vi "DOE Washer SM.vi"() -> ()   [LabVIEW 2018]
uses:
  Utility/Custom Pallet Controls/Custom Pallet Timer.ctl
  Type Definitions/DOE Front Panel Meters.ctl
  Utility/Type Definitions/UTILITY Power Data.ctl
  Utility/Standby Power/Type Definitions/Standby Power Main Data.ctl
  Drivers/Omega FMA-1600A Series Gas Flow Meter/Type Definitions/FMA1600A Gas Data.ctl
  Drivers/Omega FMA-1600A Series Gas Flow Meter/Type Definitions/FMA1600A Gas Type.ctl
  Range/Type Definitions/RANGE Meter Selector 1-2.ctl
  Utility/Save File/File Setup (Public)/Type Definition/Save File DOE File Path Control.ctl
  Utility/Save File/File Setup (Public)/Type Definition/Save File DOE Data Save Filepaths.ctl
  Type Definitions/DOE Main Control.ctl
  Type Definitions/DOE Test Fixture Hardware.ctl
  Utility/Type Definitions/UTILITY Power Inputs Control.ctl
  Drivers/IND560 Scale Monitor/Type Definitions/IND560 Configuration.ctl
  Hybrid Water Heater/Type Definitions/HEWH Agilent Cluster.ctl
  Utility/Type Definitions/UTILITY TC Coefficients.ctl
  Drivers/Omega FMA-1600A Series Gas Flow Meter/Type Definitions/FMA1600A COM Ports.ctl
  Configuration/GEA2.ctl
  Type Definitions/DOE Capacity Measurments.ctl
  Utility/Save File/Public/Type Definitions/Save File Washer.ctl
  Utility/Save File/File Setup (Public)/Type Definition/Save File DISH Dishwasher Details.ctl
  <vilib>/Platform/fileVersionInfo.llb/FileVersionInformation.ctl
  Type Definitions/DOE Appliance Common.ctl
  Utility/Custom Pallet Controls/Custom Pallet String.ctl
  Utility/Save File/File Setup (Public)/Type Definition/DPT IMC Data.ctl
  Type Definitions/DOE Dryer Standard.ctl
  Utility/Save File/Public/Type Definitions/Save File Appliance Display.ctl
  Utility/Save File/Public/Type Definitions/Save File Unit Type.ctl
  Utility/Type Definitions/UTILITY Power Analyzer.ctl
  Type Definitions/DOE Dishwasher Events.ctl
  Utility/Save File/File Setup (Public)/Type Definition/Save File DOE Configuration State.ctl
  Utility/Custom Pallet Controls/Custom Pallet DBL.ctl
  Range/Type Definitions/RANGE DAQ Data Four Meters.ctl
  Range/Type Definitions/RANGE DAQ Data.ctl
  Drivers/Omega FMA-1600A Series Gas Flow Meter/Type Definitions/FMA1600A Units String.ctl
  Range/Type Definitions/RANGE GAS Data.ctl
  Range/Type Definitions/RANGE Panel Data.ctl
  Drivers/Chroma 617xx/Type Definition/CHROMA Phase Shift Lines.ctl
  Drivers/Chroma 617xx/Type Definition/CHROMA Voltage Range.ctl
  Drivers/Yokogawa WT500/Type Definitions/WT500 Wiring Control.ctl
  Type Definitions/DOE Dryer NI Card Settings.ctl
  <vilib>/NI/Modbus Library/API/Master/Modbus Master.lvclass
  Refrigeration/RTS/Type Definitions/RTS Room Selector.ctl
  Drivers/Chroma 617xx/Type Definition/CHROMA Phase.ctl
  Drivers/Chroma 617xx/Type Definition/CHROMA Output State.ctl
  <vilib>/Utility/NIReport.llb/NI_report.lvclass
  Utility/Save File/File Setup (Public)/Type Definition/Save File DOE Model Information.ctl
  Utility/GEA2 Commands/Type Definitions/GEA2 Commands Washer logData.ctl
  Utility/Save File/File Setup (Public)/Type Definition/Save File DOE LabView Program.ctl
  Type Definitions/DOE Data Logger Type.ctl
  <vilib>/Utility/error.llb/whitespace.ctl
  Drivers/Omega FMA-1600A Series Gas Flow Meter/Type Definitions/FMA1600A Commands.ctl
  <vilib>/Instr/_visa.llb/VISA Open Access Mode.ctl
  Drivers/Laurel Meter/Type Definitions/Laurel Serial Commands.ctl
  Range/Type Definitions/Range Meter Bank.ctl
  <vilib>/NI/Modbus Library/API/Wrapper/Create TCP Master.vi
  <vilib>/Utility/file.llb/Write Delimited Spreadsheet (string).vi
  Utility/Save File/File Setup.lvlib
  Utility/Save File/Save File.lvlib
  <vilib>/NI/Modbus Library/API/Wrapper/API Main.lvlib
panel:
  out "Hot Water Rate (GPM)":dbl
  in  "Reset":bool
  in  "Main Tab":T1(tab)
  out "Dishwasher Events":T2
  in  "Rinse Button?":bool
  in  "Reset Hot Laurel Meter":bool
  in  "Scan Rate (Seconds)":dbl=1.0
  in  "Final Weight":bool
  in  "Reset Cold Laurel Meter":bool
  in  "Log Data":bool
  out "Cold Total Usage (Gal)":dbl
  in  "Cold Estimated Water Usage (Gallons)":dbl
  out "Hot Total Usage (Gal)":dbl
  in  "Hot Estimated Water Usage (Gallons)":dbl
  in  "Wait for Power Threshold":bool
  in  "Auto-Terminate Prog":bool
  in  "Power Limit (Watts)":dbl=4.0 format="%#_13g"
  in  "Time Limit At Power Limit (Seconds)":dbl=20.0
  out "XY Graph":T3(graph)
  out "Delta X":dbl
  out "Delta Y":dbl
  in  "Pause Graph":bool
  in  "Clear Graph Data":bool
  in  "X-Axis":string(combo)
  in  "Y-Axis-1":string(combo)
  in  "Y-Axis-2":string(combo)
  out "Test Status":string
  out "Save Path":path
  out "Data":string[][](array[string])
  in  "Change Headers":bool
  out "Point File Path":path
  in  "Save Standby Power Data":bool
  in  "Reset Standby Power":bool
  in  "Est. Power (Watts)":dbl
  in  "Use Estimated Standby Power":bool
  in  "X-Axis (Standby)":string(combo)
  in  "Y-Axis (Standby)":string(combo)
  out "XY Graph Standby":cluster{dbl[], dbl[]}(graph)
  in  "Reset Standby Data":bool
  in  "Start Standby Power":bool
  out "Standby Power Data":string[][](array[string])
  in  "Choose Folder":path
  in  "Start/Stop (Wh Integration)":bool=TRUE
  in  "Tare Totalized Flow":bool
  in  "Tare Mass Flow":bool
  in  "Voltage Limit":i32=130
  in  "Power Supply Status":bool
  in  "L1 Voltage":dbl=120.0
  in  "L2 Voltage":dbl=120.0
  out "Chroma Name":string
  in  "Set Parameters":bool
  in  "Frequency":dbl=60.0
  in  "Set Initialization":bool
  in  "Phase Shift Lines":T4
  in  "Phase Shift Angle":i32=180
  in  "Voltage Range":T5=enum."Low (150V)"
  in  "Wiring (0: 1P2W, 1P2W, 1P2W)":T6=1 items=["1P2W, 1P2W, 1P2W", "1P3W, 1P2W", "3P3W, 1P2W", "1P2W, 1P3W", "1P2W, 3P3W", "3P4W", "3V3A"]
  in  "Set Configuration":bool
  in  "Element (0: All)":u16(ring) items=["All", "Element 1", "Element 2", "Element 3", "Sigma"]
  in  "Voltage Range (8: 1000V)":u16(ring)=6 items=["AUTO", "15", "30", "60", "100", "150", "300", "600", "1000", "7.5", "15", "30", "50", "75", "150", "300", "500"]
  in  "Current Range (7: 40A)":u16(ring)=7 items=["AUTO", "500 mA", "1 A", "2 A", "5 A", "10 A", "20 A", "40 A", "S-AUTO", "50 mV", "100 mV", "200 mV", "500 mV", "1 V", "2 V", "5 V", "10 V", "250 mA", "500 mA", "1 A", "2.5 A", "5 A", "10 A", "20 A", "25 mV", "50 mV", "100 mV", "250 mV", "500 mV", "1 V", "2.5 V", "5 V"]
  in  "Update Rate (3: 500ms)":u16(ring)=2 items=["-", "100ms", "200ms", "500ms", "1s", "2s", "5s"]
  in  "Crest Factor (0: 3)":u16(ring) items=["3", "6"]
  in  "Display Format":u16(ring) items=["Numeric", "Wave", "Bar", "Vector", "Trend"]
  in  "Reset Power Meter":bool
  in  "Condition Name In Column":string="RINSE"
  in  "Column Name":string="Sub-Cycle"
  in  "Use Auto-Rinse Detect":bool
  in  "Start Reading":bool
  in  "File Path To Read":path
  out "Voltage":dbl
  out "Power (Watts)":dbl
  out "Cold Water Pressure (PSIG)":dbl
  out "Hot Water Pressure (PSIG)":dbl
  out "Hot Water Total (Gallons)":dbl
  out "Cold Water Total (Gallons)":dbl
  out "Room Temperature":dbl
  out "Water Temperature (°F)":dbl
  in  "Heating Value (BTU/ft³)":dbl=990.0
  in  "Dryer Pre-Condition":bool
  out "Cold Dryer Weight (lbs)":dbl
  in  "NI Card Settings":T7={"Disable NI Card 1"=FALSE, "Disable NI Card 2"=TRUE, "Disable NI Card 3"=TRUE, "Disable NI Card 4"=TRUE, "Disable NI Card 5"=TRUE, "Disable NI Card 6"=TRUE, "Disable NI Card 7"=TRUE}
  in  "Update Calibration":bool
  in  "Disable Temp/Humidity":bool
  in  "Disable Power":bool
  in  "Disable Flow Rates":bool
  in  "Disable Scale Data":bool
  in  "Disable Analog Data":bool
  in  "Disable Plot":bool
  in  "Washer Controls Input":T8={"Test Fixture Hardware"={"Power "={"Yokogawa"={"WT210"={"Sample Rate (1: 0.25s)"=1, "A Range (12: 20A)"=12, "V Range (6: 600V)"=4, "Power VISA Yokogawa WT210"="WT210"}, "WT500"={"Power VISA Yokogawa WT500"="WT500", "V Range (8: 1000V)"=6, "I Range (7: 40A)"=7, "Update Rate (3: 500ms)"=2}, "WT310_2"={"Sample Rate (1: 0.25s)"=1, "A Range (12: 20A)"=12, "V Range (6: 600V)"=4, "Power VISA Yokogawa WT310_2"="WT310_2"}, "WT310_3"={"Sample Rate (1: 0.25s)"=1, "A Range (12: 20A)"=12, "V Range (6: 600V)"=4, "Power VISA Yokogawa WT310_3"="WT310_3"}}, "Aplus"={"Aplus IP Address"="192.168.1.101", "Remote Port"=502, "Instrument"="APLUS", "Instr Driver Revision"="1.03.0053"}, "Power Limits"={"Crest Factor"={"Upper Limit"=1.49, "Lower Limit"=1.34}, "Harmonic Content"={"Uthd"=2.0}, "Voltage"={"% Error"=2.0}, "Stability"={"<1 Watt "={"Wattage"=1.0, "Slope (mW/H)"=10.0}, ">1 Watt"={"1%Power/Hour"=1.0}}}, "Nominal Voltage"=120, "Time Limit (s)"=10800.0, "Power Variation Limit (%)"=50.0, "Power Supply"={"Chroma 61605"="CHROMA", "Use Chroma?"=FALSE}}, "Weight Scale"={"Com Options"={"IND560Scale VISA"="IND560", "IP Address"="192.168.1.50", "Remote Port"=502, "Setra Scale VISA"="SETRA", "GSE 350"="GSE350"}, "Select Scale"=""}, "Flow Rates"={"Laurel Cold IP Address"="", "Laurel Hot IP Address"="34972A_2", "Hot Water Laurel VISA"="LaurelMeter_Hot", "Cold Water Laurel VISA"="LaurelMeter_Cold", "Remote Port"=0, "Laurel Communication Type"="", "Meters To Collect (Hot Cold)"="", "HOT Laurel Reference"=refnum, "COLD Laurel Reference"=refnum}, "Analog Data"={"Agilent"={"Agilent 34972_1"="34972A_1", "Agilent 34972_2"="34972A_2", "Agilent 34972_3"="34972A_3", "Agilent 34972_4"="34972A_4", "Agilent 34972_5"="34972A_5", "Agilent 34972_6"="34972A_6", "Agilent Gain"=0.0, "TC Type (K,J,T)"="", "Instrument IDN?"="", "TC Channels-List"="", "Analog Channels-List"="", "Agilent Cluster Array"=[], "TC Channels-List 2"="", "Analog Channels-List 2"=""}, "Yokogawa"={"MW100"="MW100", "Intellifaucet"=FALSE}, "Select Analog"="", "TC Coefficients"={"TC Coefficients 1"=[], "TC Coefficients 2"=[], "TC Coefficients 3"=[], "TC Coefficients 4"=[], "TC Coefficients 5"=[], "TC Coefficients 6"=[], "TC Coefficients 7"=[]}, "NI Tasks (Dryer DOE)"=["TC Temps-Module 1", "TC Temps-Module 2", "TC Temps-Module 3", "TC Temps-Module 4", "TC Temps-Module 5", "Gas and Temp-Module 6", "AC_DC Events-Module 7"], "Laurel Analog"={"Laurel IP (Water Temp)"="", "Laurel IP (Pressure)"=""}}, "ITHX-Temp Humidity"={"IP Address 1"="", "Remote Port"=0, "IP Address 2"="", "IP Address 3"=""}, "Gas Meter COM Ports"={"Gas Meter 1"="COM3", "Gas Meter 2"="COM4", "Gas Meter 3"="COM5", "Gas Meter 4"="COM6", "Gas Meter 5"="COM7", "Gas Meter 6"="COM8"}, "Barometric Pressure"={"HEISE 901A"="HEISE", "Use Barometer?"=FALSE}}, "GEA2"={"Address"=35, "Source"=228, "Viper/Hawk"=0}, "DOE Capacity Measurments"={"Weight 1"=35.0, "Model Number 1"="", "Temp 1"=0.0, "Serial Number 1"="", "Lab Number 1"="", "Lab Number 2"="", "Serial Number 2"="", "Temp 2"=0.0, "Model Number 2"="", "Weight 2"=0.0, "Lab Number 3"="", "Serial Number 3"="", "Temp 3"=0.0, "Model Number 3"="", "Weight 3"=0.0, "Lab Number 4"="", "Serial Number 4"="", "Temp 4"=0.0, "Model Number 4"="", "Weight 4"=0.0, "Capacity Measurment Output String"=[]}, "Initialize.Washer In"={"Appliance Details"={"FileVersionInfo"={"FileVersion"="", "ProductName"="", "InternalName"="", "CompanyName"="", "LegalCopyright"="", "FileDescription"=""}, "Dishwasher Info"={"Open Cup Weight (gm):"=0.0, "Auto Cup Weight (gm):"=0.0, "Detergent-Dish:"="", "Inlet Temperature-Dish:"="", "Cycle Mode-Dish:"="", "Unit Control-Dish:"="", "Manufacturer-Dish:"=""}, "Washer Info"={"Hot Water Temperature (Fahrenheit):"="", "Cold Water Temperature (Fahrenheit):"="", "Capacity (cu.ft):"=0.0, "Initial Cloth Weight:"=0.0, "Cloth Lot:"=60, "Model Family:"="", "Program Name:"="", "Cycle Selection:"="", "Wash Temperature:"="", "Rinse Temperature:"="", "Load Size:"=""}, "File Name Output Array"=[], "Calibration Output Array"=[], "Appliance Common"={"Engineer:"="", "Model Number:"="", "Serial Number:"="", "Comments:"="", "Station ID:"="", "Technician:"="", "TR Number:"="", "Lab ID:"="", "Voltage:"="", "Water Pressure (PSI):"="", "Test Date:"="", "Computer Name:"="", "IP Address:"="", "Ambient RH:"="", "Frequency:"="", "Build:"="", "Filename:"="", "Test Type:"="", "Load Run #:"=17, "Ambient Temperature (F):"="", "File Path:"=path "", "Cycles Per Year"=0}, "Water Heater"={"Heating Mode:"=""}, "Dryer"={"Heat Setting:"="", "Washer Water Temperature (60 ± 5°F):"=7, "Water Hardness (PPM):"=7, "Dryness Setting:"="", "Dryer Type:"="", "Exhaust:"="", "Drying Cycle:"="", "Load Type:"="", "Nominal Load Weight"="", "Dryer Initial IMC Data"={"Measured IMC (lbs)"=100.0, "Actual Initial RMC (%)"=7.0, "RMC (Desired %)"=5.0, "Bone Dry Wt(lbs)"=60.0, "Tolerance(%)"=0.0, "Actual Final RMC (%)"=7.0, "CEF (lbf/kWh)"=0.0, "Minimum Weight (lbf)"=0.0, "Average Weight (lbf)"=0.0, "Maximum Weight (lbf)"=0.0, "Measured IMC In Range?"=FALSE, "Moisture Reduction Factor"=55.5, "Field Use Factor"=1.04, "Empty Dryer Cold Weigth"=0.0, "Energy Standard"=enum."D2-Automatic Dryer", "Weight Cloth (lbs)"=0.0, "Relative Moisture Content (%)"=0.0, "Relative Moisture Content - Avg (%)"=0.0}}}, "Display Data (RLT)"={"Status Color"=0, "Serial Number Display"="", "Cycle Count Display"=0, "Station Label Display"="", "Current Run Start Time Display"=0.0, "Board ID Display"="", "RPM Display"=0, "Current Display"=0.0, "Current Path Display"=path "", "Saving Display"=FALSE, "Unit Type Display"=enum."", "Total Time On Display"=0.0, "UI Button"=FALSE}}} {"Initialize.Washer In"."Display Data (RLT)"."Current Display" format="%.2f"; "Initialize.Washer In"."Display Data (RLT)"."Cycle Count Display" format="%04d"; "Initialize.Washer In"."Appliance Details"."Dryer"."Dryer Initial IMC Data"."Maximum Weight (lbf)" format="%03_6g"; "Initialize.Washer In"."Appliance Details"."Dryer"."Dryer Initial IMC Data"."Average Weight (lbf)" format="%03_6g"; "Initialize.Washer In"."Appliance Details"."Dryer"."Dryer Initial IMC Data"."Minimum Weight (lbf)" format="%03_6g"; "Initialize.Washer In"."Appliance Details"."Dryer"."Dryer Initial IMC Data"."CEF (lbf/kWh)" format="%03_6g"; "Initialize.Washer In"."Appliance Details"."Dryer"."Dryer Initial IMC Data"."Actual Final RMC (%)" format="%03_6g"; "Initialize.Washer In"."Appliance Details"."Dryer"."Dryer Initial IMC Data"."Tolerance(%)" format="%0#_6g"; "Initialize.Washer In"."Appliance Details"."Dryer"."Dryer Initial IMC Data"."Bone Dry Wt(lbs)" format="%03_6g"; "Initialize.Washer In"."Appliance Details"."Dryer"."Dryer Initial IMC Data"."RMC (Desired %)" format="%0#_6g"; "Initialize.Washer In"."Appliance Details"."Dryer"."Dryer Initial IMC Data"."Actual Initial RMC (%)" format="%03_6g"; "Initialize.Washer In"."Appliance Details"."Dryer"."Dryer Initial IMC Data"."Measured IMC (lbs)" format="%0#_6g"; "GEA2"."Address" format="%x"; "GEA2"."Source" format="%x"; "GEA2"."Viper/Hawk" items=["Viper", "Hawk"]; "Test Fixture Hardware"."Power"."Yokogawa"."WT310_3"."V Range (6: 600V)" items=["Auto", "15V", "30V", "60V", "150V", "300V", "600V"]; "Test Fixture Hardware"."Power"."Yokogawa"."WT310_3"."A Range (12: 20A)" items=["Auto", "5mA", "10mA", "20mA", "50mA", "100mA", "200mA", "0.5A", "1A", "2A", "5A", "10A", "20A", "50mV", "100mV", "200mV", "2.5V", "5V", "10V"]; "Test Fixture Hardware"."Power"."Yokogawa"."WT310_3"."Sample Rate (1: 0.25s)" items=["0.1s", "0.25s", "0.5s", "1s", "2s", "5s"]; "Test Fixture Hardware"."Power"."Yokogawa"."WT310_2"."V Range (6: 600V)" items=["Auto", "15V", "30V", "60V", "150V", "300V", "600V"]; "Test Fixture Hardware"."Power"."Yokogawa"."WT310_2"."A Range (12: 20A)" items=["Auto", "5mA", "10mA", "20mA", "50mA", "100mA", "200mA", "0.5A", "1A", "2A", "5A", "10A", "20A", "50mV", "100mV", "200mV", "2.5V", "5V", "10V"]; "Test Fixture Hardware"."Power"."Yokogawa"."WT310_2"."Sample Rate (1: 0.25s)" items=["0.1s", "0.25s", "0.5s", "1s", "2s", "5s"]; "Test Fixture Hardware"."Power"."Yokogawa"."WT500"."Update Rate (3: 500ms)" items=["-", "100ms", "200ms", "500ms", "1s", "2s", "5s"]; "Test Fixture Hardware"."Power"."Yokogawa"."WT500"."I Range (7: 40A)" items=["AUTO", "500 mA", "1 A", "2 A", "5 A", "10 A", "20 A", "40 A", "S-AUTO", "50 mV", "100 mV", "200 mV", "500 mV", "1 V", "2 V", "5 V", "10 V", "250 mA", "500 mA", "1 A", "2.5 A", "5 A", "10 A", "20 A", "25 mV", "50 mV", "100 mV", "250 mV", "500 mV", "1 V", "2.5 V", "5 V"]; "Test Fixture Hardware"."Power"."Yokogawa"."WT500"."V Range (8: 1000V)" items=["AUTO", "15", "30", "60", "100", "150", "300", "600", "1000", "7.5", "15", "30", "50", "75", "150", "300", "500"]; "Test Fixture Hardware"."Power"."Yokogawa"."WT210"."V Range (6: 600V)" items=["Auto", "15V", "30V", "60V", "150V", "300V", "600V"]; "Test Fixture Hardware"."Power"."Yokogawa"."WT210"."A Range (12: 20A)" items=["Auto", "5mA", "10mA", "20mA", "50mA", "100mA", "200mA", "0.5A", "1A", "2A", "5A", "10A", "20A", "50mV", "100mV", "200mV", "2.5V", "5V", "10V"]; "Test Fixture Hardware"."Power"."Yokogawa"."WT210"."Sample Rate (1: 0.25s)" items=["0.1s", "0.25s", "0.5s", "1s", "2s", "5s"]}
  out "Max File Size":dbl
  out "Station Name (Specific)":string="Parametric Stand"
  out "Dishwasher Events Visible":bool
  out "Fixture Hardware":T9={"Power "={"Yokogawa"={"WT210"={"Sample Rate (1: 0.25s)"=1, "A Range (12: 20A)"=11, "V Range (6: 600V)"=4, "Power VISA Yokogawa WT210"=""}, "WT500"={"Power VISA Yokogawa WT500"="", "V Range (8: 1000V)"=6, "I Range (7: 40A)"=7, "Update Rate (3: 500ms)"=2}, "WT310_2"={"Sample Rate (1: 0.25s)"=1, "A Range (12: 20A)"=11, "V Range (6: 600V)"=4, "Power VISA Yokogawa WT310_2"=""}, "WT310_3"={"Sample Rate (1: 0.25s)"=1, "A Range (12: 20A)"=11, "V Range (6: 600V)"=4, "Power VISA Yokogawa WT310_3"=""}}, "Aplus"={"Aplus IP Address"="192.168.1.101", "Remote Port"=502, "Instrument"="APLUS", "Instr Driver Revision"="1.03.0053"}, "Power Limits"={"Crest Factor"={"Upper Limit"=1.49, "Lower Limit"=1.34}, "Harmonic Content"={"Uthd"=2.0}, "Voltage"={"% Error"=2.0}, "Stability"={"<1 Watt "={"Wattage"=1.0, "Slope (mW/H)"=10.0}, ">1 Watt"={"1%Power/Hour"=1.0}}}, "Nominal Voltage"=120, "Time Limit (s)"=10800.0, "Power Variation Limit (%)"=50.0, "Power Supply"={"Chroma 61605"="CHROMA", "Use Chroma?"=FALSE}}, "Weight Scale"={"Com Options"={"IND560Scale VISA"="MW100", "IP Address"="", "Remote Port"=0, "Setra Scale VISA"="MW100", "GSE 350"="GSE350"}, "Select Scale"=""}, "Flow Rates"={"Laurel Cold IP Address"="", "Laurel Hot IP Address"="", "Hot Water Laurel VISA"="LaurelMeter_Cold", "Cold Water Laurel VISA"="MW100", "Remote Port"=0, "Laurel Communication Type"="", "Meters To Collect (Hot Cold)"="", "HOT Laurel Reference"=refnum, "COLD Laurel Reference"=refnum}, "Analog Data"={"Agilent"={"Agilent 34972_1"="34972A_3", "Agilent 34972_2"="34972A_2", "Agilent 34972_3"="34972A_3", "Agilent 34972_4"="34972A_3", "Agilent 34972_5"="34972A_3", "Agilent 34972_6"="34972A_3", "Agilent Gain"=0.0, "TC Type (K,J,T)"="", "Instrument IDN?"="", "TC Channels-List"="", "Analog Channels-List"="", "Agilent Cluster Array"=[], "TC Channels-List 2"="", "Analog Channels-List 2"=""}, "Yokogawa"={"MW100"="MW100", "Intellifaucet"=FALSE}, "Select Analog"="", "TC Coefficients"={"TC Coefficients 1"=[], "TC Coefficients 2"=[], "TC Coefficients 3"=[], "TC Coefficients 4"=[], "TC Coefficients 5"=[], "TC Coefficients 6"=[], "TC Coefficients 7"=[]}, "NI Tasks (Dryer DOE)"=["TC Temps-Module 1", "TC Temps-Module 2", "TC Temps-Module 3", "TC Temps-Module 4", "TC Temps-Module 5", "Gas and Temp-Module 6", "AC_DC Events-Module 7"], "Laurel Analog"={"Laurel IP (Water Temp)"="", "Laurel IP (Pressure)"=""}}, "ITHX-Temp Humidity"={"IP Address 1"="", "Remote Port"=0, "IP Address 2"="", "IP Address 3"=""}, "Gas Meter COM Ports"={"Gas Meter 1"="COM3", "Gas Meter 2"="COM4", "Gas Meter 3"="COM5", "Gas Meter 4"="COM6", "Gas Meter 5"="COM7", "Gas Meter 6"="COM8"}, "Barometric Pressure"={"HEISE 901A"="HEISE", "Use Barometer?"=FALSE}} {"Power"."Yokogawa"."WT310_3"."V Range (6: 600V)" items=["Auto", "15V", "30V", "60V", "150V", "300V", "600V"]; "Power"."Yokogawa"."WT310_3"."A Range (12: 20A)" items=["Auto", "5mA", "10mA", "20mA", "50mA", "100mA", "200mA", "0.5A", "1A", "2A", "5A", "10A", "20A", "50mV", "100mV", "200mV", "2.5V", "5V", "10V"]; "Power"."Yokogawa"."WT310_3"."Sample Rate (1: 0.25s)" items=["0.1s", "0.25s", "0.5s", "1s", "2s", "5s"]; "Power"."Yokogawa"."WT310_2"."V Range (6: 600V)" items=["Auto", "15V", "30V", "60V", "150V", "300V", "600V"]; "Power"."Yokogawa"."WT310_2"."A Range (12: 20A)" items=["Auto", "5mA", "10mA", "20mA", "50mA", "100mA", "200mA", "0.5A", "1A", "2A", "5A", "10A", "20A", "50mV", "100mV", "200mV", "2.5V", "5V", "10V"]; "Power"."Yokogawa"."WT310_2"."Sample Rate (1: 0.25s)" items=["0.1s", "0.25s", "0.5s", "1s", "2s", "5s"]; "Power"."Yokogawa"."WT500"."Update Rate (3: 500ms)" items=["-", "100ms", "200ms", "500ms", "1s", "2s", "5s"]; "Power"."Yokogawa"."WT500"."I Range (7: 40A)" items=["AUTO", "500 mA", "1 A", "2 A", "5 A", "10 A", "20 A", "40 A", "S-AUTO", "50 mV", "100 mV", "200 mV", "500 mV", "1 V", "2 V", "5 V", "10 V", "250 mA", "500 mA", "1 A", "2.5 A", "5 A", "10 A", "20 A", "25 mV", "50 mV", "100 mV", "250 mV", "500 mV", "1 V", "2.5 V", "5 V"]; "Power"."Yokogawa"."WT500"."V Range (8: 1000V)" items=["AUTO", "15", "30", "60", "100", "150", "300", "600", "1000", "7.5", "15", "30", "50", "75", "150", "300", "500"]; "Power"."Yokogawa"."WT210"."V Range (6: 600V)" items=["Auto", "15V", "30V", "60V", "150V", "300V", "600V"]; "Power"."Yokogawa"."WT210"."A Range (12: 20A)" items=["Auto", "5mA", "10mA", "20mA", "50mA", "100mA", "200mA", "0.5A", "1A", "2A", "5A", "10A", "20A", "50mV", "100mV", "200mV", "2.5V", "5V", "10V"]; "Power"."Yokogawa"."WT210"."Sample Rate (1: 0.25s)" items=["0.1s", "0.25s", "0.5s", "1s", "2s", "5s"]}
  out "Header Data":string[][](array[string])
  out "Measurments Output":T26={"Power Measurements"={"Current (A):Element 1"=0.0, "Current (A):Element 2"=0.0, "Power (W):Sigma"=0.0, "Watt Hours (Wh):Sigma"=0.0, "Voltage (V):Element 2"=0.0, "Voltage (V):Element 1"=0.0, "Current Crest Factor:Element 1"=0.0, "Current Crest Factor:Element 2"=0.0, "Voltage Harmonic (%):Element 1"=0.0, "Voltage Harmonic (%):Element 2"=0.0, "Voltage Crest Factor:Element 1"=0.0, "Voltage Crest Factor:Element 2"=0.0, "Time:Element 1"=0.0, "Frequency (Hz):Element 1"=0.0, "Apparent Power (VA):Element 1"=0.0, "Apparent Power (VA):Element 2"=0.0, "Power Factor:Element 1"=0.0, "Power Factor:Element 2"=0.0, "Max Watt Hours"=0.0, "Voltage (V):Element 2 Avg"=0.0, "Voltage (V):Element 1 Avg"=0.0}, "Standby Power"={"Standby Power Spreadsheet"=[], "Standby Power - Pia (Watts)"=0.0, "Off Mode Power - Poff (Watts)"=0.0, "Sia hr/yr"=8620.0, "Soff hr/yr"=0.0, "Yearly Energy Etso kWh/yr"=0.0, "Maximum Power (Watts)"=0.0, "Power Variation (%)"=0.0, "Slope (mW/hr)"=0.0, "Final Harmonics-U1 (%)"="", "Final Harmonics-U2 (%)"="", "Energy (Wh)"=0.0}, "Washer"={"Washer String Data"=[], "Analog Scale Weight (lbs)"=0.0}, "Dishwasher"={"Drain Solonoid Event"=0, "Pump Event"=0, "Water Valve Event"=0, "Heater Event"=0, "Motor Event"=0, "Turbidity Sensor"=0.0, "Spare 2"=0.0, "Spare 3"=0.0, "Spare 4"=0.0, "Spare 5"=0.0, "Thermocouple 1"=0.0, "Thermocouple 2"=0.0, "Thermocouple 3"=0.0, "Thermocouple 4"=0.0, "Thermocouple 5"=0.0, "Thermocouple 6"=0.0, "Spare 1"=0.0, "Dishwasher String Data"=[]}, "Washer HCC"={"Chan 101"=0.0, "Chan 102"=0.0, "Chan 103"=0.0, "Chan 104"=0.0, "Chan 105"=0.0, "Chan 106"=0.0, "Chan 107"=0.0, "Chan 108"=0.0, "Chan 109"=0.0, "Chan 110"=0.0, "Chan 111"=0.0, "Chan 112"=0.0, "Chan 113"=0.0, "Chan 114"=0.0, "Chan 115"=0.0, "Chan 116"=0.0, "Chan 117"=0.0, "Chan 118"=0.0, "Chan 119"=0.0, "Chan 120"=0.0, "Chan 201"=0.0, "Chan 202"=0.0, "Chan 203"=0.0, "Chan 204"=0.0, "Chan 205"=0.0, "Chan 206"=0.0, "Chan 207"=0.0, "Chan 208"=0.0, "Chan 209"=0.0, "Chan 210"=0.0, "Chan 211"=0.0, "Chan 212"=0.0, "Chan 213"=0.0, "Chan 214"=0.0, "Chan 215"=0.0, "Chan 216"=0.0, "Chan 217"=0.0, "Chan 218"=0.0, "Chan 219"=0.0, "Chan 220"=0.0, "Chan 301"=0.0, "Chan 302"=0.0, "Chan 303"=0.0, "Chan 304"=0.0, "Chan 305"=0.0, "Chan 306"=0.0, "Chan 307"=0.0, "Chan 308"=0.0, "Chan 309"=0.0, "Chan 310"=0.0, "Chan 311"=0.0, "Chan 312"=0.0, "Chan 313"=0.0, "Chan 314"=0.0, "Chan 315"=0.0, "Chan 316"=0.0, "Chan 317"=0.0, "Chan 318"=0.0, "Chan 319"=0.0, "Chan 320"=0.0}, "Barometric Pressure"={"Barometric Pressure (in. Hg)"=0.0}, "Ambient Conditions"={"Ambient Temperature  1 (°F)"=0.0, "Ambient Temperature 2 (°F)"=0.0, "Ambient Temperature 3 (°F)"=0.0, "Ambient Humidity 1 (%)"=0.0, "Ambient Humidity 2 (%)"=0.0, "Ambient Humidity 3 (%)"=0.0, "Ambient Dewpoint  1 (°F)"=0.0, "Ambient Dewpoint 2 (°F)"=0.0, "Ambient Dewpoint 3 (°F)"=0.0}, "Weight Scale"={"Gross Weigth (lbs)"=0.0, "Net Weight (lbs)"=0.0, "Final Weight (lbs)"=""}, "Water Measurements"={"Hot Water Pressure (psi)"=0.0, "Hot Water Pressure Max (psi)"=0.0, "Hot Water Temperature (°F)"=0.0, "Cold Water Pressure (psi)"=0.0, "Cold Water Pressure Max (psi)"=0.0, "Hot Water Temperature Max (°F)"=0.0, "Cold Water Temperature (°F)"=0.0, "Cold Water Temperature Max (°F)"=0.0, "Hot Water Total (Gal)"=0.0, "Hot Water Rate (GPM)"=0.0, "Cold Water Total (Gal)"=0.0, "Cold Water Rate (GPM)"=0.0, "Cold Water Total During Wash (Gal)"=0.0, "Hot Water Total During Wash (Gal)"=0.0, "Rinse Cold (Gal)"=0.0, "Rinse Hot (Gal)"=0.0, "Hot Water Pressure Min (psi)"=0.0, "Hot Water Temperature Min (°F)"=0.0, "Cold Water Pressure Min (psi)"=0.0, "Cold Water Temperature Min (°F)"=0.0}, "Gas Data"={"Meter Type (Gas)"="", "Meter ID"=enum."Disabled", "Heating Value (BTU/ft³)"=0.0, "Ft³ / Hr (SCFH)"=0.0, "15 Second Average (BTU/HR)"=0.0, "30 Second Average (BTU/HR)"=0.0, "SLPM (Mass Flow)"=0.0, "LPM (Vol. Flow)"=0.0, "Gas Temperature (°F)"=0.0, "Gas Pressure (PSIA)"=0.0, "Tot.Flow (Liters)"=0.0}} {"Power Measurements"."Voltage (V):Element 1 Avg" format="%.3g"; "Power Measurements"."Voltage (V):Element 2 Avg" format="%.3g"; "Power Measurements"."Max Watt Hours" format="%.3g"; "Power Measurements"."Power Factor:Element 2" format="%.3g"; "Power Measurements"."Power Factor:Element 1" format="%.3g"; "Power Measurements"."Apparent Power (VA):Element 2" format="%.3g"; "Power Measurements"."Apparent Power (VA):Element 1" format="%.3g"; "Power Measurements"."Frequency (Hz):Element 1" format="%.3g"; "Power Measurements"."Time:Element 1" format="%.3g"; "Power Measurements"."Voltage Crest Factor:Element 2" format="%.3g"; "Power Measurements"."Voltage Crest Factor:Element 1" format="%.3g"; "Power Measurements"."Voltage Harmonic (%):Element 2" format="%.3g"; "Power Measurements"."Voltage Harmonic (%):Element 1" format="%.3g"; "Power Measurements"."Current Crest Factor:Element 2" format="%.3g"; "Power Measurements"."Current Crest Factor:Element 1" format="%.3g"; "Power Measurements"."Voltage (V):Element 1" format="%.3g"; "Power Measurements"."Voltage (V):Element 2" format="%.3g"; "Power Measurements"."Watt Hours (Wh):Sigma" format="%.3f"; "Power Measurements"."Power (W):Sigma" format="%.3g"; "Power Measurements"."Current (A):Element 2" format="%.3g"; "Power Measurements"."Current (A):Element 1" format="%.3g"}
  out "Measurments 2":T26={"Power Measurements"={"Current (A):Element 1"=0.0, "Current (A):Element 2"=0.0, "Power (W):Sigma"=0.0, "Watt Hours (Wh):Sigma"=0.0, "Voltage (V):Element 2"=0.0, "Voltage (V):Element 1"=0.0, "Current Crest Factor:Element 1"=0.0, "Current Crest Factor:Element 2"=0.0, "Voltage Harmonic (%):Element 1"=0.0, "Voltage Harmonic (%):Element 2"=0.0, "Voltage Crest Factor:Element 1"=0.0, "Voltage Crest Factor:Element 2"=0.0, "Time:Element 1"=0.0, "Frequency (Hz):Element 1"=0.0, "Apparent Power (VA):Element 1"=0.0, "Apparent Power (VA):Element 2"=0.0, "Power Factor:Element 1"=0.0, "Power Factor:Element 2"=0.0, "Max Watt Hours"=0.0, "Voltage (V):Element 2 Avg"=0.0, "Voltage (V):Element 1 Avg"=0.0}, "Standby Power"={"Standby Power Spreadsheet"=[], "Standby Power - Pia (Watts)"=0.0, "Off Mode Power - Poff (Watts)"=0.0, "Sia hr/yr"=8620.0, "Soff hr/yr"=0.0, "Yearly Energy Etso kWh/yr"=0.0, "Maximum Power (Watts)"=0.0, "Power Variation (%)"=0.0, "Slope (mW/hr)"=0.0, "Final Harmonics-U1 (%)"="", "Final Harmonics-U2 (%)"="", "Energy (Wh)"=0.0}, "Washer"={"Washer String Data"=[], "Analog Scale Weight (lbs)"=0.0}, "Dishwasher"={"Drain Solonoid Event"=0, "Pump Event"=0, "Water Valve Event"=0, "Heater Event"=0, "Motor Event"=0, "Turbidity Sensor"=0.0, "Spare 2"=0.0, "Spare 3"=0.0, "Spare 4"=0.0, "Spare 5"=0.0, "Thermocouple 1"=0.0, "Thermocouple 2"=0.0, "Thermocouple 3"=0.0, "Thermocouple 4"=0.0, "Thermocouple 5"=0.0, "Thermocouple 6"=0.0, "Spare 1"=0.0, "Dishwasher String Data"=[]}, "Washer HCC"={"Chan 101"=0.0, "Chan 102"=0.0, "Chan 103"=0.0, "Chan 104"=0.0, "Chan 105"=0.0, "Chan 106"=0.0, "Chan 107"=0.0, "Chan 108"=0.0, "Chan 109"=0.0, "Chan 110"=0.0, "Chan 111"=0.0, "Chan 112"=0.0, "Chan 113"=0.0, "Chan 114"=0.0, "Chan 115"=0.0, "Chan 116"=0.0, "Chan 117"=0.0, "Chan 118"=0.0, "Chan 119"=0.0, "Chan 120"=0.0, "Chan 201"=0.0, "Chan 202"=0.0, "Chan 203"=0.0, "Chan 204"=0.0, "Chan 205"=0.0, "Chan 206"=0.0, "Chan 207"=0.0, "Chan 208"=0.0, "Chan 209"=0.0, "Chan 210"=0.0, "Chan 211"=0.0, "Chan 212"=0.0, "Chan 213"=0.0, "Chan 214"=0.0, "Chan 215"=0.0, "Chan 216"=0.0, "Chan 217"=0.0, "Chan 218"=0.0, "Chan 219"=0.0, "Chan 220"=0.0, "Chan 301"=0.0, "Chan 302"=0.0, "Chan 303"=0.0, "Chan 304"=0.0, "Chan 305"=0.0, "Chan 306"=0.0, "Chan 307"=0.0, "Chan 308"=0.0, "Chan 309"=0.0, "Chan 310"=0.0, "Chan 311"=0.0, "Chan 312"=0.0, "Chan 313"=0.0, "Chan 314"=0.0, "Chan 315"=0.0, "Chan 316"=0.0, "Chan 317"=0.0, "Chan 318"=0.0, "Chan 319"=0.0, "Chan 320"=0.0}, "Barometric Pressure"={"Barometric Pressure (in. Hg)"=0.0}, "Ambient Conditions"={"Ambient Temperature  1 (°F)"=0.0, "Ambient Temperature 2 (°F)"=0.0, "Ambient Temperature 3 (°F)"=0.0, "Ambient Humidity 1 (%)"=0.0, "Ambient Humidity 2 (%)"=0.0, "Ambient Humidity 3 (%)"=0.0, "Ambient Dewpoint  1 (°F)"=0.0, "Ambient Dewpoint 2 (°F)"=0.0, "Ambient Dewpoint 3 (°F)"=0.0}, "Weight Scale"={"Gross Weigth (lbs)"=0.0, "Net Weight (lbs)"=0.0, "Final Weight (lbs)"=""}, "Water Measurements"={"Hot Water Pressure (psi)"=0.0, "Hot Water Pressure Max (psi)"=0.0, "Hot Water Temperature (°F)"=0.0, "Cold Water Pressure (psi)"=0.0, "Cold Water Pressure Max (psi)"=0.0, "Hot Water Temperature Max (°F)"=0.0, "Cold Water Temperature (°F)"=0.0, "Cold Water Temperature Max (°F)"=0.0, "Hot Water Total (Gal)"=0.0, "Hot Water Rate (GPM)"=0.0, "Cold Water Total (Gal)"=0.0, "Cold Water Rate (GPM)"=0.0, "Cold Water Total During Wash (Gal)"=0.0, "Hot Water Total During Wash (Gal)"=0.0, "Rinse Cold (Gal)"=0.0, "Rinse Hot (Gal)"=0.0, "Hot Water Pressure Min (psi)"=0.0, "Hot Water Temperature Min (°F)"=0.0, "Cold Water Pressure Min (psi)"=0.0, "Cold Water Temperature Min (°F)"=0.0}, "Gas Data"={"Meter Type (Gas)"="", "Meter ID"=enum."Disabled", "Heating Value (BTU/ft³)"=0.0, "Ft³ / Hr (SCFH)"=0.0, "15 Second Average (BTU/HR)"=0.0, "30 Second Average (BTU/HR)"=0.0, "SLPM (Mass Flow)"=0.0, "LPM (Vol. Flow)"=0.0, "Gas Temperature (°F)"=0.0, "Gas Pressure (PSIA)"=0.0, "Tot.Flow (Liters)"=0.0}} {"Power Measurements"."Voltage (V):Element 1 Avg" format="%.3g"; "Power Measurements"."Voltage (V):Element 2 Avg" format="%.3g"; "Power Measurements"."Max Watt Hours" format="%.3g"; "Power Measurements"."Power Factor:Element 2" format="%.3g"; "Power Measurements"."Power Factor:Element 1" format="%.3g"; "Power Measurements"."Apparent Power (VA):Element 2" format="%.3g"; "Power Measurements"."Apparent Power (VA):Element 1" format="%.3g"; "Power Measurements"."Frequency (Hz):Element 1" format="%.3g"; "Power Measurements"."Time:Element 1" format="%.3g"; "Power Measurements"."Voltage Crest Factor:Element 2" format="%.3g"; "Power Measurements"."Voltage Crest Factor:Element 1" format="%.3g"; "Power Measurements"."Voltage Harmonic (%):Element 2" format="%.3g"; "Power Measurements"."Voltage Harmonic (%):Element 1" format="%.3g"; "Power Measurements"."Current Crest Factor:Element 2" format="%.3g"; "Power Measurements"."Current Crest Factor:Element 1" format="%.3g"; "Power Measurements"."Voltage (V):Element 1" format="%.3g"; "Power Measurements"."Voltage (V):Element 2" format="%.3g"; "Power Measurements"."Watt Hours (Wh):Sigma" format="%.3f"; "Power Measurements"."Power (W):Sigma" format="%.3g"; "Power Measurements"."Current (A):Element 2" format="%.3g"; "Power Measurements"."Current (A):Element 1" format="%.3g"}
  out "Save Data":string[][](array[string])
  out "Start DAQ":bool
  in  "Config State":T32
  out "File  Version":string="Parametric Stand"
  out "Standard GEA2":string[][](array[string])
  out "Front Program Name":string="Parametric Stand"
  out "Elapsed Time":T33 format="%<%H:%M:%S>t"
  in  "Configuration Tab":T34(tab)
  out "Start Flow Rate Loop":bool
  out "Test State":string[](array[string])
  in  "Debug Main":bool
  out "Flow Rate Loop":i32
  out "Write Header":bool
  out "Config Path with Tool Base":path
  in  "Disable Digital":bool
  out "Folder Path":path
  out "Plot Array":dbl[][](array[numeric])
  out "Main Start":dbl format="%.2f"
  out "Main Loop Rate":dbl format="%0.2f"
  out "Scale Loop":i32
  out "Main Loop Rate 2":T35 format="%.2f"
  out "Rate":dbl format="%0.2f"
  in  "K(0.3)":dbl=0.3 format="%#_13g"
  out "Main Loop":i32
  in  "Initialize Rate":bool
  out "Laurel SM":string[](array[string])
  in  "Debug Laurel":bool
  out "Laurel State":string
  out "Main State":string
  out "Stop Scale Loop":bool=TRUE
  out "Main Exit":bool=TRUE
  in  "Enable RMC Collection":bool
  in  "Manual Range (20 <10> A)":dbl(ring)=10.0 items=["5m <2.5m>"=0.0025, "10m <5m>"=0.005, "20m <10m>"=0.01, "50m <25m>"=0.025, "100m <50m>"=0.05, "200m <100m>"=0.1, "500m <250m>"=0.25, "1 <500m>"=0.5, "2 <1>"=1.0, "5 <2.5>"=2.5, "10 <5>"=5.0, "20 <10>"=10.0, "40 <20>"=20.0]
  out "Water Temperature":dbl
  out "Water Pressure":dbl
  in  "Hardware Tab":T36(tab)
  out "Washer Controls":T8={"Test Fixture Hardware"={"Power "={"Yokogawa"={"WT210"={"Sample Rate (1: 0.25s)"=1, "A Range (12: 20A)"=12, "V Range (6: 600V)"=4, "Power VISA Yokogawa WT210"="WT210"}, "WT500"={"Power VISA Yokogawa WT500"="WT500", "V Range (8: 1000V)"=0, "I Range (7: 40A)"=0, "Update Rate (3: 500ms)"=2}, "WT310_2"={"Sample Rate (1: 0.25s)"=1, "A Range (12: 20A)"=11, "V Range (6: 600V)"=4, "Power VISA Yokogawa WT310_2"="WT310_2"}, "WT310_3"={"Sample Rate (1: 0.25s)"=1, "A Range (12: 20A)"=11, "V Range (6: 600V)"=4, "Power VISA Yokogawa WT310_3"="WT310_3"}}, "Aplus"={"Aplus IP Address"="192.168.1.101", "Remote Port"=502, "Instrument"="APLUS", "Instr Driver Revision"="1.03.0053"}, "Power Limits"={"Crest Factor"={"Upper Limit"=1.49, "Lower Limit"=1.34}, "Harmonic Content"={"Uthd"=2.0}, "Voltage"={"% Error"=2.0}, "Stability"={"<1 Watt "={"Wattage"=1.0, "Slope (mW/H)"=10.0}, ">1 Watt"={"1%Power/Hour"=1.0}}}, "Nominal Voltage"=120, "Time Limit (s)"=10800.0, "Power Variation Limit (%)"=50.0, "Power Supply"={"Chroma 61605"="CHROMA", "Use Chroma?"=FALSE}}, "Weight Scale"={"Com Options"={"IND560Scale VISA"="IND560", "IP Address"="192.168.1.50", "Remote Port"=502, "Setra Scale VISA"="SETRA", "GSE 350"="GSE350"}, "Select Scale"=""}, "Flow Rates"={"Laurel Cold IP Address"="", "Laurel Hot IP Address"="34972A_2", "Hot Water Laurel VISA"="LaurelMeter_Hot", "Cold Water Laurel VISA"="LaurelMeter_Cold", "Remote Port"=0, "Laurel Communication Type"="", "Meters To Collect (Hot Cold)"="", "HOT Laurel Reference"=refnum, "COLD Laurel Reference"=refnum}, "Analog Data"={"Agilent"={"Agilent 34972_1"="34972A_1", "Agilent 34972_2"="34972A_2", "Agilent 34972_3"="34972A_3", "Agilent 34972_4"="34972A_4", "Agilent 34972_5"="34972A_5", "Agilent 34972_6"="34972A_6", "Agilent Gain"=0.0, "TC Type (K,J,T)"="", "Instrument IDN?"="", "TC Channels-List"="", "Analog Channels-List"="", "Agilent Cluster Array"=[], "TC Channels-List 2"="", "Analog Channels-List 2"=""}, "Yokogawa"={"MW100"="MW100", "Intellifaucet"=FALSE}, "Select Analog"="", "TC Coefficients"={"TC Coefficients 1"=[], "TC Coefficients 2"=[], "TC Coefficients 3"=[], "TC Coefficients 4"=[], "TC Coefficients 5"=[], "TC Coefficients 6"=[], "TC Coefficients 7"=[]}, "NI Tasks (Dryer DOE)"=["TC Temps-Module 1", "TC Temps-Module 2", "TC Temps-Module 3", "TC Temps-Module 4", "TC Temps-Module 5", "Gas and Temp-Module 6", "AC_DC Events-Module 7"], "Laurel Analog"={"Laurel IP (Water Temp)"="", "Laurel IP (Pressure)"=""}}, "ITHX-Temp Humidity"={"IP Address 1"="", "Remote Port"=0, "IP Address 2"="", "IP Address 3"=""}, "Gas Meter COM Ports"={"Gas Meter 1"="COM3", "Gas Meter 2"="COM4", "Gas Meter 3"="COM5", "Gas Meter 4"="COM6", "Gas Meter 5"="COM7", "Gas Meter 6"="COM8"}, "Barometric Pressure"={"HEISE 901A"="HEISE", "Use Barometer?"=FALSE}}, "GEA2"={"Address"=35, "Source"=228, "Viper/Hawk"=0}, "DOE Capacity Measurments"={"Weight 1"=35.0, "Model Number 1"="", "Temp 1"=0.0, "Serial Number 1"="", "Lab Number 1"="", "Lab Number 2"="", "Serial Number 2"="", "Temp 2"=0.0, "Model Number 2"="", "Weight 2"=0.0, "Lab Number 3"="", "Serial Number 3"="", "Temp 3"=0.0, "Model Number 3"="", "Weight 3"=0.0, "Lab Number 4"="", "Serial Number 4"="", "Temp 4"=0.0, "Model Number 4"="", "Weight 4"=0.0, "Capacity Measurment Output String"=[]}, "Initialize.Washer In"={"Appliance Details"={"FileVersionInfo"={"FileVersion"="", "ProductName"="", "InternalName"="", "CompanyName"="", "LegalCopyright"="", "FileDescription"=""}, "Dishwasher Info"={"Open Cup Weight (gm):"=0.0, "Auto Cup Weight (gm):"=0.0, "Detergent-Dish:"="", "Inlet Temperature-Dish:"="", "Cycle Mode-Dish:"="", "Unit Control-Dish:"="", "Manufacturer-Dish:"=""}, "Washer Info"={"Hot Water Temperature (Fahrenheit):"="", "Cold Water Temperature (Fahrenheit):"="", "Capacity (cu.ft):"=0.0, "Initial Cloth Weight:"=0.0, "Cloth Lot:"=60, "Model Family:"="", "Program Name:"="", "Cycle Selection:"="", "Wash Temperature:"="", "Rinse Temperature:"="", "Load Size:"=""}, "File Name Output Array"=[], "Calibration Output Array"=[], "Appliance Common"={"Engineer:"="", "Model Number:"="", "Serial Number:"="", "Comments:"="", "Station ID:"="", "Technician:"="", "TR Number:"="", "Lab ID:"="", "Voltage:"="", "Water Pressure (PSI):"="", "Test Date:"="", "Computer Name:"="", "IP Address:"="", "Ambient RH:"="", "Frequency:"="", "Build:"="", "Filename:"="", "Test Type:"="", "Load Run #:"=17, "Ambient Temperature (F):"="", "File Path:"=path "", "Cycles Per Year"=0}, "Water Heater"={"Heating Mode:"=""}, "Dryer"={"Heat Setting:"="", "Washer Water Temperature (60 ± 5°F):"=7, "Water Hardness (PPM):"=7, "Dryness Setting:"="", "Dryer Type:"="", "Exhaust:"="", "Drying Cycle:"="", "Load Type:"="", "Nominal Load Weight"="", "Dryer Initial IMC Data"={"Measured IMC (lbs)"=100.0, "Actual Initial RMC (%)"=7.0, "RMC (Desired %)"=5.0, "Bone Dry Wt(lbs)"=60.0, "Tolerance(%)"=0.0, "Actual Final RMC (%)"=7.0, "CEF (lbf/kWh)"=0.0, "Minimum Weight (lbf)"=0.0, "Average Weight (lbf)"=0.0, "Maximum Weight (lbf)"=0.0, "Measured IMC In Range?"=FALSE, "Moisture Reduction Factor"=55.5, "Field Use Factor"=1.04, "Empty Dryer Cold Weigth"=0.0, "Energy Standard"=enum."D2-Automatic Dryer", "Weight Cloth (lbs)"=0.0, "Relative Moisture Content (%)"=0.0, "Relative Moisture Content - Avg (%)"=0.0}}}, "Display Data (RLT)"={"Status Color"=0, "Serial Number Display"="", "Cycle Count Display"=0, "Station Label Display"="", "Current Run Start Time Display"=0.0, "Board ID Display"="", "RPM Display"=0, "Current Display"=0.0, "Current Path Display"=path "", "Saving Display"=FALSE, "Unit Type Display"=enum."", "Total Time On Display"=0.0, "UI Button"=FALSE}}} {"Initialize.Washer In"."Display Data (RLT)"."Current Display" format="%.2f"; "Initialize.Washer In"."Display Data (RLT)"."Cycle Count Display" format="%04d"; "Initialize.Washer In"."Appliance Details"."Dryer"."Dryer Initial IMC Data"."Maximum Weight (lbf)" format="%03_6g"; "Initialize.Washer In"."Appliance Details"."Dryer"."Dryer Initial IMC Data"."Average Weight (lbf)" format="%03_6g"; "Initialize.Washer In"."Appliance Details"."Dryer"."Dryer Initial IMC Data"."Minimum Weight (lbf)" format="%03_6g"; "Initialize.Washer In"."Appliance Details"."Dryer"."Dryer Initial IMC Data"."CEF (lbf/kWh)" format="%03_6g"; "Initialize.Washer In"."Appliance Details"."Dryer"."Dryer Initial IMC Data"."Actual Final RMC (%)" format="%03_6g"; "Initialize.Washer In"."Appliance Details"."Dryer"."Dryer Initial IMC Data"."Tolerance(%)" format="%0#_6g"; "Initialize.Washer In"."Appliance Details"."Dryer"."Dryer Initial IMC Data"."Bone Dry Wt(lbs)" format="%03_6g"; "Initialize.Washer In"."Appliance Details"."Dryer"."Dryer Initial IMC Data"."RMC (Desired %)" format="%0#_6g"; "Initialize.Washer In"."Appliance Details"."Dryer"."Dryer Initial IMC Data"."Actual Initial RMC (%)" format="%03_6g"; "Initialize.Washer In"."Appliance Details"."Dryer"."Dryer Initial IMC Data"."Measured IMC (lbs)" format="%0#_6g"; "GEA2"."Address" format="%x"; "GEA2"."Source" format="%x"; "GEA2"."Viper/Hawk" items=["Viper", "Hawk"]; "Test Fixture Hardware"."Power"."Yokogawa"."WT310_3"."V Range (6: 600V)" items=["Auto", "15V", "30V", "60V", "150V", "300V", "600V"]; "Test Fixture Hardware"."Power"."Yokogawa"."WT310_3"."A Range (12: 20A)" items=["Auto", "5mA", "10mA", "20mA", "50mA", "100mA", "200mA", "0.5A", "1A", "2A", "5A", "10A", "20A", "50mV", "100mV", "200mV", "2.5V", "5V", "10V"]; "Test Fixture Hardware"."Power"."Yokogawa"."WT310_3"."Sample Rate (1: 0.25s)" items=["0.1s", "0.25s", "0.5s", "1s", "2s", "5s"]; "Test Fixture Hardware"."Power"."Yokogawa"."WT310_2"."V Range (6: 600V)" items=["Auto", "15V", "30V", "60V", "150V", "300V", "600V"]; "Test Fixture Hardware"."Power"."Yokogawa"."WT310_2"."A Range (12: 20A)" items=["Auto", "5mA", "10mA", "20mA", "50mA", "100mA", "200mA", "0.5A", "1A", "2A", "5A", "10A", "20A", "50mV", "100mV", "200mV", "2.5V", "5V", "10V"]; "Test Fixture Hardware"."Power"."Yokogawa"."WT310_2"."Sample Rate (1: 0.25s)" items=["0.1s", "0.25s", "0.5s", "1s", "2s", "5s"]; "Test Fixture Hardware"."Power"."Yokogawa"."WT500"."Update Rate (3: 500ms)" items=["-", "100ms", "200ms", "500ms", "1s", "2s", "5s"]; "Test Fixture Hardware"."Power"."Yokogawa"."WT500"."I Range (7: 40A)" items=["AUTO", "500 mA", "1 A", "2 A", "5 A", "10 A", "20 A", "40 A", "S-AUTO", "50 mV", "100 mV", "200 mV", "500 mV", "1 V", "2 V", "5 V", "10 V", "250 mA", "500 mA", "1 A", "2.5 A", "5 A", "10 A", "20 A", "25 mV", "50 mV", "100 mV", "250 mV", "500 mV", "1 V", "2.5 V", "5 V"]; "Test Fixture Hardware"."Power"."Yokogawa"."WT500"."V Range (8: 1000V)" items=["AUTO", "15", "30", "60", "100", "150", "300", "600", "1000", "7.5", "15", "30", "50", "75", "150", "300", "500"]; "Test Fixture Hardware"."Power"."Yokogawa"."WT210"."V Range (6: 600V)" items=["Auto", "15V", "30V", "60V", "150V", "300V", "600V"]; "Test Fixture Hardware"."Power"."Yokogawa"."WT210"."A Range (12: 20A)" items=["Auto", "5mA", "10mA", "20mA", "50mA", "100mA", "200mA", "0.5A", "1A", "2A", "5A", "10A", "20A", "50mV", "100mV", "200mV", "2.5V", "5V", "10V"]; "Test Fixture Hardware"."Power"."Yokogawa"."WT210"."Sample Rate (1: 0.25s)" items=["0.1s", "0.25s", "0.5s", "1s", "2s", "5s"]}
  out "error out":errorcluster
  in  "error in (no error)":errorcluster
  out "P:Sigma":dbl
  out "Limit Reached":bool
  out "Start Saving Data":bool
  in  "Power Analyzer":T37=enum."APLUS"
  out "Start Time (sec)":dbl format="%<%H:%M:%S>t"
  in  "Filepath":T38
  out "File Name Output Array":string[][](array[string])
  out "Weight Data":string[][](array[string])
  out "DAQ Data Out":T40={"Meter 1"={"Meter Size"=0.0, "DAQ Output (Voltage)"=0.0, "Reference (Voltage)"=0.0, "Meter Present"=FALSE, "Meter Visa"="COM3", "Gas Type"="", "SLPM Error @ Zero"=0.0, "Gas Mix Number"="", "Set STP Register"=FALSE, "Measurement Units"={"Abs. Pressure"="", "Gauge/Diff. Press."="", "Barometric Press."="", "Temperature"="", "Volume"="", "Mass"="", "Setpoint"="", "Valve Drive"="", "Totalizer"="", "Tot. Timer"="", "Tot. Avg. Flow"="", "Tot. Peak Flow"="", "Software Version"=""}}, "Meter 2"={"Meter Size"=0.0, "DAQ Output (Voltage)"=0.0, "Reference (Voltage)"=0.0, "Meter Present"=FALSE, "Meter Visa"="COM3", "Gas Type"="", "SLPM Error @ Zero"=0.0, "Gas Mix Number"="", "Set STP Register"=FALSE, "Measurement Units"={"Abs. Pressure"="", "Gauge/Diff. Press."="", "Barometric Press."="", "Temperature"="", "Volume"="", "Mass"="", "Setpoint"="", "Valve Drive"="", "Totalizer"="", "Tot. Timer"="", "Tot. Avg. Flow"="", "Tot. Peak Flow"="", "Software Version"=""}}, "Meter 3"={"Meter Size"=0.0, "DAQ Output (Voltage)"=0.0, "Reference (Voltage)"=0.0, "Meter Present"=FALSE, "Meter Visa"="COM3", "Gas Type"="", "SLPM Error @ Zero"=0.0, "Gas Mix Number"="", "Set STP Register"=FALSE, "Measurement Units"={"Abs. Pressure"="", "Gauge/Diff. Press."="", "Barometric Press."="", "Temperature"="", "Volume"="", "Mass"="", "Setpoint"="", "Valve Drive"="", "Totalizer"="", "Tot. Timer"="", "Tot. Avg. Flow"="", "Tot. Peak Flow"="", "Software Version"=""}}, "Meter 4"={"Meter Size"=0.0, "DAQ Output (Voltage)"=0.0, "Reference (Voltage)"=0.0, "Meter Present"=FALSE, "Meter Visa"="COM3", "Gas Type"="", "SLPM Error @ Zero"=0.0, "Gas Mix Number"="", "Set STP Register"=FALSE, "Measurement Units"={"Abs. Pressure"="", "Gauge/Diff. Press."="", "Barometric Press."="", "Temperature"="", "Volume"="", "Mass"="", "Setpoint"="", "Valve Drive"="", "Totalizer"="", "Tot. Timer"="", "Tot. Avg. Flow"="", "Tot. Peak Flow"="", "Software Version"=""}}, "Meter 5"={"Meter Size"=0.0, "DAQ Output (Voltage)"=0.0, "Reference (Voltage)"=0.0, "Meter Present"=FALSE, "Meter Visa"="COM3", "Gas Type"="", "SLPM Error @ Zero"=0.0, "Gas Mix Number"="", "Set STP Register"=FALSE, "Measurement Units"={"Abs. Pressure"="", "Gauge/Diff. Press."="", "Barometric Press."="", "Temperature"="", "Volume"="", "Mass"="", "Setpoint"="", "Valve Drive"="", "Totalizer"="", "Tot. Timer"="", "Tot. Avg. Flow"="", "Tot. Peak Flow"="", "Software Version"=""}}, "Meter 6"={"Meter Size"=0.0, "DAQ Output (Voltage)"=0.0, "Reference (Voltage)"=0.0, "Meter Present"=FALSE, "Meter Visa"="COM3", "Gas Type"="", "SLPM Error @ Zero"=0.0, "Gas Mix Number"="", "Set STP Register"=FALSE, "Measurement Units"={"Abs. Pressure"="", "Gauge/Diff. Press."="", "Barometric Press."="", "Temperature"="", "Volume"="", "Mass"="", "Setpoint"="", "Valve Drive"="", "Totalizer"="", "Tot. Timer"="", "Tot. Avg. Flow"="", "Tot. Peak Flow"="", "Software Version"=""}}, "Meter Bank 1"={"Flow Rate (BTU/HR)"=0.0, "ANSI Placeholder Array"=[], "15 Sec Avg Array"=[], "30 Sec Avg Array "=[], "ANSI Average (BTU/HR)"=0.0, "Panel Data"={"Meter Type (Gas)"="", "Heating Value (BTU/ft³)"=0.0, "Ft³ / Hr (SCFH)"=0.0, "15 Second Average (BTU/HR)"=0.0, "30 Second Average (BTU/HR)"=0.0, "Mass Flow"=0.0, "Vol. Flow"=0.0, "Gas Temperature"=0.0, "Gas Pressure"=0.0, "Tot.Flow"=0.0}, "Start ANSI"=FALSE, "ANSI Start Time"=0.0, "Restart ANSI"=FALSE, "Meter ID"=""}, "Meter Bank 2"={"Flow Rate (BTU/HR)"=0.0, "ANSI Placeholder Array"=[], "15 Sec Avg Array"=[], "30 Sec Avg Array "=[], "ANSI Average (BTU/HR)"=0.0, "Panel Data"={"Meter Type (Gas)"="", "Heating Value (BTU/ft³)"=0.0, "Ft³ / Hr (SCFH)"=0.0, "15 Second Average (BTU/HR)"=0.0, "30 Second Average (BTU/HR)"=0.0, "Mass Flow"=0.0, "Vol. Flow"=0.0, "Gas Temperature"=0.0, "Gas Pressure"=0.0, "Tot.Flow"=0.0}, "Start ANSI"=FALSE, "ANSI Start Time"=0.0, "Restart ANSI"=FALSE, "Meter ID"=""}, "Meter Bank 3"={"Flow Rate (BTU/HR)"=0.0, "ANSI Placeholder Array"=[], "15 Sec Avg Array"=[], "30 Sec Avg Array "=[], "ANSI Average (BTU/HR)"=0.0, "Panel Data"={"Meter Type (Gas)"="", "Heating Value (BTU/ft³)"=0.0, "Ft³ / Hr (SCFH)"=0.0, "15 Second Average (BTU/HR)"=0.0, "30 Second Average (BTU/HR)"=0.0, "Mass Flow"=0.0, "Vol. Flow"=0.0, "Gas Temperature"=0.0, "Gas Pressure"=0.0, "Tot.Flow"=0.0}, "Start ANSI"=FALSE, "ANSI Start Time"=0.0, "Restart ANSI"=FALSE, "Meter ID"=""}, "Threshold Voltage (NI DAQ)"=0.2, "Use RS232 Data Collection"=FALSE, "Use Auto Switching"=FALSE}
  in  "DAQ Data In":T40={"Meter 1"={"Meter Size"=0.0, "DAQ Output (Voltage)"=0.0, "Reference (Voltage)"=0.0, "Meter Present"=FALSE, "Meter Visa"="COM3", "Gas Type"="", "SLPM Error @ Zero"=0.0, "Gas Mix Number"="", "Set STP Register"=FALSE, "Measurement Units"={"Abs. Pressure"="", "Gauge/Diff. Press."="", "Barometric Press."="", "Temperature"="", "Volume"="", "Mass"="", "Setpoint"="", "Valve Drive"="", "Totalizer"="", "Tot. Timer"="", "Tot. Avg. Flow"="", "Tot. Peak Flow"="", "Software Version"=""}}, "Meter 2"={"Meter Size"=0.0, "DAQ Output (Voltage)"=0.0, "Reference (Voltage)"=0.0, "Meter Present"=FALSE, "Meter Visa"="COM3", "Gas Type"="", "SLPM Error @ Zero"=0.0, "Gas Mix Number"="", "Set STP Register"=FALSE, "Measurement Units"={"Abs. Pressure"="", "Gauge/Diff. Press."="", "Barometric Press."="", "Temperature"="", "Volume"="", "Mass"="", "Setpoint"="", "Valve Drive"="", "Totalizer"="", "Tot. Timer"="", "Tot. Avg. Flow"="", "Tot. Peak Flow"="", "Software Version"=""}}, "Meter 3"={"Meter Size"=0.0, "DAQ Output (Voltage)"=0.0, "Reference (Voltage)"=0.0, "Meter Present"=FALSE, "Meter Visa"="COM3", "Gas Type"="", "SLPM Error @ Zero"=0.0, "Gas Mix Number"="", "Set STP Register"=FALSE, "Measurement Units"={"Abs. Pressure"="", "Gauge/Diff. Press."="", "Barometric Press."="", "Temperature"="", "Volume"="", "Mass"="", "Setpoint"="", "Valve Drive"="", "Totalizer"="", "Tot. Timer"="", "Tot. Avg. Flow"="", "Tot. Peak Flow"="", "Software Version"=""}}, "Meter 4"={"Meter Size"=0.0, "DAQ Output (Voltage)"=0.0, "Reference (Voltage)"=0.0, "Meter Present"=FALSE, "Meter Visa"="COM3", "Gas Type"="", "SLPM Error @ Zero"=0.0, "Gas Mix Number"="", "Set STP Register"=FALSE, "Measurement Units"={"Abs. Pressure"="", "Gauge/Diff. Press."="", "Barometric Press."="", "Temperature"="", "Volume"="", "Mass"="", "Setpoint"="", "Valve Drive"="", "Totalizer"="", "Tot. Timer"="", "Tot. Avg. Flow"="", "Tot. Peak Flow"="", "Software Version"=""}}, "Meter 5"={"Meter Size"=0.0, "DAQ Output (Voltage)"=0.0, "Reference (Voltage)"=0.0, "Meter Present"=FALSE, "Meter Visa"="COM3", "Gas Type"="", "SLPM Error @ Zero"=0.0, "Gas Mix Number"="", "Set STP Register"=FALSE, "Measurement Units"={"Abs. Pressure"="", "Gauge/Diff. Press."="", "Barometric Press."="", "Temperature"="", "Volume"="", "Mass"="", "Setpoint"="", "Valve Drive"="", "Totalizer"="", "Tot. Timer"="", "Tot. Avg. Flow"="", "Tot. Peak Flow"="", "Software Version"=""}}, "Meter 6"={"Meter Size"=0.0, "DAQ Output (Voltage)"=0.0, "Reference (Voltage)"=0.0, "Meter Present"=FALSE, "Meter Visa"="COM3", "Gas Type"="", "SLPM Error @ Zero"=0.0, "Gas Mix Number"="", "Set STP Register"=FALSE, "Measurement Units"={"Abs. Pressure"="", "Gauge/Diff. Press."="", "Barometric Press."="", "Temperature"="", "Volume"="", "Mass"="", "Setpoint"="", "Valve Drive"="", "Totalizer"="", "Tot. Timer"="", "Tot. Avg. Flow"="", "Tot. Peak Flow"="", "Software Version"=""}}, "Meter Bank 1"={"Flow Rate (BTU/HR)"=0.0, "ANSI Placeholder Array"=[], "15 Sec Avg Array"=[], "30 Sec Avg Array "=[], "ANSI Average (BTU/HR)"=0.0, "Panel Data"={"Meter Type (Gas)"="", "Heating Value (BTU/ft³)"=0.0, "Ft³ / Hr (SCFH)"=0.0, "15 Second Average (BTU/HR)"=0.0, "30 Second Average (BTU/HR)"=0.0, "Mass Flow"=0.0, "Vol. Flow"=0.0, "Gas Temperature"=0.0, "Gas Pressure"=0.0, "Tot.Flow"=0.0}, "Start ANSI"=FALSE, "ANSI Start Time"=0.0, "Restart ANSI"=FALSE, "Meter ID"=""}, "Meter Bank 2"={"Flow Rate (BTU/HR)"=0.0, "ANSI Placeholder Array"=[], "15 Sec Avg Array"=[], "30 Sec Avg Array "=[], "ANSI Average (BTU/HR)"=0.0, "Panel Data"={"Meter Type (Gas)"="", "Heating Value (BTU/ft³)"=0.0, "Ft³ / Hr (SCFH)"=0.0, "15 Second Average (BTU/HR)"=0.0, "30 Second Average (BTU/HR)"=0.0, "Mass Flow"=0.0, "Vol. Flow"=0.0, "Gas Temperature"=0.0, "Gas Pressure"=0.0, "Tot.Flow"=0.0}, "Start ANSI"=FALSE, "ANSI Start Time"=0.0, "Restart ANSI"=FALSE, "Meter ID"=""}, "Meter Bank 3"={"Flow Rate (BTU/HR)"=0.0, "ANSI Placeholder Array"=[], "15 Sec Avg Array"=[], "30 Sec Avg Array "=[], "ANSI Average (BTU/HR)"=0.0, "Panel Data"={"Meter Type (Gas)"="", "Heating Value (BTU/ft³)"=0.0, "Ft³ / Hr (SCFH)"=0.0, "15 Second Average (BTU/HR)"=0.0, "30 Second Average (BTU/HR)"=0.0, "Mass Flow"=0.0, "Vol. Flow"=0.0, "Gas Temperature"=0.0, "Gas Pressure"=0.0, "Tot.Flow"=0.0}, "Start ANSI"=FALSE, "ANSI Start Time"=0.0, "Restart ANSI"=FALSE, "Meter ID"=""}, "Threshold Voltage (NI DAQ)"=0.2, "Use RS232 Data Collection"=FALSE, "Use Auto Switching"=FALSE}
  out "Measurments.Standby Power":T28={"Standby Power Spreadsheet"=[], "Standby Power - Pia (Watts)"=0.0, "Off Mode Power - Poff (Watts)"=0.0, "Sia hr/yr"=8620.0, "Soff hr/yr"=0.0, "Yearly Energy Etso kWh/yr"=0.0, "Maximum Power (Watts)"=0.0, "Power Variation (%)"=0.0, "Slope (mW/hr)"=0.0, "Final Harmonics-U1 (%)"="", "Final Harmonics-U2 (%)"="", "Energy (Wh)"=0.0}
  in  "Measurments":T26={"Power Measurements"={"Current (A):Element 1"=0.0, "Current (A):Element 2"=0.0, "Power (W):Sigma"=0.0, "Watt Hours (Wh):Sigma"=0.0, "Voltage (V):Element 2"=0.0, "Voltage (V):Element 1"=0.0, "Current Crest Factor:Element 1"=0.0, "Current Crest Factor:Element 2"=0.0, "Voltage Harmonic (%):Element 1"=0.0, "Voltage Harmonic (%):Element 2"=0.0, "Voltage Crest Factor:Element 1"=0.0, "Voltage Crest Factor:Element 2"=0.0, "Time:Element 1"=0.0, "Frequency (Hz):Element 1"=0.0, "Apparent Power (VA):Element 1"=0.0, "Apparent Power (VA):Element 2"=0.0, "Power Factor:Element 1"=0.0, "Power Factor:Element 2"=0.0, "Max Watt Hours"=0.0, "Voltage (V):Element 2 Avg"=0.0, "Voltage (V):Element 1 Avg"=0.0}, "Standby Power"={"Standby Power Spreadsheet"=[], "Standby Power - Pia (Watts)"=0.0, "Off Mode Power - Poff (Watts)"=0.0, "Sia hr/yr"=8620.0, "Soff hr/yr"=0.0, "Yearly Energy Etso kWh/yr"=0.0, "Maximum Power (Watts)"=0.0, "Power Variation (%)"=0.0, "Slope (mW/hr)"=0.0, "Final Harmonics-U1 (%)"="", "Final Harmonics-U2 (%)"="", "Energy (Wh)"=0.0}, "Washer"={"Washer String Data"=[], "Analog Scale Weight (lbs)"=0.0}, "Dishwasher"={"Drain Solonoid Event"=0, "Pump Event"=0, "Water Valve Event"=0, "Heater Event"=0, "Motor Event"=0, "Turbidity Sensor"=0.0, "Spare 2"=0.0, "Spare 3"=0.0, "Spare 4"=0.0, "Spare 5"=0.0, "Thermocouple 1"=0.0, "Thermocouple 2"=0.0, "Thermocouple 3"=0.0, "Thermocouple 4"=0.0, "Thermocouple 5"=0.0, "Thermocouple 6"=0.0, "Spare 1"=0.0, "Dishwasher String Data"=[]}, "Washer HCC"={"Chan 101"=0.0, "Chan 102"=0.0, "Chan 103"=0.0, "Chan 104"=0.0, "Chan 105"=0.0, "Chan 106"=0.0, "Chan 107"=0.0, "Chan 108"=0.0, "Chan 109"=0.0, "Chan 110"=0.0, "Chan 111"=0.0, "Chan 112"=0.0, "Chan 113"=0.0, "Chan 114"=0.0, "Chan 115"=0.0, "Chan 116"=0.0, "Chan 117"=0.0, "Chan 118"=0.0, "Chan 119"=0.0, "Chan 120"=0.0, "Chan 201"=0.0, "Chan 202"=0.0, "Chan 203"=0.0, "Chan 204"=0.0, "Chan 205"=0.0, "Chan 206"=0.0, "Chan 207"=0.0, "Chan 208"=0.0, "Chan 209"=0.0, "Chan 210"=0.0, "Chan 211"=0.0, "Chan 212"=0.0, "Chan 213"=0.0, "Chan 214"=0.0, "Chan 215"=0.0, "Chan 216"=0.0, "Chan 217"=0.0, "Chan 218"=0.0, "Chan 219"=0.0, "Chan 220"=0.0, "Chan 301"=0.0, "Chan 302"=0.0, "Chan 303"=0.0, "Chan 304"=0.0, "Chan 305"=0.0, "Chan 306"=0.0, "Chan 307"=0.0, "Chan 308"=0.0, "Chan 309"=0.0, "Chan 310"=0.0, "Chan 311"=0.0, "Chan 312"=0.0, "Chan 313"=0.0, "Chan 314"=0.0, "Chan 315"=0.0, "Chan 316"=0.0, "Chan 317"=0.0, "Chan 318"=0.0, "Chan 319"=0.0, "Chan 320"=0.0}, "Barometric Pressure"={"Barometric Pressure (in. Hg)"=0.0}, "Ambient Conditions"={"Ambient Temperature  1 (°F)"=0.0, "Ambient Temperature 2 (°F)"=0.0, "Ambient Temperature 3 (°F)"=0.0, "Ambient Humidity 1 (%)"=0.0, "Ambient Humidity 2 (%)"=0.0, "Ambient Humidity 3 (%)"=0.0, "Ambient Dewpoint  1 (°F)"=0.0, "Ambient Dewpoint 2 (°F)"=0.0, "Ambient Dewpoint 3 (°F)"=0.0}, "Weight Scale"={"Gross Weigth (lbs)"=0.0, "Net Weight (lbs)"=0.0, "Final Weight (lbs)"=""}, "Water Measurements"={"Hot Water Pressure (psi)"=0.0, "Hot Water Pressure Max (psi)"=0.0, "Hot Water Temperature (°F)"=0.0, "Cold Water Pressure (psi)"=0.0, "Cold Water Pressure Max (psi)"=0.0, "Hot Water Temperature Max (°F)"=0.0, "Cold Water Temperature (°F)"=0.0, "Cold Water Temperature Max (°F)"=0.0, "Hot Water Total (Gal)"=0.0, "Hot Water Rate (GPM)"=0.0, "Cold Water Total (Gal)"=0.0, "Cold Water Rate (GPM)"=0.0, "Cold Water Total During Wash (Gal)"=0.0, "Hot Water Total During Wash (Gal)"=0.0, "Rinse Cold (Gal)"=0.0, "Rinse Hot (Gal)"=0.0, "Hot Water Pressure Min (psi)"=0.0, "Hot Water Temperature Min (°F)"=0.0, "Cold Water Pressure Min (psi)"=0.0, "Cold Water Temperature Min (°F)"=0.0}, "Gas Data"={"Meter Type (Gas)"="", "Meter ID"=enum."Disabled", "Heating Value (BTU/ft³)"=0.0, "Ft³ / Hr (SCFH)"=0.0, "15 Second Average (BTU/HR)"=0.0, "30 Second Average (BTU/HR)"=0.0, "SLPM (Mass Flow)"=0.0, "LPM (Vol. Flow)"=0.0, "Gas Temperature (°F)"=0.0, "Gas Pressure (PSIA)"=0.0, "Tot.Flow (Liters)"=0.0}} {"Power Measurements"."Voltage (V):Element 1 Avg" format="%.3g"; "Power Measurements"."Voltage (V):Element 2 Avg" format="%.3g"; "Power Measurements"."Max Watt Hours" format="%.3g"; "Power Measurements"."Power Factor:Element 2" format="%.3g"; "Power Measurements"."Power Factor:Element 1" format="%.3g"; "Power Measurements"."Apparent Power (VA):Element 2" format="%.3g"; "Power Measurements"."Apparent Power (VA):Element 1" format="%.3g"; "Power Measurements"."Frequency (Hz):Element 1" format="%.3g"; "Power Measurements"."Time:Element 1" format="%.3g"; "Power Measurements"."Voltage Crest Factor:Element 2" format="%.3g"; "Power Measurements"."Voltage Crest Factor:Element 1" format="%.3g"; "Power Measurements"."Voltage Harmonic (%):Element 2" format="%.3g"; "Power Measurements"."Voltage Harmonic (%):Element 1" format="%.3g"; "Power Measurements"."Current Crest Factor:Element 2" format="%.3g"; "Power Measurements"."Current Crest Factor:Element 1" format="%.3g"; "Power Measurements"."Voltage (V):Element 1" format="%.3g"; "Power Measurements"."Voltage (V):Element 2" format="%.3g"; "Power Measurements"."Watt Hours (Wh):Sigma" format="%.3f"; "Power Measurements"."Power (W):Sigma" format="%.3g"; "Power Measurements"."Current (A):Element 2" format="%.3g"; "Power Measurements"."Current (A):Element 1" format="%.3g"}
  # "Standby Power Analysis"
  # "Gas Meter"
  # "WT500 Wiring Configuration"
  # "Rinse Cycle Search Commands"
  # "Read External Software"
  # "Step 1: Select File"
  # "Step 2: Start Reading"
  # "Cold Dryer Weight (Activate in Log Data Screen)"
  # "Step 1: Pre-Condition Dryer (No Load)"
  # "General Configuration"
  # "Auto Terminate Features"
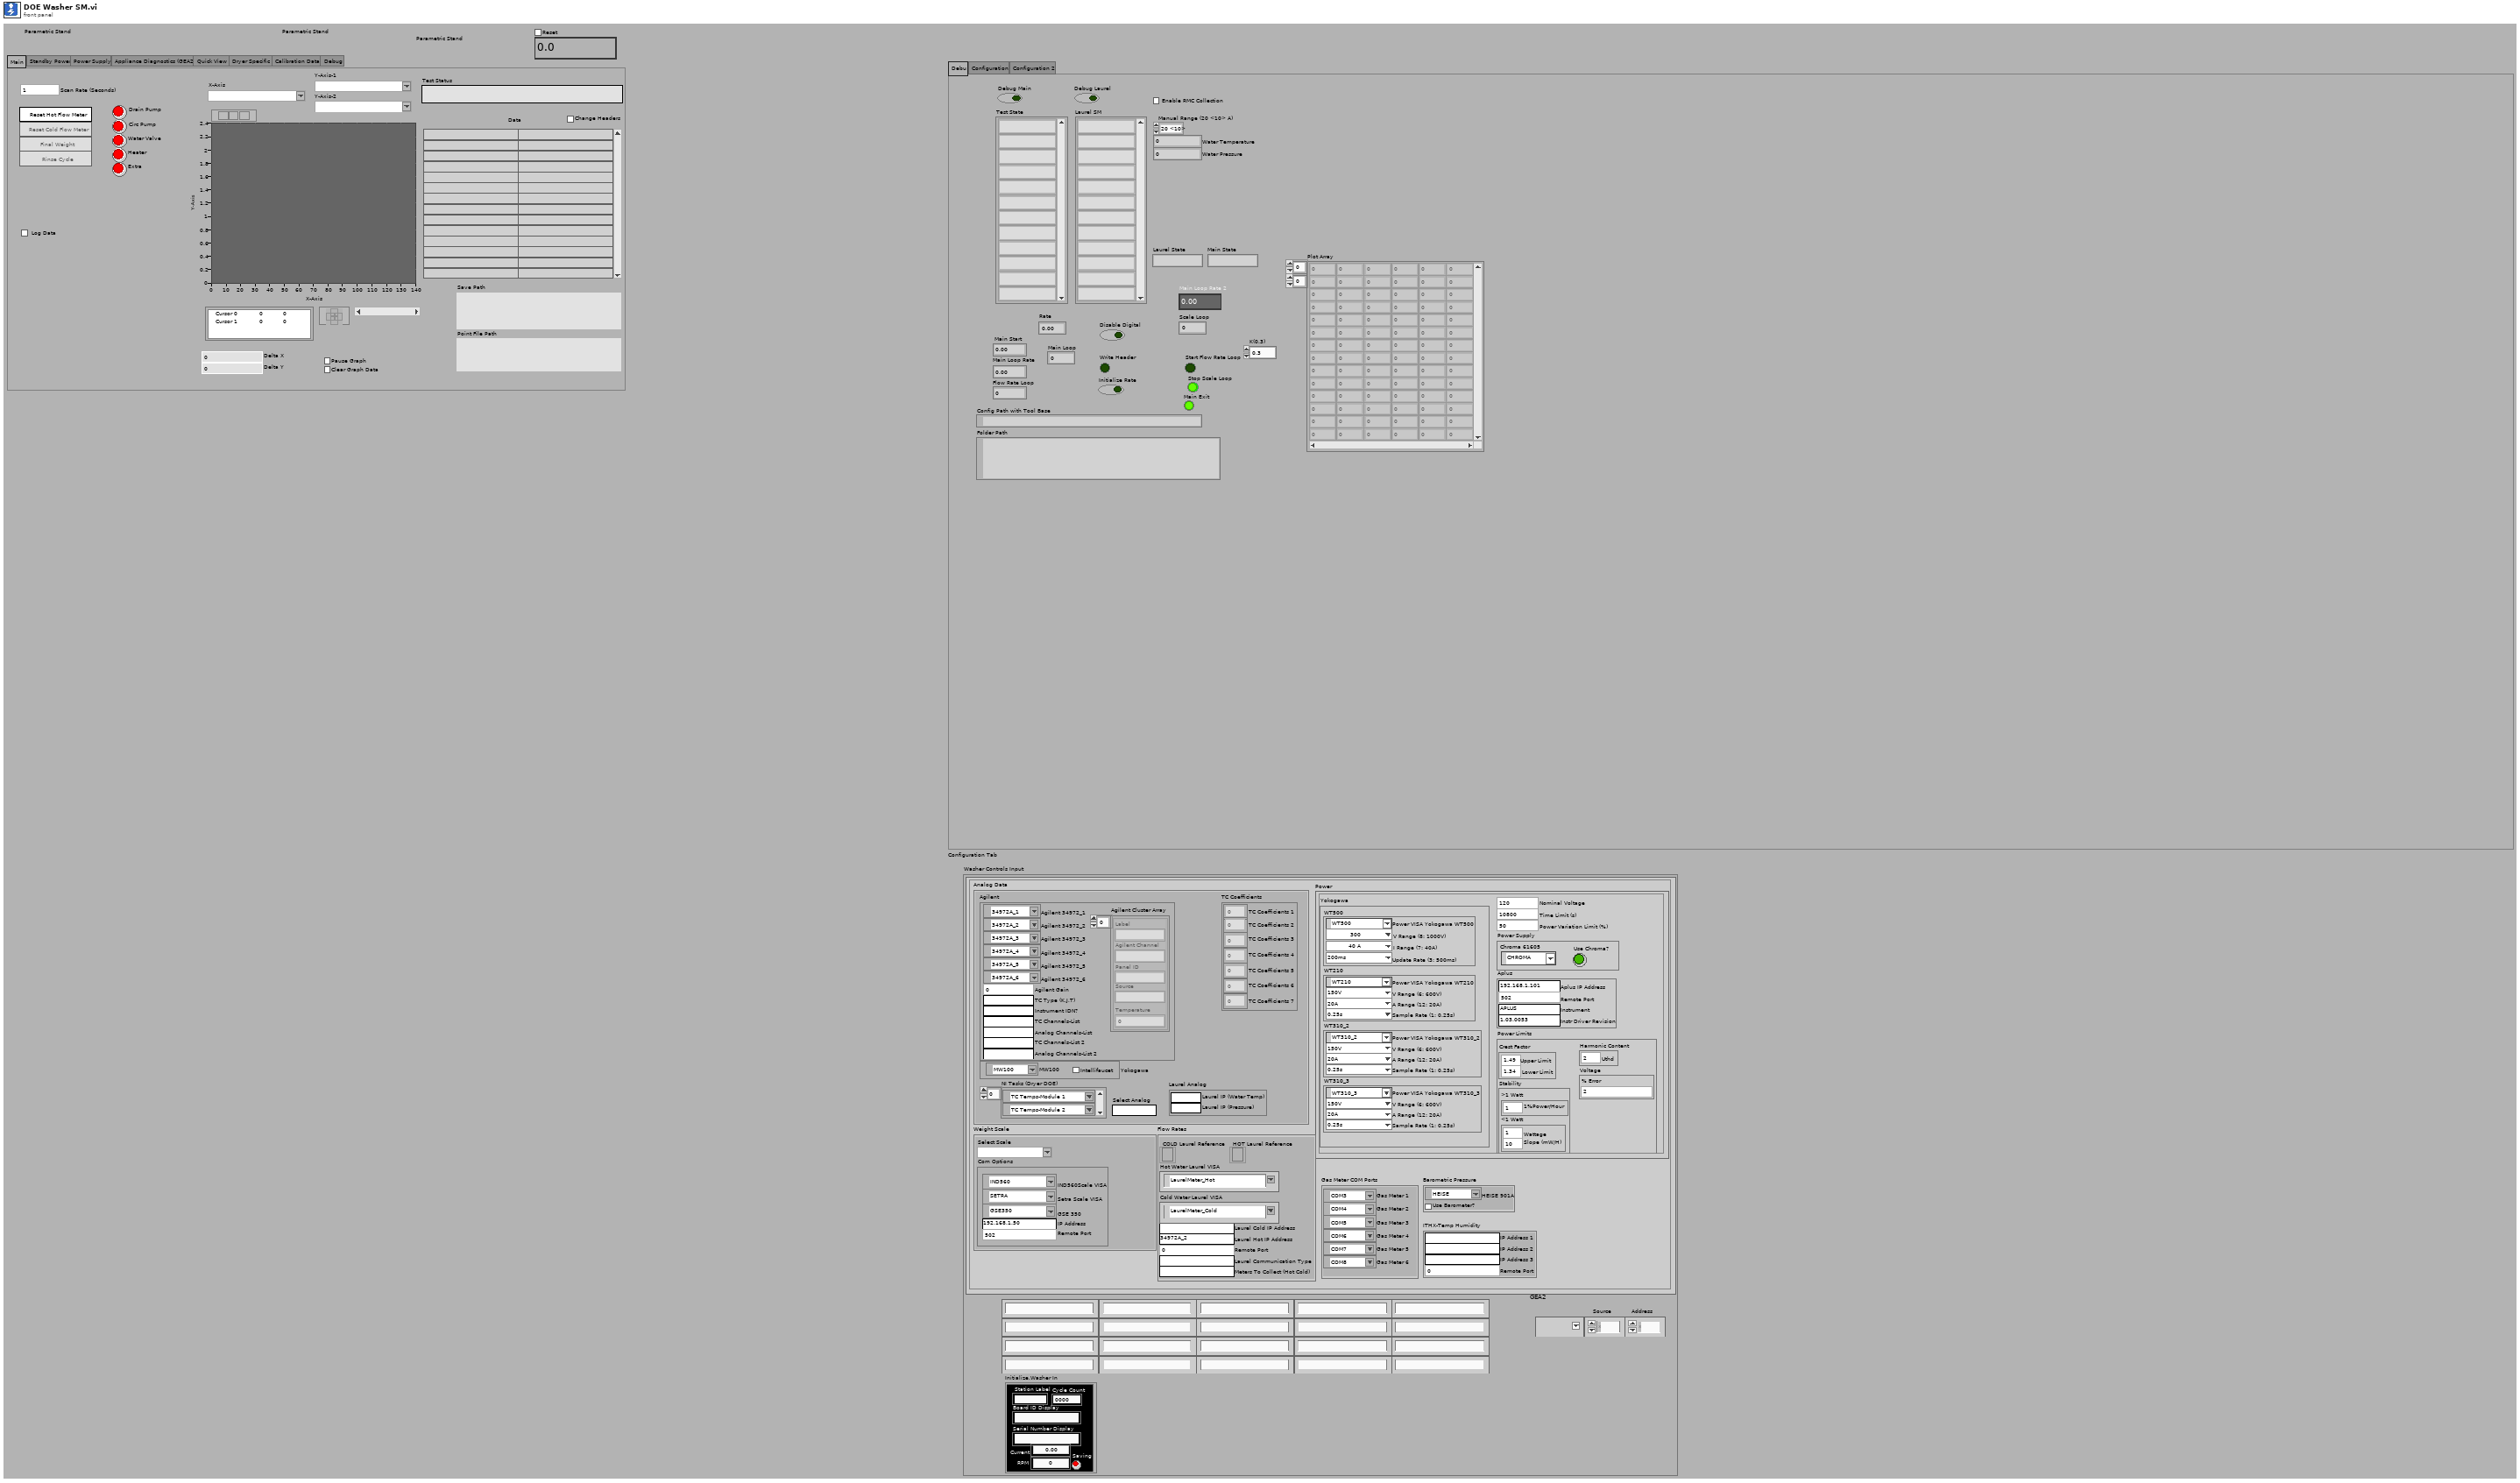
[diagram p1: front panel]
types:
  T1 = enum32{"Main", "Standby Power", "Power Supply", "Appliance Diagnostics (GEA2)", "Quick View", "Dryer Specific", "Calibration Data", "Debug"}
  T2 = typedef "DOE Dishwasher Events.ctl" = cluster{"Drain Pump":bool, "Circ Pump":bool, "Water Valve":bool, "Heater":bool, "Extra":bool}
  T3 = cluster{"Time Array Output":dbl[], "Data Array Output":dbl[]}[]
  T4 = typedef "CHROMA Phase Shift Lines.ctl" = enum16{"P1 and P2", "P1 and P3"}
  T5 = typedef "CHROMA Voltage Range.ctl" = enum16{"High (300V)", "Low (150V)"}
  T6 = typedef "WT500 Wiring Control.ctl" = u16
  T7 = typedef "DOE Dryer NI Card Settings.ctl" = cluster{"Disable NI Card 1":bool, "Disable NI Card 2":bool, "Disable NI Card 3":bool, "Disable NI Card 4":bool, "Disable NI Card 5":bool, "Disable NI Card 6":bool, "Disable NI Card 7":bool}
  T8 = typedef "DOE Main Control.ctl" = cluster{"Test Fixture Hardware":T9, "GEA2":T15, "DOE Capacity Measurments":T16, "Initialize.Washer In":T17}
  T9 = typedef "DOE Test Fixture Hardware.ctl" = cluster{"Power ":T10, "Weight Scale":cluster{"Com Options":T11, "Select Scale":string}, "Flow Rates":cluster{"Laurel Cold IP Address":string, "Laurel Hot IP Address":string, "Hot Water Laurel VISA":refnum<visa-resource-name>, "Cold Water Laurel VISA":refnum<visa-resource-name>, "Remote Port":u16, "Laurel Communication Type":string, "Meters To Collect (Hot Cold)":string, "HOT Laurel Reference":refnum<k5>, "COLD Laurel Reference":refnum<k5>}, "Analog Data":cluster{"Agilent":cluster{"Agilent 34972_1":refnum<visa-resource-name>, "Agilent 34972_2":refnum<visa-resource-name>, "Agilent 34972_3":refnum<visa-resource-name>, "Agilent 34972_4":refnum<visa-resource-name>, "Agilent 34972_5":refnum<visa-resource-name>, "Agilent 34972_6":refnum<visa-resource-name>, "Agilent Gain":dbl, "TC Type (K,J,T)":string, "Instrument IDN?":string, "TC Channels-List":string, "Analog Channels-List":string, "Agilent Cluster Array":T12[], "TC Channels-List 2":string, "Analog Channels-List 2":string}, "Yokogawa":cluster{"MW100":refnum<visa-resource-name>, "Intellifaucet":bool}, "Select Analog":string, "TC Coefficients":T13, "NI Tasks (Dryer DOE)":refnum<k21>[], "Laurel Analog":cluster{"Laurel IP (Water Temp)":string, "Laurel IP (Pressure)":string}}, "ITHX-Temp Humidity":cluster{"IP Address 1":string, "Remote Port":u16, "IP Address 2":string, "IP Address 3":string}, "Gas Meter COM Ports":T14, "Barometric Pressure":cluster{"HEISE 901A":refnum<visa-resource-name>, "Use Barometer?":bool}}
  T10 = typedef "UTILITY Power Inputs Control.ctl" = cluster{"Yokogawa":cluster{"WT210":cluster{"Sample Rate (1: 0.25s)":i32, "A Range (12: 20A)":i32, "V Range (6: 600V)":i32, "Power VISA Yokogawa WT210":refnum<visa-resource-name>}, "WT500":cluster{"Power VISA Yokogawa WT500":refnum<visa-resource-name>, "V Range (8: 1000V)":i32, "I Range (7: 40A)":i32, "Update Rate (3: 500ms)":i32}, "WT310_2":cluster{"Sample Rate (1: 0.25s)":i32, "A Range (12: 20A)":i32, "V Range (6: 600V)":i32, "Power VISA Yokogawa WT310_2":refnum<visa-resource-name>}, "WT310_3":cluster{"Sample Rate (1: 0.25s)":i32, "A Range (12: 20A)":i32, "V Range (6: 600V)":i32, "Power VISA Yokogawa WT310_3":refnum<visa-resource-name>}}, "Aplus":cluster{"Aplus IP Address":string, "Remote Port":i32, "Instrument":string, "Instr Driver Revision":string}, "Power Limits":cluster{"Crest Factor":cluster{"Upper Limit":dbl, "Lower Limit":dbl}, "Harmonic Content":cluster{"Uthd":dbl}, "Voltage":cluster{"% Error":dbl}, "Stability":cluster{"<1 Watt ":cluster{"Wattage":dbl, "Slope (mW/H)":dbl}, ">1 Watt":cluster{"1%Power/Hour":dbl}}}, "Nominal Voltage":i32, "Time Limit (s)":dbl, "Power Variation Limit (%)":dbl, "Power Supply":cluster{"Chroma 61605":refnum<visa-resource-name>, "Use Chroma?":bool}}
  T11 = typedef "IND560 Configuration.ctl" = cluster{"IND560Scale VISA":refnum<visa-resource-name>, "IP Address":string, "Remote Port":u16, "Setra Scale VISA":refnum<visa-resource-name>, "GSE 350":refnum<visa-resource-name>}
  T12 = typedef "HEWH Agilent Cluster.ctl" = cluster{"Label":string, "Agilent Channel":string, "Panel ID":string, "Source":string, "Temperature":dbl}
  T13 = typedef "UTILITY TC Coefficients.ctl" = cluster{"TC Coefficients 1":dbl[], "TC Coefficients 2":dbl[], "TC Coefficients 3":dbl[], "TC Coefficients 4":dbl[], "TC Coefficients 5":dbl[], "TC Coefficients 6":dbl[], "TC Coefficients 7":dbl[]}
  T14 = typedef "FMA1600A COM Ports.ctl" = cluster{"Gas Meter 1":refnum<visa-resource-name>, "Gas Meter 2":refnum<visa-resource-name>, "Gas Meter 3":refnum<visa-resource-name>, "Gas Meter 4":refnum<visa-resource-name>, "Gas Meter 5":refnum<visa-resource-name>, "Gas Meter 6":refnum<visa-resource-name>}
  T15 = typedef "GEA2.ctl" = cluster{"Address":u8, "Source":u8, "Viper/Hawk":u8}
  T16 = typedef "DOE Capacity Measurments.ctl" = cluster{"Weight 1":dbl, "Model Number 1":string, "Temp 1":dbl, "Serial Number 1":string, "Lab Number 1":string, "Lab Number 2":string, "Serial Number 2":string, "Temp 2":dbl, "Model Number 2":string, "Weight 2":dbl, "Lab Number 3":string, "Serial Number 3":string, "Temp 3":dbl, "Model Number 3":string, "Weight 3":dbl, "Lab Number 4":string, "Serial Number 4":string, "Temp 4":dbl, "Model Number 4":string, "Weight 4":dbl, "Capacity Measurment Output String":string[][]}
  T17 = typedef "Save File.lvlib/Save File Washer.ctl" = cluster{"Appliance Details":T18, "Display Data (RLT)":T24}
  T18 = typedef "File Setup.lvlib/Save File DISH Dishwasher Details.ctl" = cluster{"FileVersionInfo":T19, "Dishwasher Info":cluster{"Open Cup Weight (gm):":dbl, "Auto Cup Weight (gm):":dbl, "Detergent-Dish:":string, "Inlet Temperature-Dish:":string, "Cycle Mode-Dish:":string, "Unit Control-Dish:":string, "Manufacturer-Dish:":string}, "Washer Info":cluster{"Hot Water Temperature (Fahrenheit):":string, "Cold Water Temperature (Fahrenheit):":string, "Capacity (cu.ft):":dbl, "Initial Cloth Weight:":dbl, "Cloth Lot:":i32, "Model Family:":string, "Program Name:":string, "Cycle Selection:":string, "Wash Temperature:":string, "Rinse Temperature:":string, "Load Size:":string}, "File Name Output Array":string[][], "Calibration Output Array":string[][], "Appliance Common":T20, "Water Heater":cluster{"Heating Mode:":string}, "Dryer":cluster{"Heat Setting:":T21, "Washer Water Temperature (60 ± 5°F):":u16, "Water Hardness (PPM):":u16, "Dryness Setting:":T21, "Dryer Type:":string, "Exhaust:":string, "Drying Cycle:":string, "Load Type:":string, "Nominal Load Weight":string, "Dryer Initial IMC Data":T22}}
  T19 = typedef "FileVersionInformation.ctl" = cluster{"FileVersion":string, "ProductName":string, "InternalName":string, "CompanyName":string, "LegalCopyright":string, "FileDescription":string}
  T20 = typedef "DOE Appliance Common.ctl" = cluster{"Engineer:":string, "Model Number:":string, "Serial Number:":string, "Comments:":string, "Station ID:":string, "Technician:":string, "TR Number:":string, "Lab ID:":string, "Voltage:":string, "Water Pressure (PSI):":string, "Test Date:":string, "Computer Name:":string, "IP Address:":string, "Ambient RH:":string, "Frequency:":string, "Build:":string, "Filename:":string, "Test Type:":string, "Load Run #:":i32, "Ambient Temperature (F):":string, "File Path:":path, "Cycles Per Year":u32}
  T21 = typedef "Custom Pallet String.ctl" = string
  T22 = typedef "DPT IMC Data.ctl" = cluster{"Measured IMC (lbs)":dbl, "Actual Initial RMC (%)":dbl, "RMC (Desired %)":dbl, "Bone Dry Wt(lbs)":dbl, "Tolerance(%)":dbl, "Actual Final RMC (%)":dbl, "CEF (lbf/kWh)":dbl, "Minimum Weight (lbf)":dbl, "Average Weight (lbf)":dbl, "Maximum Weight (lbf)":dbl, "Measured IMC In Range?":bool, "Moisture Reduction Factor":dbl, "Field Use Factor":dbl, "Empty Dryer Cold Weigth":dbl, "Energy Standard":T23, "Weight Cloth (lbs)":dbl, "Relative Moisture Content (%)":dbl, "Relative Moisture Content - Avg (%)":dbl}
  T23 = typedef "DOE Dryer Standard.ctl" = enum16{"D2-Automatic Dryer", "D2-Timer Dryer", "D1-Automatic Dryer", "D1-Timer Dryer", "Other"}
  T24 = typedef "Save File Appliance Display.ctl" = cluster{"Status Color":u32, "Serial Number Display":string, "Cycle Count Display":i32, "Station Label Display":string, "Current Run Start Time Display":dbl, "Board ID Display":string, "RPM Display":u32, "Current Display":dbl, "Current Path Display":path, "Saving Display":bool, "Unit Type Display":T25, "Total Time On Display":dbl, "UI Button":bool}
  T25 = typedef "Save File.lvlib/Save File Unit Type.ctl" = enum32{"", "Viper", "Hawk", "2015"}
  T26 = typedef "DOE Front Panel Meters.ctl" = cluster{"Power Measurements":T27, "Standby Power":T28, "Washer":cluster{"Washer String Data":string[][], "Analog Scale Weight (lbs)":dbl}, "Dishwasher":cluster{"Drain Solonoid Event":i32, "Pump Event":i32, "Water Valve Event":i32, "Heater Event":i32, "Motor Event":i32, "Turbidity Sensor":dbl, "Spare 2":dbl, "Spare 3":dbl, "Spare 4":dbl, "Spare 5":dbl, "Thermocouple 1":dbl, "Thermocouple 2":dbl, "Thermocouple 3":dbl, "Thermocouple 4":dbl, "Thermocouple 5":dbl, "Thermocouple 6":dbl, "Spare 1":dbl, "Dishwasher String Data":string[][]}, "Washer HCC":cluster{"Chan 101":dbl, "Chan 102":dbl, "Chan 103":dbl, "Chan 104":dbl, "Chan 105":dbl, "Chan 106":dbl, "Chan 107":dbl, "Chan 108":dbl, "Chan 109":dbl, "Chan 110":dbl, "Chan 111":dbl, "Chan 112":dbl, "Chan 113":dbl, "Chan 114":dbl, "Chan 115":dbl, "Chan 116":dbl, "Chan 117":dbl, "Chan 118":dbl, "Chan 119":dbl, "Chan 120":dbl, "Chan 201":dbl, "Chan 202":dbl, "Chan 203":dbl, "Chan 204":dbl, "Chan 205":dbl, "Chan 206":dbl, "Chan 207":dbl, "Chan 208":dbl, "Chan 209":dbl, "Chan 210":dbl, "Chan 211":dbl, "Chan 212":dbl, "Chan 213":dbl, "Chan 214":dbl, "Chan 215":dbl, "Chan 216":dbl, "Chan 217":dbl, "Chan 218":dbl, "Chan 219":dbl, "Chan 220":dbl, "Chan 301":dbl, "Chan 302":dbl, "Chan 303":dbl, "Chan 304":dbl, "Chan 305":dbl, "Chan 306":dbl, "Chan 307":dbl, "Chan 308":dbl, "Chan 309":dbl, "Chan 310":dbl, "Chan 311":dbl, "Chan 312":dbl, "Chan 313":dbl, "Chan 314":dbl, "Chan 315":dbl, "Chan 316":dbl, "Chan 317":dbl, "Chan 318":dbl, "Chan 319":dbl, "Chan 320":dbl}, "Barometric Pressure":cluster{"Barometric Pressure (in. Hg)":dbl}, "Ambient Conditions":cluster{"Ambient Temperature  1 (°F)":dbl, "Ambient Temperature 2 (°F)":dbl, "Ambient Temperature 3 (°F)":dbl, "Ambient Humidity 1 (%)":dbl, "Ambient Humidity 2 (%)":dbl, "Ambient Humidity 3 (%)":dbl, "Ambient Dewpoint  1 (°F)":dbl, "Ambient Dewpoint 2 (°F)":dbl, "Ambient Dewpoint 3 (°F)":dbl}, "Weight Scale":cluster{"Gross Weigth (lbs)":dbl, "Net Weight (lbs)":dbl, "Final Weight (lbs)":string}, "Water Measurements":cluster{"Hot Water Pressure (psi)":dbl, "Hot Water Pressure Max (psi)":dbl, "Hot Water Temperature (°F)":dbl, "Cold Water Pressure (psi)":dbl, "Cold Water Pressure Max (psi)":dbl, "Hot Water Temperature Max (°F)":dbl, "Cold Water Temperature (°F)":dbl, "Cold Water Temperature Max (°F)":dbl, "Hot Water Total (Gal)":dbl, "Hot Water Rate (GPM)":dbl, "Cold Water Total (Gal)":dbl, "Cold Water Rate (GPM)":dbl, "Cold Water Total During Wash (Gal)":dbl, "Hot Water Total During Wash (Gal)":dbl, "Rinse Cold (Gal)":dbl, "Rinse Hot (Gal)":dbl, "Hot Water Pressure Min (psi)":dbl, "Hot Water Temperature Min (°F)":dbl, "Cold Water Pressure Min (psi)":dbl, "Cold Water Temperature Min (°F)":dbl}, "Gas Data":T29}
  T27 = typedef "UTILITY Power Data.ctl" = cluster{"Current (A):Element 1":dbl, "Current (A):Element 2":dbl, "Power (W):Sigma":dbl, "Watt Hours (Wh):Sigma":dbl, "Voltage (V):Element 2":dbl, "Voltage (V):Element 1":dbl, "Current Crest Factor:Element 1":dbl, "Current Crest Factor:Element 2":dbl, "Voltage Harmonic (%):Element 1":dbl, "Voltage Harmonic (%):Element 2":dbl, "Voltage Crest Factor:Element 1":dbl, "Voltage Crest Factor:Element 2":dbl, "Time:Element 1":dbl, "Frequency (Hz):Element 1":dbl, "Apparent Power (VA):Element 1":dbl, "Apparent Power (VA):Element 2":dbl, "Power Factor:Element 1":dbl, "Power Factor:Element 2":dbl, "Max Watt Hours":dbl, "Voltage (V):Element 2 Avg":dbl, "Voltage (V):Element 1 Avg":dbl}
  T28 = typedef "Standby Power Main Data.ctl" = cluster{"Standby Power Spreadsheet":string[][], "Standby Power - Pia (Watts)":dbl, "Off Mode Power - Poff (Watts)":dbl, "Sia hr/yr":dbl, "Soff hr/yr":dbl, "Yearly Energy Etso kWh/yr":dbl, "Maximum Power (Watts)":dbl, "Power Variation (%)":dbl, "Slope (mW/hr)":dbl, "Final Harmonics-U1 (%)":string, "Final Harmonics-U2 (%)":string, "Energy (Wh)":dbl}
  T29 = typedef "FMA1600A Gas Data.ctl" = cluster{"Meter Type (Gas)":T30, "Meter ID":T31, "Heating Value (BTU/ft³)":dbl, "Ft³ / Hr (SCFH)":dbl, "15 Second Average (BTU/HR)":dbl, "30 Second Average (BTU/HR)":dbl, "SLPM (Mass Flow)":dbl, "LPM (Vol. Flow)":dbl, "Gas Temperature (°F)":dbl, "Gas Pressure (PSIA)":dbl, "Tot.Flow (Liters)":dbl}
  T30 = typedef "FMA1600A Gas Type.ctl" = string
  T31 = typedef "RANGE Meter Selector 1-2.ctl" = enum16{"Disabled", "Meter 1", "Meter 2", "Auto"}
  T32 = typedef "File Setup.lvlib/Save File DOE Configuration State.ctl" = enum16{"Open Front Panel", "Load Config"}
  T33 = typedef "Custom Pallet Timer.ctl" = dbl
  T34 = enum32{"Debu", "Configuration", "Configuration 2"}
  T35 = typedef "Custom Pallet DBL.ctl" = dbl
  T36 = enum32{"Hardware Setup", "Raw Data", "File Setup"}
  T37 = typedef "UTILITY Power Analyzer.ctl" = enum16{"", "APLUS", "WT210", "WT500", "WT300", "OSI", "Debug", "WT230", "WT300_1", "WT300_2"}
  T38 = typedef "File Setup.lvlib/Save File DOE File Path Control.ctl" = cluster{"General Setup Paths":cluster{"Calibration File Path":path, "DOE Capacity Path":path, "Data Folder Path":path, "RLT Backup Data Path":path, "Tool Base Path":path, "General Startup Config Path":path, "File Save Previous Run Path":path, "File Save Configuration Data Path":path}, "Data File Paths":T39, "New Summary Created":bool, "Check Location Interval (Second)":i32}
  T39 = typedef "File Setup.lvlib/Save File DOE Data Save Filepaths.ctl" = cluster{"Data File Path":path, "Debug File Path":path, "Bus Log Path":path, "Current":path, "Summary":path}
  T40 = typedef "RANGE DAQ Data Four Meters.ctl" = cluster{"Meter 1":T41, "Meter 2":T41, "Meter 3":T41, "Meter 4":T41, "Meter 5":T41, "Meter 6":T41, "Meter Bank 1":T43, "Meter Bank 2":T43, "Meter Bank 3":T43, "Threshold Voltage (NI DAQ)":dbl, "Use RS232 Data Collection":bool, "Use Auto Switching":bool}
  T41 = typedef "RANGE DAQ Data.ctl" = cluster{"Meter Size":dbl, "DAQ Output (Voltage)":dbl, "Reference (Voltage)":dbl, "Meter Present":bool, "Meter Visa":refnum<visa-resource-name>, "Gas Type":T30, "SLPM Error @ Zero":dbl, "Gas Mix Number":string, "Set STP Register":bool, "Measurement Units":T42}
  T42 = typedef "FMA1600A Units String.ctl" = cluster{"Abs. Pressure":string, "Gauge/Diff. Press.":string, "Barometric Press.":string, "Temperature":string, "Volume":string, "Mass":string, "Setpoint":string, "Valve Drive":string, "Totalizer":string, "Tot. Timer":string, "Tot. Avg. Flow":string, "Tot. Peak Flow":string, "Software Version":string}
  T43 = typedef "RANGE GAS Data.ctl" = cluster{"Flow Rate (BTU/HR)":dbl, "ANSI Placeholder Array":dbl[], "15 Sec Avg Array":dbl[], "30 Sec Avg Array ":dbl[], "ANSI Average (BTU/HR)":dbl, "Panel Data":T44, "Start ANSI":bool, "ANSI Start Time":dbl, "Restart ANSI":bool, "Meter ID":string}
  T44 = typedef "RANGE Panel Data.ctl" = cluster{"Meter Type (Gas)":T30, "Heating Value (BTU/ft³)":dbl, "Ft³ / Hr (SCFH)":dbl, "15 Second Average (BTU/HR)":dbl, "30 Second Average (BTU/HR)":dbl, "Mass Flow":dbl, "Vol. Flow":dbl, "Gas Temperature":dbl, "Gas Pressure":dbl, "Tot.Flow":dbl}
  T45 = enum8{"Enabled", "Disabled", "Disabled and Grayed Out"}
  T46 = typedef "FMA1600A Commands.ctl" = string
  T47 = typedef "Laurel Serial Commands.ctl" = string
  T48 = typedef "Range Meter Bank.ctl" = enum16{"Meter Bank 1", "Meter Bank 2", "Meter Bank 3"}
  T49 = typedef "File Setup.lvlib/Save File DOE LabView Program.ctl" = enum16{"No Name Found", "DOE Stand", "Dishwasher Kitchen", "Portable Stand", "HEWH", "Dryer", "Dryer WILT", "HCC", "PRAT", "HEWH RLT", "Refrigeration"}
  T50 = cluster{"LV Program":T49, "Fixture Hardware":T9, "DAQ Data In":T40}
  T51 = typedef "VISA Open Access Mode.ctl" = u32
  T52 = typedef "whitespace.ctl" = u16
  T53 = typedef "RTS Room Selector.ctl" = string
  T54 = typedef "CHROMA Phase.ctl" = enum16{"P1", "P2", "P3"}
  T55 = typedef "CHROMA Output State.ctl" = enum16{"Chroma OFF", "Chroma ON"}
  T56 = enum32{"invalid app kind", "Development System", "Run Time System", "Student Edition", "Embedded LabVIEW", "Evaluation", "Custom"}
  T57 = cluster{"Current VI Reference":refnum<vi>, "Close Panel on Exit?":bool}
  T58 = enum32{"Invalid", "Standard", "Closed", "Hidden", "Minimized", "Maximized"}
  T59 = typedef "DOE Data Logger Type.ctl" = enum16{"MW100", "Agilent", "Agilent_Laurel_DC_Clamp"}
  T60 = typedef "GEA2 Commands Washer logData.ctl" = cluster{"IGBT Temp (Deg C)":u8, "Speed":u32, "Load Size":u32, "Temperature":u8, "Water Pressure":u32, "Detergent":u32, "Fabric Softener":u32, "Direction":string, "Det":bool, "FS":bool, "Recirc":bool, "Drain":bool, "Hot":bool, "Cold":bool, "LidClosed":bool, "LidLocked":bool, "Motor Speed":u16, "Latched Out Of Balance":u16, "Raw Out Of Balance":u16, "Plaster Status":u8, "Inverter Power (Watts)":u16, "Profiler Status":string, "Profiler CRC":u16, "Current Inverter Action":string, "Target Speed (BRPM)":u16, "Latched Agitate Motor Temp (Deg C)":u8, "Current Motor Temp (Deg C)":u8, "Error Codes 1":string}
  T61 = typedef "File Setup.lvlib/Save File DOE Model Information.ctl" = cluster{"Model Information":string[][], "Program Names":string[], "Search Program Name":string, "Parsed Program List":string[][], "Header":string[], "Search Model Name":string, "File Search Parameters":string[], "Test Date":timestamp, "AF/MF Unit Number":string, "Stby Pwr Unit":string, "Model Details Header":string[], "Model Details Output":string[][], "End of Cycle Commands":string[], "Raw Data":string[][], "Startup Config Data":string[][]}
  T62 = cluster{"Core":cluster{"Current VI Reference":refnum<vi>, "Close Panel on Exit?":bool}, "Total Array":string[][], "Measurments":T26, "Calibration":string[][], "Filepath":T38, "Laundry GEA2 Data":T60, "Configuration File Param":T61, "Excel Report":refnum<class "NI_report.lvclass">, "Washer Controls Input":T8, "Power Analyzer":T37, "Save Data":string[][], "Plot Array":dbl[][], "New File":bool, "Reset Timer":bool, "Full Data Output":string[][], "Wait for Power Threshold (Output)":bool, "Force Read Point":bool}
  T63 = cluster{"WT210":cluster{"Sample Rate (1: 0.25s)":i32, "A Range (12: 20A)":i32, "V Range (6: 600V)":i32, "Power VISA Yokogawa WT210":refnum<visa-resource-name>}, "WT500":cluster{"Power VISA Yokogawa WT500":refnum<visa-resource-name>, "V Range (8: 1000V)":i32, "I Range (7: 40A)":i32, "Update Rate (3: 500ms)":i32}, "WT310_2":cluster{"Sample Rate (1: 0.25s)":i32, "A Range (12: 20A)":i32, "V Range (6: 600V)":i32, "Power VISA Yokogawa WT310_2":refnum<visa-resource-name>}, "WT310_3":cluster{"Sample Rate (1: 0.25s)":i32, "A Range (12: 20A)":i32, "V Range (6: 600V)":i32, "Power VISA Yokogawa WT310_3":refnum<visa-resource-name>}}
  T64 = cluster{"Aplus IP Address":string, "Remote Port":i32, "Instrument":string, "Instr Driver Revision":string}
  T65 = typedef "DOE Front Panel Controls.ctl" = cluster{"Test Stand Name (General)":string, "Power Analyzer":string, "Scan Rate (Sec)":dbl, "Auto Terminate Power Limit (Watts)":dbl, "Time Limit At Power Level (Seconds)":dbl, "Hot Water Estimated Water Usage (Gallons)":dbl, "Cold Water Estimated Water Usage (Gallons)":dbl, "Analog DAQ":string, "Flow Rates":string, "Scale":string, "Dishwasher Events Visible":bool, "Rinse Button Enabled":bool, "Final RMC Enabled":bool, "Reset Cold Laurel Meter Enabled":bool, "Laurel Communication Type":string, "Agilent Gain":dbl, "Station Name (Specific)":string, "TC Type (K,J)":string, "Max File Size":dbl, "Reset Hot Laurel Meter Enabled":bool, "Use Chroma?":bool, "Standby Power Enabled":bool, "Reset Power Meter Enabled":bool, "Use Heise Barometric Pressure":bool, "Enable Dryer PreCondition":bool, "Cycles Per Year":u32}
  T66 = cluster{"Agilent 34972_1":refnum<visa-resource-name>, "Agilent 34972_2":refnum<visa-resource-name>, "Agilent 34972_3":refnum<visa-resource-name>, "Agilent 34972_4":refnum<visa-resource-name>, "Agilent 34972_5":refnum<visa-resource-name>, "Agilent 34972_6":refnum<visa-resource-name>, "Agilent Gain":dbl, "TC Type (K,J,T)":string, "Instrument IDN?":string, "TC Channels-List":string, "Analog Channels-List":string, "Agilent Cluster Array":T12[], "TC Channels-List 2":string, "Analog Channels-List 2":string}
  T67 = typedef "Advantech DAQ.ctl" = cluster{"Cold Water Pressure":dbl, "Hot Water Pressure":dbl, "Cold Water Temp":dbl, "Hot Water Temp":dbl, "Ambient Temp":dbl, "Room Humidity":dbl, "Scale (lbs)":dbl, "RPM":dbl, "Cold Water Temp-Avg":dbl, "Hot Water Temp-Avg":dbl, "Cold Water Pressure-Avg":dbl, "Hot Water Pressure-Avg":dbl}
  T68 = typedef "iBTHX Data Values.ctl" = cluster{"iBTHX Barometric Pressure (mbar/hPa)":dbl, "iBTHX Humidity (%)":dbl, "iBTHX Temperature (°F)":dbl, "iBTHX DewPoint Temp":dbl}
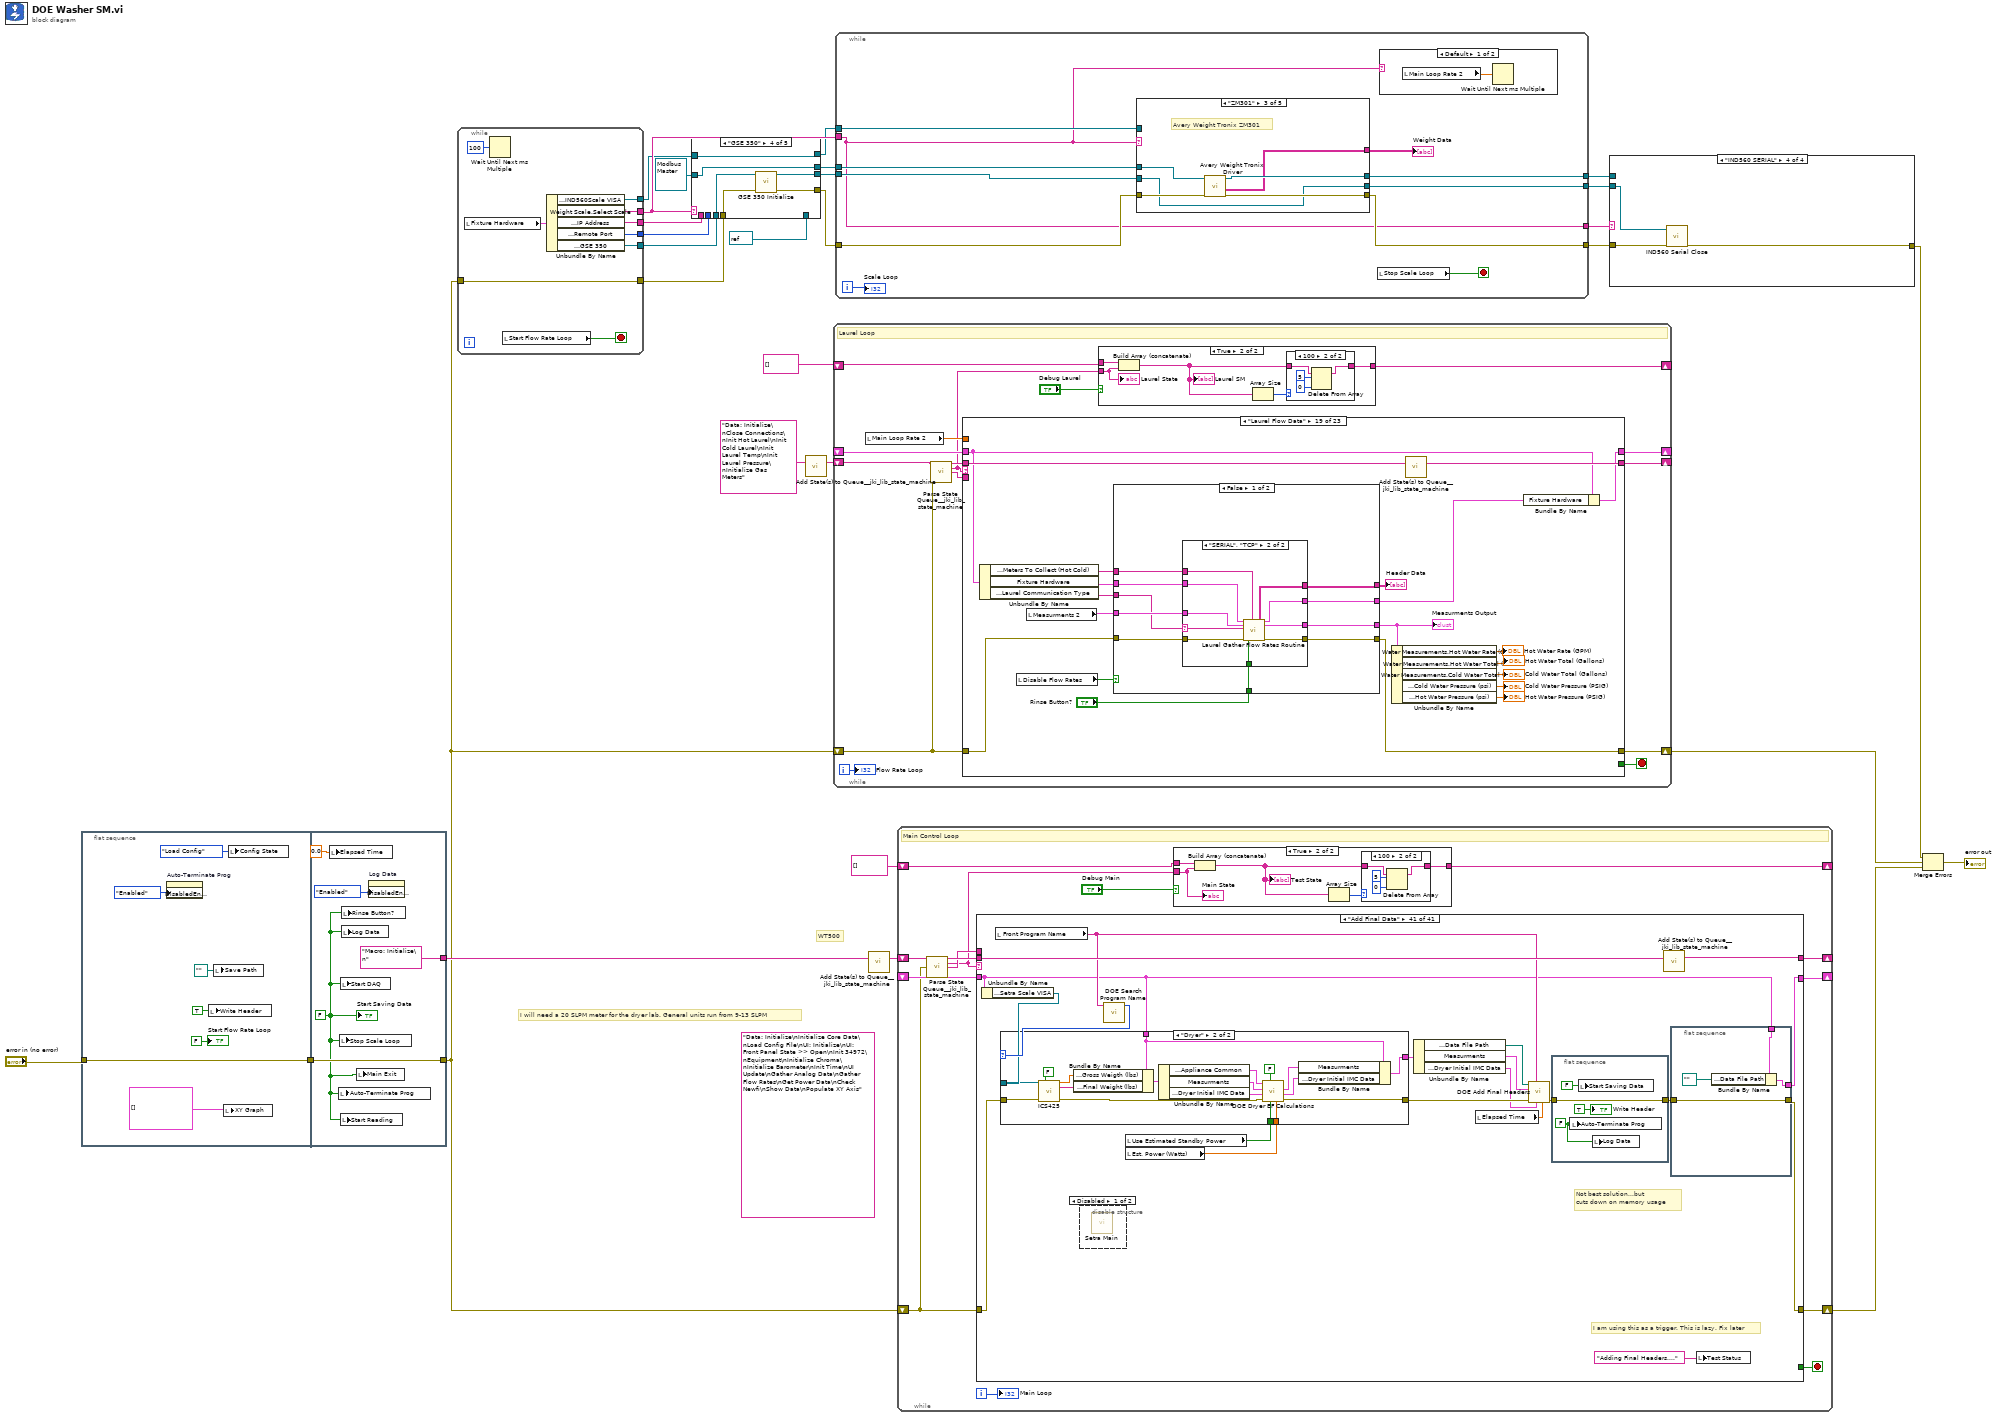
[diagram p0: block diagram]
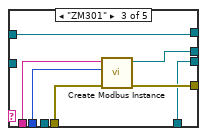
[diagram p4: hidden frame]
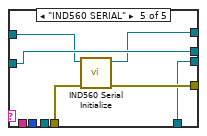
[diagram p5: hidden frame]
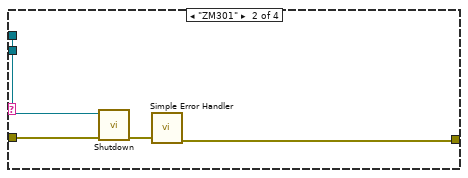
[diagram p7: hidden frame]
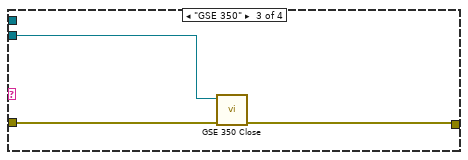
[diagram p8: hidden frame]
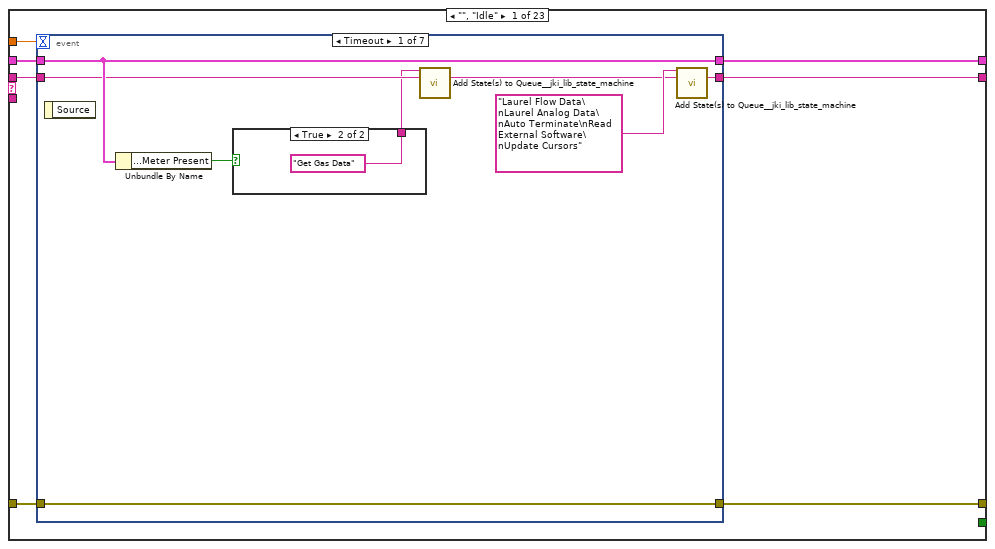
[diagram p11: hidden frame]
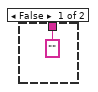
[diagram p12: hidden frame]
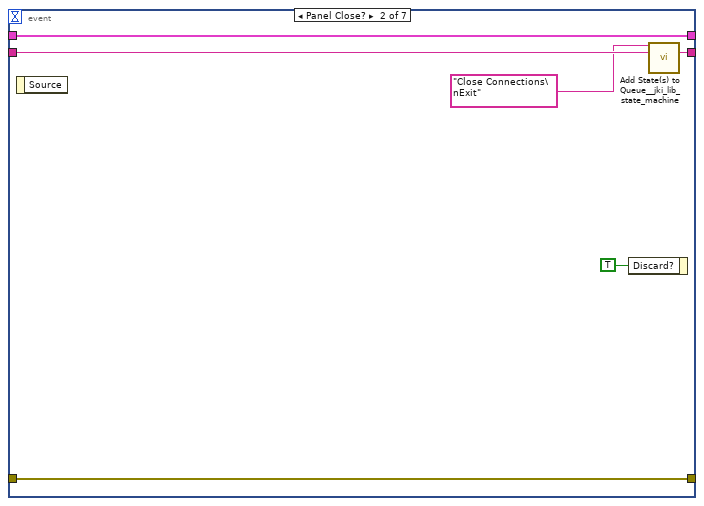
[diagram p13: hidden frame]
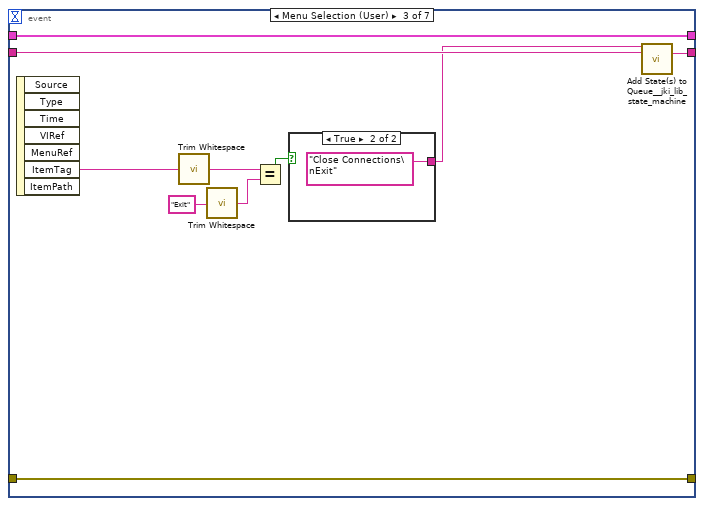
[diagram p14: hidden frame]
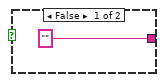
[diagram p15: hidden frame]
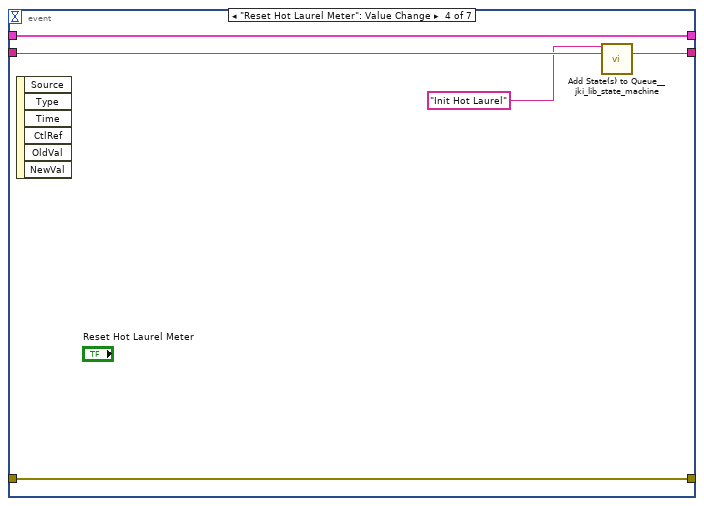
[diagram p16: hidden frame]
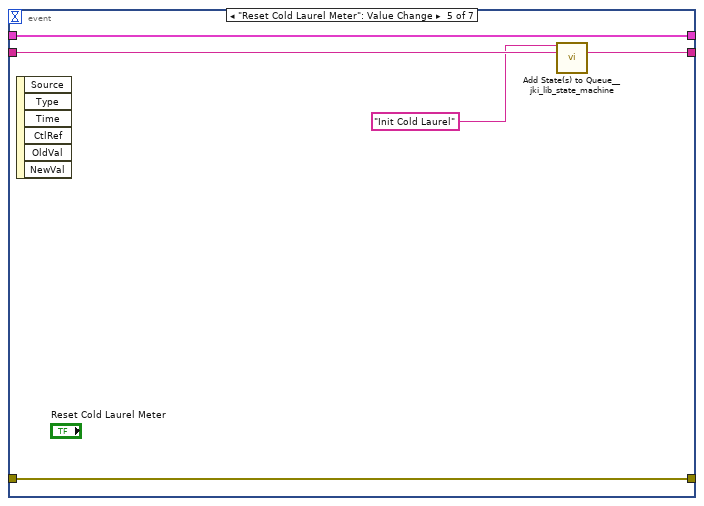
[diagram p17: hidden frame]
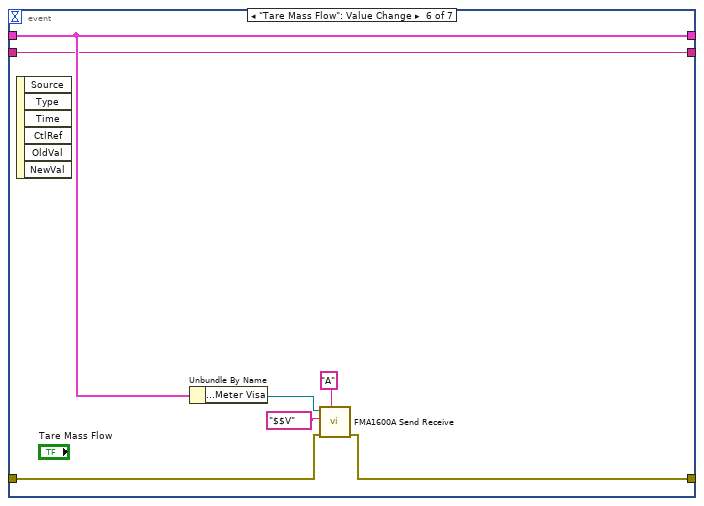
[diagram p18: hidden frame]
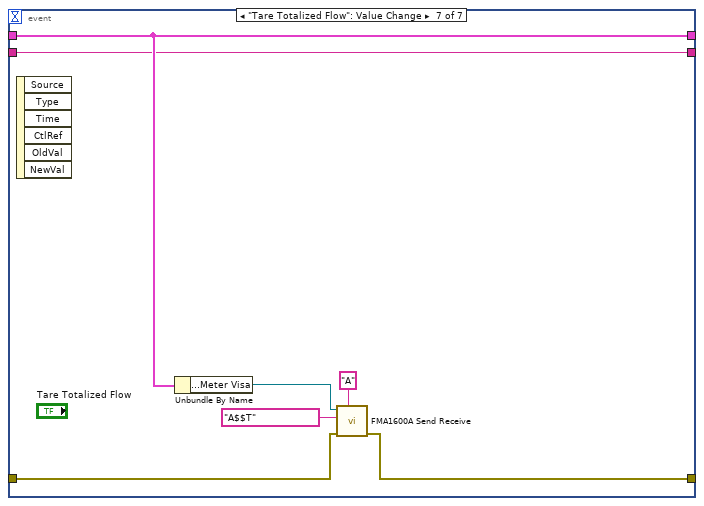
[diagram p19: hidden frame]
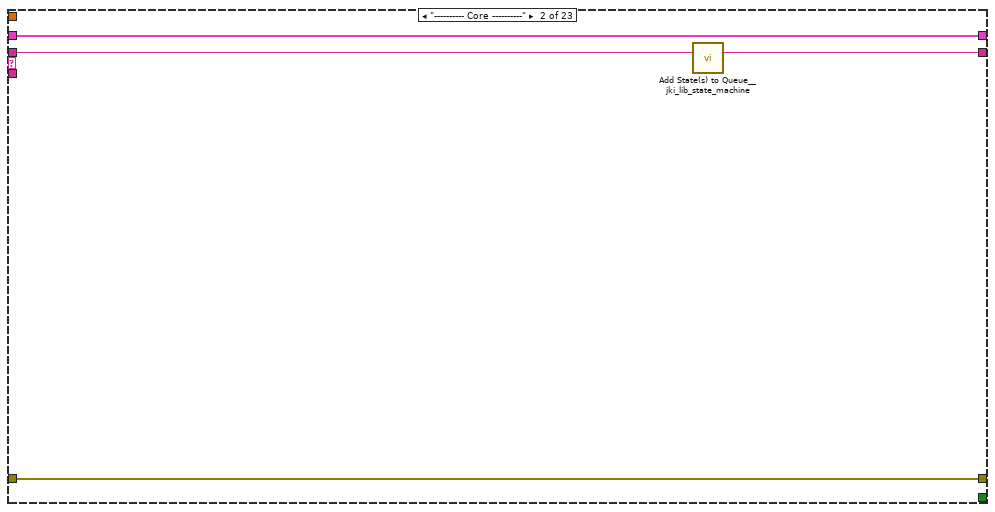
[diagram p20: hidden frame]
diagram:
  (unwired) "Data: Initialize\nInitialize Core Data\nLoad Config File\nUI: Initialize\nUI: Front Panel State >> Open\nInit 34972\nEquipment\nInitialize Chroma\nInitialize Barometer\nInit Time\nUI Update\nGather Analog Data\nGather Flow Rates\nGet Power Data\nCheck Newfi\nShow Data\nPopulate XY Axis"
  # "I will need a 20 SLPM meter for the dryer lab. General units run from 9-13 SLPM"
  # "WT500"
  n1 = flat-sequence {
    tunnel: [w36] -> w27
    tunnel: "error in (no error)" -> [w36]
    tunnel: ["Macro: Initialize\n"] -> w28
    tunnel: w27 -> [w40]
    tunnel: [w40] -> w11
    frame #0 {
      n2 = property on="Auto-Terminate Prog" class="Bool (strict)"("DisabledEnum"=T45."Enabled" ("Disabled")) -> ()  [unwired: 2 in, 2 out]
      n3 = local write "Write Header"(TRUE ("Write Header")) -> ()
      n4 = local write "Save Path"(path "" ("Save Path")) -> ()
      n5 = local write "XY Graph"(T3 [] ("XY Graph")) -> ()
      n6 = local write "Config State"(Save_File_DOE_Configuration_State."Load Config" ("Config State")) -> ()
      "Start Flow Rate Loop" <- FALSE ("Start Flow Rate Loop")
    }
    frame #1 {
      w37 = FALSE ("Start ERD")
      n7 = local write "Elapsed Time"(0.0 ("Total Gallons")) -> ()
      n8 = local write "Auto-Terminate Prog"(w37) -> ()
      n9 = local write "Stop Scale Loop"(w37) -> ()
      n10 = local write "Start DAQ"(w37) -> ()
      n11 = local write "Start Reading"(w37) -> ()
      n12 = local write "Rinse Button?"(w37) -> ()
      n13 = local write "Log Data"(w37) -> ()
      n14 = local write "Main Exit"(w37) -> ()
      n15 = property on="Log Data" class="Bool (strict)"("DisabledEnum"=T45."Enabled" ("Disabled")) -> ()  [unwired: 2 in, 2 out]
      "Start Saving Data" <- w37
    }
  }
  n16 = while {
    tunnel: w11 -> [w48]
    tunnel: [w48] -> w7
    tunnel: [w46] -> w14
    tunnel: [w45] -> w16
    tunnel: [w44] -> w15
    tunnel: [w43] -> w2
    tunnel: [w42] -> w8
    stop <- w50 stop-if-true
    n17 = local read "Fixture Hardware"() -> (w47:T9)
    n18 = Wait Until Next ms Multiple(millisecond multiple=u32 100) -> ()  [unwired: 1 out]
    n19 = local read "Start Flow Rate Loop"() -> (w50:bool)
    n20 = Unbundle By Name(w47) -> ("Weight Scale.Com Options.IND560Scale VISA"=w43:refnum<visa-resource-name>, "Weight Scale.Select Scale"=w46:string, "Weight Scale.Com Options.IP Address"=w45:string, "Weight Scale.Com Options.Remote Port"=w44:u16, "Weight Scale.Com Options.GSE 350"=w42:refnum<visa-resource-name>)
  }
  n21 = case shown="\"GSE 350\"" w14 {
    tunnel: w16 -> [_ _ w65 _ _]
    tunnel: w15 -> [_ _ w64 _ _]
    tunnel: [w54 w58 w63 w71 w75] -> w13
    tunnel: refnum<class "Modbus Master.lvclass"> refnum ("TCP master instance") -> [w54 w58 _ w71 w75]
    tunnel: w8 -> [_ _ _ w70 _]
    tunnel: w7 -> [w53 w57 w62 w69 w77]
    tunnel: [w53 w57 w61 w68 w76] -> w6
    tunnel: [w52 w56 w60 w67 w72] -> w5
    tunnel: refnum<visa-resource-name> refnum ("VISA Refnum out") -> [w52 w56 w60 _ w72]
    tunnel: w2 -> [w51 w55 w59 w66 w74]
    tunnel: [w51 w55 w59 w66 w73] -> w1
    frame Default {
    }
    frame "IND560" {
    }
    frame "ZM301" {
      n22 = call-poly <vilib>:"Create Modbus Instance.vi"("error in"=w62, "port (502)"=w64, "address"=w65) -> ("error out"=w61:errorcluster, "TCP master instance"=w63:refnum<class "Modbus Master.lvclass">)  [unwired: 7 in]
    }
    frame "GSE 350" {
      n23 = call "GSE 350 Initialize.vi"("error in (no error)"=w69, "VISA Refnum in"=w70) -> ("error out"=w68:errorcluster, "VISA Refnum out"=w67:refnum<visa-resource-name>)  [unwired: 8 in]
    }
    frame "IND560 SERIAL" {
      n24 = call "IND560 Serial Initialize.vi"("Error In"=w77, "VISA Refnum in"=w74) -> ("Error Out"=w76:errorcluster, "VISA Refnum Out"=w73:refnum<visa-resource-name>)  [unwired: 8 in]
    }
  }
  n25 = call <vilib>:"Add State(s) to Queue__jki_lib_state_machine.vi"("State(s) in (\"\")"="Data: Initialize\nClose Connections\nInit Hot Laurel\nInit Cold Laurel\nInit Laurel Temp\nInit Laurel Pressure\nInitialize Gas Meters") -> ("States Out"=w23:string)  [unwired: 14 in]
  n26 = while "JKI - String-Based Queued State Machine (Basic) v1.0" {
    shift-right: [w86] -> _
    shift-left: _ -> [w85]
    shift-right: [w89] -> w20
    shift-left: w11 -> [w84]
    shift-right: [w88] -> _
    shift-left: w23 -> [w90]
    shift-right: [w79] -> _
    shift-left: string[] [] -> [w81]
    i -> [w82]
    stop <- w87 stop-if-true
    # "Laurel Loop"
    n27 = local read "Main Loop Rate 2"() -> (w83:T35)
    n28 = call <vilib>:"Parse State Queue__jki_lib_state_machine.vi"("State Queue"=w90, "Error In (no error)"=w84) -> ("Remaining States"=w92:string, "Current State"=w80:string, "Arguments"=w91:string)  [unwired: 11 in]
    n29 = case shown="\"Laurel Flow Data\"" w80 {
      selector: w80 -> [_ _ w167 _ _ _ _ _ _ _ _ _ _ _ _ _ _ _ _ _ _ _ _]
      tunnel: w92 -> [w110 w166 w171 w183 w186 w192 w199 w208 w212 w222 w248 w266 w286 w302 w318 w322 w326 w339 w359 w403 w430 w452 w489]
      tunnel: w91 -> [_ _ _ _ _ _ _ _ _ _ _ _ _ _ _ _ _ _ _ _ _ _ _]
      tunnel: w85 -> [w108 w163 w169 w180 w187 w189 _ w205 w210 w214 w244 w261 w279 w298 w311 w319 w323 w330 w350 w398 w427 w449 w486]
      tunnel: [w107 w164 w173 errorcluster {"status"=FALSE, "code"=0, "source"=""} ("error out") w184 w190 w196 w206 w209 w215 w245 w262 w277 w299 w314 w320 w324 w331 w352 w399 w428 w450 w487] -> w89
      tunnel: w84 -> [w106 w164 w172 w179 w184 w190 w196 w206 w209 w216 w246 w263 w278 w300 w315 w320 w324 w332 w353 w400 w428 w450 w487]
      tunnel: [w109 w165 w170 w182 w185 w191 w198 w207 w211 w221 w247 w265 w285 w301 w317 w321 w325 w338 w358 w402 w429 w451 w488] -> w88
      tunnel: [_ _ _ _ w188 _ _ _ _ _ _ _ _ _ _ _ _ _ _ _ _ _ _] -> w87
      tunnel: [w105 w163 w169 w180 w187 w189 w197 w205 w210 w214 w243 w260 w279 w298 w310 w319 w323 w329 w349 w398 w427 w449 w486] -> w86
      tunnel: w83 -> [w104 _ _ _ _ _ _ _ _ _ _ _ _ _ _ _ _ _ _ _ _ _ _]
      frame "", "Idle" {
        n30 = event shown="[0] Timeout" {
          selector: _ -> [_ _ _ _ _ _ _]
          dyn-events: _ -> [_ _ _ _ _ _ _]
          timeout: w104 -> [_ _ _ _ _ _ _]
          tunnel: w110 -> [w114 w126 w134 w142 w146 w149 w156]
          tunnel: [w118 w125 w135 w141 w147 w149 w156] -> w109
          tunnel: w108 -> [w115 w123 w136 w143 w148 w150 w157]
          tunnel: [w117 w124 w127 w140 w145 w152 w159] -> w107
          tunnel: w106 -> [w117 w124 w127 w140 w145 w153 w160]
          tunnel: [w115 w123 w136 w143 w148 w150 w157] -> w105
          event Timeout {
            n31 = event-data() -> ()  [unwired: 1 in, 1 out]
            n32 = Unbundle By Name(w115) -> ("DAQ Data In.Meter 1.Meter Present"=w112:bool)
            n33 = case shown="True" w112 {
              tunnel: ["" ("State(s) in Front (\"\")") "Get Gas Data" ("State(s) in Front (\"\")")] -> w111
              frame False {
              }
              frame True {
              }
            }
            n34 = call <vilib>:"Add State(s) to Queue__jki_lib_state_machine.vi"("State(s) in Front (\"\")"=w111, "State(s) in (\"\")"=w114) -> ("States Out"=w113:string)  [unwired: 13 in]
            n35 = call <vilib>:"Add State(s) to Queue__jki_lib_state_machine.vi"("State(s) in Front (\"\")"="Laurel Flow Data\nLaurel Analog Data\nAuto Terminate\nRead External Software\nUpdate Cursors" ("State(s) in Front (\"\")"), "State(s) in (\"\")"=w113) -> ("States Out"=w118:string)  [unwired: 13 in]
          }
          event Panel Close? {
            n36 = event-data() -> ()  [unwired: 1 in, 1 out]
            n37 = event-data("Discard?"=TRUE) -> ()  [unwired: 1 in, 1 out]
            n38 = call <vilib>:"Add State(s) to Queue__jki_lib_state_machine.vi"("State(s) in Front (\"\")"="Close Connections\nExit", "State(s) in (\"\")"=w126) -> ("States Out"=w125:string)  [unwired: 13 in]
          }
          event Menu Selection (User) {
            n39 = event-data() -> ("ItemTag"=w128:string)  [unwired: 1 in, 6 out]
            n40 = call <vilib>:"Trim Whitespace.vi"("string"=w128) -> ("trimmed string"=w131:string)  [unwired: 1 in]
            n41 = call <vilib>:"Trim Whitespace.vi"("string"="Exit") -> ("trimmed string"=w132:string)  [unwired: 1 in]
            n42 = Equal?(x=w131, y=w132) -> (x = y?=w133:bool)
            n43 = case shown="True" w133 {
              tunnel: ["" "Close Connections\nExit"] -> w129
              frame False {
              }
              frame True {
              }
            }
            n44 = call <vilib>:"Add State(s) to Queue__jki_lib_state_machine.vi"("State(s) in Front (\"\")"=w129, "State(s) in (\"\")"=w134) -> ("States Out"=w135:string)  [unwired: 13 in]
          }
          event "Reset Hot Laurel Meter": Value Change {
            n45 = event-data() -> ()  [unwired: 1 in, 6 out]
            n46 = call <vilib>:"Add State(s) to Queue__jki_lib_state_machine.vi"("State(s) in Front (\"\")"="Init Hot Laurel" ("State(s) in Front (\"\")"), "State(s) in (\"\")"=w142) -> ("States Out"=w141:string)  [unwired: 13 in]
          }
          event "Reset Cold Laurel Meter": Value Change {
            n47 = event-data() -> ()  [unwired: 1 in, 6 out]
            n48 = call <vilib>:"Add State(s) to Queue__jki_lib_state_machine.vi"("State(s) in Front (\"\")"="Init Cold Laurel" ("State(s) in Front (\"\")"), "State(s) in (\"\")"=w146) -> ("States Out"=w147:string)  [unwired: 13 in]
          }
          event "Tare Mass Flow": Value Change {
            n49 = event-data() -> ()  [unwired: 1 in, 6 out]
            n50 = Unbundle By Name(w150) -> ("DAQ Data In.Meter 1.Meter Visa"=w151:refnum<visa-resource-name>)
            n51 = call "FMA1600A Send Receive.vi"("Unit ID"="A", "error in (no error)"=w153, "FMA1600A Commands"=T46 "$$V", "VISA Refnum in"=w151) -> ("error out"=w152:errorcluster)  [unwired: 5 in, 2 out]
          }
          event "Tare Totalized Flow": Value Change {
            n52 = event-data() -> ()  [unwired: 1 in, 6 out]
            n53 = Unbundle By Name(w157) -> ("DAQ Data In.Meter 1.Meter Visa"=w158:refnum<visa-resource-name>)
            n54 = call "FMA1600A Send Receive.vi"("Unit ID"="A", "error in (no error)"=w160, "FMA1600A Commands"=T46 "A$$T", "VISA Refnum in"=w158) -> ("error out"=w159:errorcluster)  [unwired: 5 in, 2 out]
          }
        }
      }
      frame "---------- Core ----------" {
        n55 = call <vilib>:"Add State(s) to Queue__jki_lib_state_machine.vi"("State(s) in (\"\")"=w166) -> ("States Out"=w165:string)  [unwired: 14 in]
      }
      frame Default {
        w176 = 42 items=["No error", "Argument error", "Memory is full", "Out of zone", "End of file", "File already open", "Generic file I/O error", "File not found", "File permission error", "Disk is full", "Duplicate path", "Too many files open", "System feature not enabled", "Resource file not found", "Cannot add resource", "Resource not found", "Image not found", "Image memory error", "Pen does not exist", "Config type invalid", "Config token not found", "Config parse error", "Config memory error", "Bad external code format", "Bad external code offset", "External code not present", "Null window", "Destroy window error", "Null menu", "Print aborted", "Bad print record", "Print driver error", "Windows error during printing", "Memory error during printing", "Print dialog error", "Generic print error", "Invalid device refnum", "Device not found", "Device parameter error", "Device unit error", "Cannot open device", "Device call aborted", "Generic error", "Cancelled by user", "Object ID too low", "Object ID too high", "Object not in heap", "Unknown heap", "Unknown object (invalid DefProc)", "Unknown object (DefProc not in table)", "Message out of range", "Invalid (null) method", "Unknown message", "Manager call not supported", "Bad address", "Network operation in progress", "Network operation timed out", "Connection is busy", "Network attribute not supported", "Network error", "Address in use", "System out of memory", "Connection aborted", "Connection refused", "Not connected", "Already connected", "Connection closed", "Initialization error (interapplication manager)", "Bad occurrence", "Wait on unbound occurrence handler", "Occurrence queue overflow", "Datalog type conflict", "Unused", "Unrecognized type (interapplication manager)", "Memory corrupt", "Failed to make temporary DLL", "Old CIN version", "Drag socket not found", "Failed to load drop-object", "Failed to register OLE object", "Failed to release OLE object", "Format specifier type mismatch", "Unknown format specifier", "Too few format specifiers", "Too many format specifiers", "Scan failed", "Newer CIN version", "Error converting to variant", "Runtime menu error", "Password tampered", "Variant attribute not found", "Incompatible variant data type", "Event data is not available", "Event Store is not present", "Occurrence is not found", "Event Queue is not created", "Event info is not available", "Refnum passed is NULL", "Error retrieving Class GUID", "Error retrieving CoClass GUID", "Error retrieving TypeLib GUID.", "Bad built application magic bytes.", "Specific driver is different from the specific driver associated with the Logical Name.", "There is no session opened to the class driver.", "Max Error", "MAX - Error with config objects", "MAX - Error loading configuration", "MAX - Group not supported"]
        # "Current State"
        # "Handle mistyped state name (developer tool)"
        n56 = Format Into String(format string="Software Exception: Unhandled State \"%s\"." ("message"), error in=w172, w167) -> (resulting string=w175:string, error out=w174:errorcluster)  [unwired: 1 in]
        n57 = call <vilib>:"Error Cluster From Error Code.vi"("show call chain? (False)"=TRUE, "error in (no error)"=w174, "error message (\"\")"=w175, "error code (0)"=w176) -> ("error out"=w173:errorcluster)  [unwired: 5 in]
        n58 = call <vilib>:"Add State(s) to Queue__jki_lib_state_machine.vi"("State(s) in (\"\")"=w171) -> ("States Out"=w170:string)  [unwired: 14 in]
      }
      frame "Error Handler" {
        # "Unhandled Error -- Display it"
        # "Handle any errors here.\nYou can also output any states to clean-up after errors occur"
        # "Clear error"
        n59 = call <vilib>:"General Error Handler.vi"("error in (no error)"=w179) -> ()  [unwired: 10 in, 5 out]
        n60 = call <vilib>:"Add State(s) to Queue__jki_lib_state_machine.vi"("State(s) in Front (\"\")"="/* Post Error States", "State(s) in (\"\")"=w183) -> ("States Out"=w182:string)  [unwired: 13 in]
      }
      frame "Exit" {
        w188 = TRUE
        n61 = call <vilib>:"Add State(s) to Queue__jki_lib_state_machine.vi"("State(s) in (\"\")"=w186) -> ("States Out"=w185:string)  [unwired: 14 in]
        "Stop Scale Loop" <- w188
      }
      frame "---------- Data ----------" {
        n62 = call <vilib>:"Add State(s) to Queue__jki_lib_state_machine.vi"("State(s) in (\"\")"=w192) -> ("States Out"=w191:string)  [unwired: 14 in]
      }
      frame "Data: Initialize" {
        n63 = while {
          tunnel: [w202] -> w195
          tunnel: [w201] -> w194
          tunnel: ["DAQ Data In"] -> w193
          stop <- w204 stop-if-true
          n64 = local read "Front Program Name"() -> (w203:string)
          n65 = local read "Start Flow Rate Loop"() -> (w204:bool)
          n66 = local read "Fixture Hardware"() -> (w201:T9)
          n67 = call "DOE Search Program Name.vi"("Program Name"=w203) -> ("LV Program"=w202:T49)  [unwired: 10 in]
        }
        n68 = Bundle("LV Program"=w195, "Fixture Hardware"=w194, "DAQ Data In"=w193) -> (w197:T50)  [unwired: 1 in]
        n69 = call <vilib>:"Add State(s) to Queue__jki_lib_state_machine.vi"("State(s) in (\"\")"=w199) -> ("States Out"=w198:string)  [unwired: 14 in]
      }
      frame "---------- UI ----------" {
        n70 = call <vilib>:"Add State(s) to Queue__jki_lib_state_machine.vi"("State(s) in (\"\")"=w208) -> ("States Out"=w207:string)  [unwired: 14 in]
      }
      frame "UI: Initialize" {
        n71 = call <vilib>:"Add State(s) to Queue__jki_lib_state_machine.vi"("State(s) in (\"\")"=w212) -> ("States Out"=w211:string)  [unwired: 14 in]
      }
      frame "Close Connections" {
        n72 = Unbundle By Name(w214) -> ("Fixture Hardware.Flow Rates.Laurel Communication Type"=w217:string, "Fixture Hardware.Flow Rates.Meters To Collect (Hot Cold)"=w213:string)
        n73 = call <vilib>:"Trim Whitespace.vi"("string"=w213) -> ("trimmed string"=w219:string)  [unwired: 1 in]
        n74 = String Length(string=w219) -> (length=w220:i32)
        n75 = Greater Than 0?(x=w220) -> (x > 0?=w218:bool)
        n76 = case shown="True" w218 {
          tunnel: [w223 w227] -> w215
          tunnel: w217 -> [_ w226]
          tunnel: w216 -> [w223 w225]
          tunnel: w214 -> [_ w224]
          frame False {
          }
          frame True {
            n77 = case shown="\"TCP\"" w226 {
              tunnel: [w239 w240] -> w227
              tunnel: w225 -> [_ w240]
              tunnel: w224 -> [w230 _]
              frame "SERIAL", Default {
                w236 = T51 4 items=["VISA Defaults"=0, "Exclusive Lock"=1, "Load Configured Settings"=4] ("Access Mode")
                w237 = T51 4 items=["VISA Defaults"=0, "Exclusive Lock"=1, "Load Configured Settings"=4] ("Access Mode")
                n78 = Unbundle By Name(w230) -> ("Fixture Hardware.Flow Rates.Hot Water Laurel VISA"=w229:refnum<visa-resource-name>, "Fixture Hardware.Flow Rates.Cold Water Laurel VISA"=w228:refnum<visa-resource-name>)
                n79 = VISA Open(timeout (0)=u32 500 ("VISA Open timeout (0)"), access mode=w237, VISA resource name=w229) -> (error out=w234:errorcluster)  [unwired: 2 in, 1 out]
                n80 = VISA Open(timeout (0)=u32 500 ("VISA Open timeout (0)"), access mode=w236, VISA resource name=w228) -> (error out=w233:errorcluster)  [unwired: 2 in, 1 out]
                n81 = Merge Errors(w234, w233) -> (w232:errorcluster)
                n82 = call <vilib>:"Clear Errors.vi"("error in (no error)"=w232, "specific error code to clear (0: all)"=0) -> ("error out"=w239:errorcluster)  [unwired: 4 in, 1 out]
              }
              frame "TCP" {
              }
            }
          }
        }
        n83 = call <vilib>:"Add State(s) to Queue__jki_lib_state_machine.vi"("State(s) in (\"\")"=w222) -> ("States Out"=w221:string)  [unwired: 14 in]
      }
      frame "Init Hot Laurel" {
        n84 = Unbundle By Name(w244) -> ("Fixture Hardware.Flow Rates.Meters To Collect (Hot Cold)"=w241:string, "Fixture Hardware.Flow Rates.Laurel Communication Type"=w242:string)
        n85 = case shown="Default" w241 {
          tunnel: [w250 w258] -> w245
          tunnel: w246 -> [w250 w251]
          tunnel: w244 -> [w249 w257]
          tunnel: [w249 w257] -> w243
          tunnel: w242 -> [_ w254]
          frame Default {
          }
          frame "HOT", "HOT COLD" {
            n86 = Unbundle By Name(w257) -> ("Fixture Hardware.Flow Rates.Laurel Hot IP Address"=w256:string, "Fixture Hardware.Flow Rates.Hot Water Laurel VISA"=w252:refnum<visa-resource-name>)
            n87 = First Call?() -> (First Call?: T/F=w253:bool)
            n88 = call "Laurel Data GET Top Level.vi"("Laurel IP Address"=w256, "Laurel Serial Commands"=T47 "*1C1", "First Call?"=w253, "Serial VISA"=w252, "error in (no error)"=w251, "Laurel Communication Type"=w254) -> ("error out"=w258:errorcluster)  [unwired: 4 in, 5 out]
          }
        }
        n89 = call <vilib>:"Add State(s) to Queue__jki_lib_state_machine.vi"("State(s) in (\"\")"=w248) -> ("States Out"=w247:string)  [unwired: 14 in]
      }
      frame "Init Cold Laurel" {
        n90 = Unbundle By Name(w261) -> ("Fixture Hardware.Flow Rates.Meters To Collect (Hot Cold)"=w259:string, "Fixture Hardware.Flow Rates.Laurel Communication Type"=w264:string)
        n91 = case shown="Default" w259 {
          tunnel: [w268 w274] -> w262
          tunnel: w264 -> [_ w276]
          tunnel: w263 -> [w268 w275]
          tunnel: w261 -> [w267 w273]
          tunnel: [w267 w273] -> w260
          frame Default {
          }
          frame "COLD", "HOT COLD" {
            n92 = Unbundle By Name(w273) -> ("Fixture Hardware.Flow Rates.Laurel Cold IP Address"=w272:string, "Fixture Hardware.Flow Rates.Cold Water Laurel VISA"=w270:refnum<visa-resource-name>)
            n93 = First Call?() -> (First Call?: T/F=w269:bool)
            n94 = call "Laurel Data GET Top Level.vi"("Laurel IP Address"=w272, "Laurel Serial Commands"=T47 "*1C1", "First Call?"=w269, "Serial VISA"=w270, "error in (no error)"=w275, "Laurel Communication Type"=w276) -> ("error out"=w274:errorcluster)  [unwired: 4 in, 5 out]
          }
        }
        n95 = call <vilib>:"Add State(s) to Queue__jki_lib_state_machine.vi"("State(s) in (\"\")"=w266) -> ("States Out"=w265:string)  [unwired: 14 in]
      }
      frame "Init Laurel Temp" {
        w282 = T52 0 items=["both", "start of string", "end of string"] ("location (both)")
        n96 = Unbundle By Name(w279) -> ("Fixture Hardware.Analog Data.Laurel Analog.Laurel IP (Water Temp)"=w280:string)
        n97 = call <vilib>:"Trim Whitespace.vi"("string"=w280, "location (both)"=w282) -> ("trimmed string"=w284:string)
        n98 = String Length(string=w284) -> (length=w283:i32)
        n99 = Greater Than 0?(x=w283) -> (x > 0?=w281:bool)
        n100 = case shown="True" w281 {
          tunnel: w278 -> [w287 w292]
          tunnel: [w287 w291] -> w277
          tunnel: w280 -> [_ w290]
          frame False {
          }
          frame True {
            n101 = call "Laurel Data GET Top Level.vi"("Laurel IP Address"=w290, "Laurel Serial Commands"=T47 "*1C1", "error in (no error)"=w292, "Laurel Communication Type"="TCP") -> ("error out"=w291:errorcluster)  [unwired: 6 in, 5 out]
          }
        }
        n102 = call <vilib>:"Add State(s) to Queue__jki_lib_state_machine.vi"("State(s) in (\"\")"=w286) -> ("States Out"=w285:string)  [unwired: 14 in]
      }
      frame "Init Laurel Pressure" {
        w295 = T52 0 items=["both", "start of string", "end of string"] ("location (both)")
        n103 = Unbundle By Name(w298) -> ("Fixture Hardware.Analog Data.Laurel Analog.Laurel IP (Pressure)"=w293:string)
        n104 = call <vilib>:"Trim Whitespace.vi"("string"=w293, "location (both)"=w295) -> ("trimmed string"=w297:string)
        n105 = String Length(string=w297) -> (length=w296:i32)
        n106 = Greater Than 0?(x=w296) -> (x > 0?=w294:bool)
        n107 = case shown="True" w294 {
          tunnel: w300 -> [w303 w308]
          tunnel: [w303 w307] -> w299
          tunnel: w293 -> [_ w306]
          frame False {
          }
          frame True {
            n108 = call "Laurel Data GET Top Level.vi"("Laurel IP Address"=w306, "Laurel Serial Commands"=T47 "*1C1", "error in (no error)"=w308, "Laurel Communication Type"="TCP") -> ("error out"=w307:errorcluster)  [unwired: 6 in, 5 out]
          }
        }
        n109 = call <vilib>:"Add State(s) to Queue__jki_lib_state_machine.vi"("State(s) in (\"\")"=w302) -> ("States Out"=w301:string)  [unwired: 14 in]
      }
      frame "Initialize Gas Meters" {
        n110 = local read "Filepath"() -> (w313:T38)
        n111 = Unbundle By Name(w313) -> ("General Setup Paths.Tool Base Path"=w312:path)
        n112 = call "RANGE Configuration File.vi"("Debug"=FALSE, "Error In"=w315, "Gas Lab Config File"=w312) -> ("Error Out"=w314:errorcluster, "Meter Data"=w309:T40)  [unwired: 7 in]
        n113 = Bundle By Name(cluster=w311, "DAQ Data In"=w309) -> (w310:T50)
        n114 = call <vilib>:"Add State(s) to Queue__jki_lib_state_machine.vi"("State(s) in (\"\")"=w318) -> ("States Out"=w317:string)  [unwired: 14 in]
      }
      frame "---------- Macro ----------" {
        n115 = call <vilib>:"Add State(s) to Queue__jki_lib_state_machine.vi"("State(s) in (\"\")"=w322) -> ("States Out"=w321:string)  [unwired: 14 in]
      }
      frame "---------- OffLoad Data Collection ----------" {
        n116 = call <vilib>:"Add State(s) to Queue__jki_lib_state_machine.vi"("State(s) in (\"\")"=w326) -> ("States Out"=w325:string)  [unwired: 14 in]
      }
      frame "Get Gas Data" {
        # "I have to do this because the mass flow meter and \nWT500 do not play nice together. It will error out the \nWT500 if the communication is not isolated."
        n117 = Unbundle By Name(w330) -> ("DAQ Data In"=w333:T40)
        n118 = Bundle By Name(cluster=w333, "Meter Bank 1.Panel Data.Heating Value (BTU/ft³)"="Heating Value (BTU/ft³)") -> (w335:T40)
        n119 = call "RANGE Grab Bank Data.vi"("DAQ Data In in"=w335, "Meter Number"=Range_Meter_Bank."Meter Bank 1", "Use Mass Flow Unit Converter?"=FALSE, "Meter Select"=RANGE_Meter_Selector_1-2."Meter 1" ("Meter Bank 1.Panel Data.Meter ID"), "error in (no error)"=w332) -> ("DAQ Data In out"=w328:T40, "error out"=w331:errorcluster)  [unwired: 9 in]
        "DAQ Data Out" <- w328
        n120 = Bundle By Name(cluster=w330, "DAQ Data In"=w328) -> (w329:T50)
        n121 = call <vilib>:"Add State(s) to Queue__jki_lib_state_machine.vi"("State(s) in (\"\")"=w339) -> ("States Out"=w338:string)  [unwired: 14 in]
      }
      frame "Laurel Flow Data" {
        n122 = Unbundle By Name(w350) -> ("Fixture Hardware.Flow Rates.Meters To Collect (Hot Cold)"=w341:string, "Fixture Hardware"=w351:T9, "Fixture Hardware.Flow Rates.Laurel Communication Type"=w342:string)
        n123 = local read "Disable Flow Rates"() -> (w354:bool)
        n124 = local read "Measurments 2"() -> (w357:T26)
        n125 = case shown="False" w354 {
          tunnel: w357 -> [w369 w387]
          tunnel: "Rinse Button?" -> [w368 _]
          tunnel: [w367 w387] -> w347
          tunnel: w353 -> [w366 w386]
          tunnel: [w364 w386] -> w352
          tunnel: [w365 string[][] [] ("Kitchen Flow Data")] -> w355
          tunnel: w351 -> [w363 w385]
          tunnel: [w362 w385] -> w348
          tunnel: w342 -> [w361 _]
          tunnel: w341 -> [w360 _]
          frame False {
            n126 = case shown="\"SERIAL\", \"TCP\"" w361 {
              selector: w361 -> [_ w375]
              tunnel: w369 -> [w373 w378]
              tunnel: w368 -> [_ w383]
              tunnel: [w373 w377] -> w367
              tunnel: w366 -> [w371 w382]
              tunnel: [string[][] [] ("Kitchen Flow Data") w381] -> w365
              tunnel: [w371 w380] -> w364
              tunnel: w363 -> [w370 w379]
              tunnel: [w370 w376] -> w362
              tunnel: w360 -> [_ w374]
              frame Default {
              }
              frame "SERIAL", "TCP" {
                n127 = call "Laurel Gather Flow Rates Routine.vi"("Fixture Hardware"=w379, "Measurments"=w378, "Laurel Communication Type"=w375, "error in (no error)"=w382, "Rinse Button?"=w383, "Collect Meter (HOT,COLD,HOT COLD)"=w374) -> ("Header Data"=w381:string[][], "Fixture Hardware Output"=w376:T9, "Measurments Output"=w377:T26, "error out"=w380:errorcluster)  [unwired: 9 in, 1 out]
              }
            }
          }
          frame True {
          }
        }
        "Measurments Output" <- w347
        "Header Data" <- w355
        n128 = Unbundle By Name(w347) -> ("Water Measurements.Hot Water Rate (GPM)"=→"Hot Water Rate (GPM)":dbl, "Water Measurements.Hot Water Total (Gal)"=→"Hot Water Total (Gallons)":dbl, "Water Measurements.Cold Water Total (Gal)"=→"Cold Water Total (Gallons)":dbl, "Water Measurements.Cold Water Pressure (psi)"=→"Cold Water Pressure (PSIG)":dbl, "Water Measurements.Hot Water Pressure (psi)"=→"Hot Water Pressure (PSIG)":dbl)
        n129 = call <vilib>:"Add State(s) to Queue__jki_lib_state_machine.vi"("State(s) in (\"\")"=w359) -> ("States Out"=w358:string)  [unwired: 14 in]
        n130 = Bundle By Name(cluster=w350, "Fixture Hardware"=w348) -> (w349:T50)
      }
      frame "Laurel Analog Data" {
        w390 = T52 0 items=["both", "start of string", "end of string"] ("location (both)")
        w391 = T52 0 items=["both", "start of string", "end of string"] ("location (both)")
        n131 = Unbundle By Name(w398) -> ("Fixture Hardware.Analog Data.Laurel Analog.Laurel IP (Pressure)"=w388:string, "Fixture Hardware.Analog Data.Laurel Analog.Laurel IP (Water Temp)"=w393:string)
        n132 = call <vilib>:"Trim Whitespace.vi"("string"=w393, "location (both)"=w391) -> ("trimmed string"=w395:string)
        n133 = String Length(string=w395) -> (length=w394:i32)
        n134 = Greater Than 0?(x=w394) -> (x > 0?=w392:bool)
        n135 = case shown="True" w392 {
          tunnel: [w415 w417] -> w401
          tunnel: w393 -> [_ w424]
          tunnel: w400 -> [w415 w423]
          frame False {
          }
          frame True {
            n136 = call "Laurel Data GET Top Level.vi"("Laurel IP Address"=w424, "Laurel Serial Commands"=T47 "*1B1", "Use Delay"=FALSE, "error in (no error)"=w423, "byte count"=8, "Laurel Communication Type"="TCP") -> ("Single Item"=→"Water Temperature":dbl, "error out"=w418:errorcluster)  [unwired: 4 in, 4 out]
            n137 = call <vilib>:"Clear Errors.vi"("error in (no error)"=w418, "specific error code to clear (0: all)"=0) -> ("error out"=w417:errorcluster)  [unwired: 4 in, 1 out]
          }
        }
        n138 = call <vilib>:"Trim Whitespace.vi"("string"=w388, "location (both)"=w390) -> ("trimmed string"=w396:string)
        n139 = String Length(string=w396) -> (length=w397:i32)
        n140 = Greater Than 0?(x=w397) -> (x > 0?=w389:bool)
        n141 = case shown="True" w389 {
          tunnel: w401 -> [w404 w413]
          tunnel: [w404 w405] -> w399
          tunnel: w388 -> [_ w411]
          frame False {
          }
          frame True {
            n142 = call "Laurel Data GET Top Level.vi"("Laurel IP Address"=w411, "Laurel Serial Commands"=T47 "*1B1", "Use Delay"=FALSE, "error in (no error)"=w413, "byte count"=8, "Laurel Communication Type"="TCP") -> ("Single Item"=→"Water Pressure":dbl, "error out"=w406:errorcluster)  [unwired: 4 in, 4 out]
            n143 = call <vilib>:"Clear Errors.vi"("error in (no error)"=w406, "specific error code to clear (0: all)"=0) -> ("error out"=w405:errorcluster)  [unwired: 4 in, 1 out]
          }
        }
        n144 = call <vilib>:"Add State(s) to Queue__jki_lib_state_machine.vi"("State(s) in (\"\")"=w403) -> ("States Out"=w402:string)  [unwired: 14 in]
      }
      frame "Auto Terminate" {
        n145 = local read "Auto-Terminate Prog"() -> (w426:bool)
        n146 = case shown="True" w426 {
          frame False {
          }
          frame True {
            n147 = local read "P:Sigma"() -> (w437:dbl)
            n148 = Less Or Equal?(x=w437, y="Power Limit (Watts)") -> (x <= y?=w435:bool)
            n149 = Not(x=w435) -> (.not. x?=w434:bool)
            n150 = call "UTILITY E-Time.vi"("Reset"=w434) -> ("Elapsed Time (sec)"=w433:dbl)  [unwired: 8 in, 2 out]
            n151 = Greater Or Equal?(x=w433, y="Time Limit At Power Limit (Seconds)") -> (x >= y?=→"Limit Reached":bool)
          }
        }
        n152 = call <vilib>:"Add State(s) to Queue__jki_lib_state_machine.vi"("State(s) in (\"\")"=w430) -> ("States Out"=w429:string)  [unwired: 14 in]
      }
      frame "Read External Software" {
        # "Read data collected from external program"
        n153 = local read "Rinse Button?"() -> (w439:bool)
        n154 = And(x="Use Auto-Rinse Detect", y=w439) -> (x .and. y?=w438:bool)
        n155 = Not Equal?(x="File Path To Read", y=path "") -> (x != y?=w446:bool)
        n156 = And(x="Start Reading", y=w446) -> (x .and. y?=w445:bool)
        n157 = case shown="True" w445 {
          tunnel: [string[][] [] ("Last Recorded Dataset") w465] -> w441
          tunnel: "File Path To Read" -> [_ w464]
          frame False {
          }
          frame True {
            n158 = call "UTILITY Read Get Last Dataset.vi"("File Path Control"=w464) -> ("Last Recorded Dataset"=w465:string[][])  [unwired: 10 in]
          }
        }
        "Standard GEA2" <- w441
        n159 = case shown="True" "Use Auto-Rinse Detect" {
          tunnel: "Column Name" -> [_ w456]
          tunnel: "Condition Name In Column" -> [_ w455]
          tunnel: w441 -> [_ w457]
          tunnel: w438 -> [_ w453]
          frame False {
          }
          frame True {
            # "This keeps the rinse button\npressed after the first time"
            n160 = case shown="True" w453 {
              tunnel: w457 -> [w461 _]
              tunnel: w456 -> [w460 _]
              tunnel: w455 -> [w459 _]
              tunnel: [w458 TRUE ("Condition Found?")] -> w454
              frame False {
                n161 = call "DOE Auto Rinse Detect.vi"("Condition Name In Column"=w459, "Column Name"=w460, "GEA Input Data"=w461) -> ("Condition Found?"=w458:bool)  [unwired: 8 in]
              }
              frame True {
              }
            }
            n162 = local write "Rinse Button?"(w454) -> ()
          }
        }
        n163 = call <vilib>:"Add State(s) to Queue__jki_lib_state_machine.vi"("State(s) in (\"\")"=w452) -> ("States Out"=w451:string)  [unwired: 14 in]
      }
      frame "Update Cursors" {
        n164 = property on="XY Graph" class="XYGraph (strict)"("Active Cursor"=u32 1) -> (error out=w481:errorcluster)  [unwired: 2 in, 1 out]
        n165 = property on="XY Graph" class="XYGraph (strict)"("Active Cursor"=u32 1) -> (error out=w470:errorcluster)  [unwired: 2 in, 1 out]
        n166 = property on="XY Graph" class="XYGraph (strict)"(error in=w481) -> (error out=w480:errorcluster, "Cursor.Cursor Y"=w478:dbl)  [unwired: 1 in, 1 out]
        n167 = property on="XY Graph" class="XYGraph (strict)"(error in=w470) -> (error out=w471:errorcluster, "Cursor.Cursor X"=w473:dbl)  [unwired: 1 in, 1 out]
        n168 = property on="XY Graph" class="XYGraph (strict)"(error in=w480, "Active Cursor"=u32 0) -> (error out=w479:errorcluster)  [unwired: 1 in, 1 out]
        n169 = property on="XY Graph" class="XYGraph (strict)"(error in=w471, "Active Cursor"=u32 0) -> (error out=w472:errorcluster)  [unwired: 1 in, 1 out]
        n170 = property on="XY Graph" class="XYGraph (strict)"(error in=w479) -> ("Cursor.Cursor Y"=w477:dbl)  [unwired: 1 in, 2 out]
        n171 = property on="XY Graph" class="XYGraph (strict)"(error in=w472) -> ("Cursor.Cursor X"=w474:dbl)  [unwired: 1 in, 2 out]
        n172 = Subtract(x=w478, y=w477) -> (x-y=w484:dbl)
        n173 = local read "Main Exit"() -> (w466:bool)
        n174 = Subtract(x=w473, y=w474) -> (x-y=w475:dbl)
        n175 = Absolute Value(x=w484) -> (abs(x)=→"Delta Y":dbl)
        n176 = Absolute Value(x=w475) -> (abs(x)=→"Delta X":dbl)
        n177 = case shown="True" w466 {
          tunnel: ["" ("State(s) in Front (\"\")") "Exit" ("State(s) in Front (\"\")")] -> w467
          frame False {
          }
          frame True {
          }
        }
        n178 = call <vilib>:"Add State(s) to Queue__jki_lib_state_machine.vi"("State(s) in Front (\"\")"=w467, "State(s) in (\"\")"=w489) -> ("States Out"=w488:string)  [unwired: 13 in]
      }
    }
    n179 = case shown="True" "Debug Laurel" {
      tunnel: w80 -> [_ w98]
      tunnel: [w93 w95] -> w79
      tunnel: w81 -> [w93 w97]
      frame False {
      }
      frame True {
        n180 = Build Array (concatenate)(w97, w98) -> (w94:string[])
        "Laurel SM" <- w94
        n181 = Array Size(array=w94) -> (size(s)=w96:i32)
        n182 = case shown="100" w96 {
          tunnel: [w99 w102] -> w95
          tunnel: w94 -> [w99 w103]
          frame 0, Default {
          }
          frame 100 {
            n183 = Delete From Array(array=w103, length=5, index=0) -> (array with subset deleted=w102:string[])  [unwired: 1 out]
          }
        }
        "Laurel State" <- w98
      }
    }
    "Flow Rate Loop" <- w82
  }
  n184 = while {
    tunnel: w6 -> [w496]
    tunnel: [w495] -> w18
    tunnel: [w492] -> w17
    tunnel: w1 -> [w501]
    tunnel: w14 -> [w492]
    tunnel: w13 -> [w500]
    tunnel: [w498] -> w12
    tunnel: w5 -> [w497]
    tunnel: [w494] -> w3
    i -> [w502]
    stop <- w499 stop-if-true
    n185 = case shown="\"ZM301\"" w492 {
      tunnel: w501 -> [_ w512 _ _ w527]
      tunnel: [w507 w511 w517 w524 w525] -> w498
      tunnel: w500 -> [w507 w511 w518 w524 w525]
      tunnel: w497 -> [w505 w510 w514 w523 _]
      tunnel: [w505 w510 w514 w522 w526] -> w494
      tunnel: w496 -> [w506 w509 w516 w521 w530]
      tunnel: [w506 w509 w515 w520 w529] -> w495
      tunnel: [string[][] [] ("Avery Weigth Tronix Data") w508 w513 w519 w528] -> w493
      frame "", Default {
      }
      frame "IND560" {
        n186 = call "Get IND560 Scale Data.vi"("VISA Refnum in"=w512) -> ("IND560 Scale Data"=w508:string[][])  [unwired: 6 in, 4 out]
      }
      frame "ZM301" {
        # "Avery Weight Tronix ZM301"
        n187 = call "Avery Weight Tronix Driver.vi"("error in (no error)"=w516, "Modbus master in"=w518) -> ("error out"=w515:errorcluster, "Avery Weigth Tronix Data"=w513:string[][], "Modbus master out"=w517:refnum<class "Modbus Master.lvclass">)  [unwired: 6 in, 1 out]
      }
      frame "GSE 350" {
        n188 = call "GSE 350 Send Receive.vi"("error in (no error)"=w521, "VISA Refnum in"=w523) -> ("error out"=w520:errorcluster, "Weight Data"=w519:string[][], "VISA Refnum out"=w522:refnum<visa-resource-name>)  [unwired: 4 in, 3 out]
      }
      frame "IND560 SERIAL" {
        n189 = call "IND560 Serial Get Data.vi"("error in (no error)"=w530, "VISA Refnum in"=w527) -> ("error out"=w529:errorcluster, "IND560 Serial Data"=w528:string[][], "VISA Refnum out"=w526:refnum<visa-resource-name>)  [unwired: 6 in, 1 out]
      }
    }
    "Weight Data" <- w493
    n190 = local read "Stop Scale Loop"() -> (w499:bool)
    n191 = case shown="Default" w492 {
      frame Default {
        n192 = local read "Main Loop Rate 2"() -> (w503:T35)
        n193 = Wait Until Next ms Multiple(millisecond multiple=w503) -> ()  [unwired: 1 out]
      }
      frame "GSE 350" {
      }
    }
    "Scale Loop" <- w502
  }
  n194 = call <vilib>:"Add State(s) to Queue__jki_lib_state_machine.vi"("State(s) in (\"\")"=w28) -> ("States Out"=w29:string)  [unwired: 14 in]
  n195 = while "Main Control Loop" {
    shift-right: [w538] -> _
    shift-left: _ -> [w537]
    shift-right: [w541] -> w24
    shift-left: w11 -> [w536]
    shift-right: [w540] -> _
    shift-left: w29 -> [w542]
    shift-right: [w532] -> _
    shift-left: string[] [] -> [w534]
    i -> [w531]
    stop <- w539 stop-if-true
    # "Main Control Loop"
    n196 = call <vilib>:"Parse State Queue__jki_lib_state_machine.vi"("State Queue"=w542, "Error In (no error)"=w536) -> ("Remaining States"=w544:string, "Current State"=w533:string, "Arguments"=w543:string)  [unwired: 11 in]
    n197 = case shown="\"Add Final Data\"" w533 {
      selector: w533 -> [_ _ w842 _ _ _ _ _ _ _ _ _ _ _ _ _ _ _ _ _ _ _ _ _ _ _ _ _ _ _ _ _ _ _ _ _ _ _ _ _ _]
      tunnel: w544 -> [w568 w840 w845 w863 w870 w875 w879 w891 w925 w942 w956 w961 w967 w982 w995 w1078 w1092 w1113 w1119 w1123 w1168 w1208 w1219 w1248 w1253 w1274 w1317 w1331 w1371 w1568 w1846 w1857 w1878 w1914 w1945 w1963 w1986 w2005 w2045 w2072 w2092]
      tunnel: w543 -> [_ _ _ _ _ _ _ _ _ _ _ _ _ _ _ _ _ _ _ _ _ w1203 w1213 _ _ _ _ _ _ _ _ _ _ _ _ _ _ _ _ _ _]
      tunnel: w537 -> [w566 w837 w841 w854 w867 w873 w876 _ w919 w936 w950 w958 w965 w979 w985 w1076 w1086 w1109 w1114 w1120 w1134 w1206 w1215 w1245 w1250 w1272 w1314 w1320 w1358 w1562 w1842 w1855 w1876 w1911 w1943 w1961 w1980 w2002 w2043 w2069 w2076]
      tunnel: [w565 w838 w847 w860 errorcluster {"status"=FALSE, "code"=0, "source"=""} ("error out") w872 w877 w886 w923 w939 w955 w959 w962 w980 w989 w1073 w1089 w1100 w1115 w1121 w1162 w1204 w1216 w1246 w1251 w1256 w1315 w1324 w1366 w1565 w1832 w1852 w1871 w1912 w1940 w1950 w1984 w1990 w2034 w2070 w2086] -> w541
      tunnel: w536 -> [w564 w838 w846 w860 w866 w872 w877 w882 w924 w941 w955 w959 w966 w980 w992 w1074 w1090 w1101 w1116 w1121 w1164 w1205 w1217 w1246 w1251 w1258 w1315 w1326 w1367 w1566 w1843 w1853 w1872 w1912 w1936 w1958 w1984 w1990 w2035 w2070 w2082]
      tunnel: [w567 w839 w844 w862 w869 w874 w878 w890 w926 w943 w957 w960 w968 w981 w994 w1077 w1091 w1112 w1118 w1122 w1167 w1207 w1218 w1247 w1252 w1273 w1316 w1330 w1370 w1567 w1845 w1856 w1877 w1913 w1944 w1962 w1985 w2004 w2044 w2071 w2091] -> w540
      tunnel: [_ _ _ _ TRUE w871 _ _ _ _ _ _ _ _ _ _ _ _ _ _ _ _ _ _ _ _ _ _ _ _ _ _ _ _ _ _ _ _ _ _ _] -> w539
      tunnel: [w563 w837 w841 w861 w867 w873 w876 w884 w921 w935 w950 w958 w963 w979 w984 w1076 w1086 w1108 w1114 w1120 w1166 w1206 w1215 w1245 w1250 w1272 w1314 w1319 w1361 w1555 w1841 w1854 w1875 w1910 w1942 w1960 w1979 w1994 w2043 w2069 w2085] -> w538
      frame "", "Idle" {
        n198 = call "UTILITY JKI Loop Timer.vi"("Initialize Rate"="Initialize Rate", "K(0.3)"="K(0.3)", "Scan Rate (Seconds)"="Scan Rate (Seconds)") -> ("Rate"=→"Rate":dbl, "New Time"=w561:dbl)  [unwired: 7 in]
        n199 = Multiply(x=T35 1000.0 ("y"), y=w561) -> (x*y=w557:T35)
        "Main Loop Rate 2" <- w557
        n200 = event shown="[9] \"Final Weight\": Value Change" {
          selector: _ -> [_ _ _ _ _ _ _ _ _ _ _ _ _ _ _ _ _ _ _ _ _]
          dyn-events: _ -> [_ _ _ _ _ _ _ _ _ _ _ _ _ _ _ _ _ _ _ _ _]
          timeout: w557 -> [_ _ _ _ _ _ _ _ _ _ _ _ _ _ _ _ _ _ _ _ _]
          tunnel: w568 -> [w588 w610 w619 w639 w646 w655 w661 w672 w677 w686 w694 w707 w712 w725 w739 w744 w767 w773 w787 w805 w815]
          tunnel: [w586 w609 w620 w640 w646 w655 w662 w671 w676 w687 w695 w707 w712 w725 w738 w744 w767 w773 w787 w806 w815] -> w567
          tunnel: w566 -> [w573 w607 w618 w638 w645 w654 w657 w673 w678 w684 w697 w705 w711 w724 w731 w741 w760 w770 w786 w793 w816]
          tunnel: [w576 w608 w616 w641 w647 w653 w663 w674 w679 w680 w696 w706 w713 w726 w735 w742 w761 w774 w788 w800 w812] -> w565
          tunnel: w564 -> [w577 w608 w616 w641 w647 w653 w663 w674 w679 w681 w696 w706 w713 w726 w736 w743 w762 w775 w789 w804 w820]
          tunnel: [w572 w607 w618 w638 w644 w654 w656 w673 w678 w685 w697 w704 w711 w723 w730 w741 w760 w769 w786 w792 w816] -> w563
          event Timeout {
            # "Get the Modbus Scale Data"
            n201 = event-data() -> ()  [unwired: 1 in, 1 out]
            n202 = Unbundle By Name(w573) -> ("Washer Controls Input.Test Fixture Hardware.Weight Scale.Select Scale"=w584:string, "Measurments.Power Measurements.Power (W):Sigma"=w575:dbl)
            n203 = local read "Power Limit (Watts)"() -> (w579:dbl)
            n204 = local read "DAQ Data Out"() -> (w571:T40)
            n205 = call "DOE Check Power Thresholds.vi"("Power (W):Sigma"=w575, "Error In"=w577, "Power Limit (Watts)"=w579, "Wait for Power Threshold"="Wait for Power Threshold") -> ("Error Out"=w576:errorcluster, "Wait for Power Threshold (Output)"=w569:bool, "States"=w574:string)  [unwired: 5 in]
            n206 = Unbundle By Name(w571) -> ("Meter 1.Meter Present"=w570:bool)
            n207 = case shown="False" w569 {
              frame False {
                n208 = property on="Wait for Power Threshold" class="Bool (strict)"("Value"=FALSE ("Wait for Power Threshold")) -> ()  [unwired: 2 in, 2 out]
              }
              frame True {
                n209 = property on="Wait for Power Threshold" class="Bool (strict)"("Value"=TRUE ("Wait for Power Threshold")) -> ()  [unwired: 2 in, 2 out]
              }
            }
            n210 = Equal?(x="" ("y"), y=w584) -> (x = y?=w582:bool)
            n211 = case shown="True" w569 {
              tunnel: ["Save Data" ""] -> w585
              tunnel: w582 -> [w600 _]
              tunnel: [w599 w602] -> w581
              tunnel: w574 -> [_ w602]
              tunnel: w570 -> [w592 _]
              frame False {
                n212 = Not(x=w592) -> (.not. x?=w591:bool)
                n213 = call "DOE States.vi"("Enable RMC Collection"="Enable RMC Collection", "Disable Gas Data"=w591, "Disable Temp/Humidity"="Disable Temp/Humidity", "Disable Power"="Disable Power", "Disable Analog Data"="Disable Analog Data", "Disable Flow Rates"="Disable Flow Rates", "Disable Scale Data"="Disable Scale Data", "Scale Disabled Config"=w600) -> ("States"=w599:string)  [unwired: 3 in]
              }
              frame True {
              }
            }
            n214 = Bundle By Name(cluster=w573, "Wait for Power Threshold (Output)"=w569) -> (w572:T62)
            n215 = local write "Start Flow Rate Loop"(TRUE ("Start Flow Rate Loop")) -> ()
            n216 = call <vilib>:"Add State(s) to Queue__jki_lib_state_machine.vi"("State(s) in Front (\"\")"=w581, "State(s) in (\"\")"=w588) -> ("States Out"=w587:string)  [unwired: 13 in]
            n217 = call <vilib>:"Add State(s) to Queue__jki_lib_state_machine.vi"("State(s) in (\"\")"=w587, "State(s) at Back (\"\")"=w585) -> ("States Out"=w586:string)  [unwired: 13 in]
          }
          event Panel Close? {
            n218 = event-data() -> ()  [unwired: 1 in, 1 out]
            n219 = local read "Start Saving Data"() -> (w605:bool)
            n220 = case shown="True" w605 {
              tunnel: ["Macro: Exit" "Add Final Data\nMacro: Exit"] -> w604
              frame False {
              }
              frame True {
              }
            }
            n221 = call <vilib>:"Add State(s) to Queue__jki_lib_state_machine.vi"("State(s) in Front (\"\")"=w604, "State(s) in (\"\")"=w610) -> ("States Out"=w609:string)  [unwired: 13 in]
            n222 = event-data("Discard?"=TRUE) -> ()  [unwired: 1 in, 1 out]
          }
          event "Reset Power Meter": Value Change {
            # "Allow manual reset of the power meters"
            n223 = event-data() -> ()  [unwired: 1 in, 6 out]
            n224 = Unbundle By Name(w618) -> ("Power Analyzer"=w617:T37, "Washer Controls Input.Test Fixture Hardware.Power.Aplus.Aplus IP Address"=w615:string, "Washer Controls Input.Test Fixture Hardware.Power.Aplus.Remote Port"=w614:i32)
            n225 = case shown="\"APLUS\"" w617 {
              tunnel: w616 -> [_ w625 _ _ _ _ _]
              tunnel: w615 -> [_ w627 _ _ _ _ _]
              tunnel: w614 -> [_ w626 _ _ _ _ _]
              tunnel: ["" "" "Equipment" "Equipment" "Equipment" "" ""] -> w613
              frame "", Default {
              }
              frame "APLUS" {
                n226 = call-poly <vilib>:"Create Modbus Instance.vi"("error in"=w625, "port (502)"=w626, "address"=w627) -> ("error out"=w624:errorcluster, "TCP master instance"=w623:refnum<class "Modbus Master.lvclass">)  [unwired: 7 in]
                n227 = call "APLUS Open Reset Coil.vi"("Reset WattHours"=TRUE, "error in (no error)"=w624, "Modbus Master in"=w623) -> ("error out"=w629:errorcluster, "Modbus Master out"=w630:refnum<class "Modbus Master.lvclass">)  [unwired: 7 in]
                n228 = call-dynamic "Shutdown.vi"("error in"=w629, "Modbus master in"=w630) -> ("error out"=w628:errorcluster)  [unwired: 9 in]
                n229 = call <vilib>:"Simple Error Handler.vi"("error in (no error)"=w628) -> ()  [unwired: 1 in, 8 out]
              }
              frame "WT210", "WT230" {
              }
              frame "WT300", "WT300_1", "WT300_2" {
              }
              frame "WT500" {
              }
              frame "OSI" {
              }
              frame "Debug" {
              }
            }
            n230 = call <vilib>:"Add State(s) to Queue__jki_lib_state_machine.vi"("State(s) in Front (\"\")"=w613, "State(s) in (\"\")"=w619) -> ("States Out"=w620:string)  [unwired: 13 in]
          }
          event "Start Standby Power": Value Change {
            # "Reset the watt hour meter. Then start\nthe standby power test"
            n231 = event-data() -> ()  [unwired: 1 in, 6 out]
            n232 = call <vilib>:"Add State(s) to Queue__jki_lib_state_machine.vi"("State(s) in Front (\"\")"="Off-Standby Mode", "State(s) in (\"\")"=w639) -> ("States Out"=w640:string)  [unwired: 13 in]
          }
          event "Reset Standby Power": Value Change {
            n233 = event-data() -> ()  [unwired: 1 in, 6 out]
            n234 = local write "Standby Power Data"(string[][] [] ("Standby Power Data")) -> ()
            n235 = Bundle By Name(cluster=w645, "Measurments.Standby Power"=T28 {"Standby Power Spreadsheet"=[], "Standby Power - Pia (Watts)"=0.0, "Off Mode Power - Poff (Watts)"=0.0, "Sia hr/yr"=8620.0, "Soff hr/yr"=0.0, "Yearly Energy Etso kWh/yr"=0.0, "Maximum Power (Watts)"=0.0, "Power Variation (%)"=0.0, "Slope (mW/hr)"=0.0, "Final Harmonics-U1 (%)"="", "Final Harmonics-U2 (%)"="", "Energy (Wh)"=0.0}) -> (w644:T62)
          }
          event "Save Standby Power Data": Value Change {
            n236 = event-data() -> ()  [unwired: 1 in, 6 out]
            n237 = local read "Standby Power Data"() -> (w652:string[][])
            n238 = Build Path(base path="Choose Folder", name or relative path="Standby_Power.csv") -> (appended path=w649:path)
            n239 = call-poly <vilib>:"Write Delimited Spreadsheet.vi"("file path (dialog if empty)"=w649, "2D data"=w652, "delimiter (\\t)"="," ("delimiter (\\t)")) -> ()  [unwired: 11 in, 2 out]
          }
          event "Log Data": Value Change {
            # "UI:Initialize repopulates data erased by Get File Info"
            n240 = event-data() -> ("NewVal"=w658:bool)  [unwired: 1 in, 5 out]
            n241 = case shown="True" w658 {
              tunnel: ["Add Final Data" ("State(s) in Front (\"\")") "Get File Info\nEquipment" ("State(s) in Front (\"\")")] -> w659
              tunnel: w657 -> [w664 w668]
              tunnel: [w664 w667] -> w656
              frame False {
              }
              frame True {
                n242 = Bundle By Name(cluster=w668, "Reset Timer"=TRUE) -> (w667:T62)
              }
            }
            n243 = local write "Config State"(Save_File_DOE_Configuration_State."Open Front Panel" ("Config State")) -> ()
            n244 = call <vilib>:"Add State(s) to Queue__jki_lib_state_machine.vi"("State(s) in Front (\"\")"=w659, "State(s) in (\"\")"=w661) -> ("States Out"=w662:string)  [unwired: 13 in]
          }
          event "X-Axis": Value Change {
            n245 = event-data() -> ()  [unwired: 1 in, 6 out]
            n246 = call <vilib>:"Add State(s) to Queue__jki_lib_state_machine.vi"("State(s) in Front (\"\")"="Populate XY Axis", "State(s) in (\"\")"=w672) -> ("States Out"=w671:string)  [unwired: 13 in]
          }
          event "Y-Axis-1", "Y-Axis-2": Value Change {
            n247 = event-data() -> ()  [unwired: 1 in, 6 out]
            n248 = call <vilib>:"Add State(s) to Queue__jki_lib_state_machine.vi"("State(s) in Front (\"\")"="Populate XY Axis", "State(s) in (\"\")"=w677) -> ("States Out"=w676:string)  [unwired: 13 in]
          }
          event "Final Weight": Value Change {
            n249 = event-data() -> ()  [unwired: 1 in, 6 out]
            n250 = Unbundle By Name(w684) -> ("Washer Controls Input.Test Fixture Hardware.Weight Scale.Com Options.Setra Scale VISA"=w683:refnum<visa-resource-name>)
            n251 = disable-structure shown="Disabled" {
              frame Disabled {
                n252 = call "Setra Main.vi"() -> ()  [unwired: 13 in, 3 out]
              }
              frame Enabled {
              }
            }
            n253 = call "ICS425.vi"("VISA resource name"=w683, "Error In"=w681) -> ("Weight Output (string)"=w682:string, "Error Out"=w680:errorcluster)  [unwired: 11 in, 1 out]
            n254 = Bundle By Name(cluster=w684, "Measurments.Weight Scale.Final Weight (lbs)"=w682) -> (w685:T62)
            n255 = call <vilib>:"Add State(s) to Queue__jki_lib_state_machine.vi"("State(s) in (\"\")"=w686) -> ("States Out"=w687:string)  [unwired: 14 in]
          }
          event Menu Selection (User) {
            n256 = event-data() -> ("ItemTag"=w691:string)  [unwired: 1 in, 6 out]
            n257 = call <vilib>:"Trim Whitespace.vi"("string"=w691) -> ("trimmed string"=w690:string)  [unwired: 1 in]
            n258 = call <vilib>:"Trim Whitespace.vi"("string"="Exit") -> ("trimmed string"=w689:string)  [unwired: 1 in]
            n259 = Equal?(x=w690, y=w689) -> (x = y?=w688:bool)
            n260 = case shown="True" w688 {
              tunnel: ["" w699] -> w693
              frame False {
              }
              frame True {
                n261 = local read "Start Saving Data"() -> (w700:bool)
                n262 = case shown="False" w700 {
                  tunnel: ["Macro: Exit" "Add Final Data\nMacro: Exit"] -> w699
                  frame False {
                  }
                  frame True {
                  }
                }
              }
            }
            n263 = call <vilib>:"Add State(s) to Queue__jki_lib_state_machine.vi"("State(s) in Front (\"\")"=w693, "State(s) in (\"\")"=w694) -> ("States Out"=w695:string)  [unwired: 13 in]
          }
          event "Reset Standby Data": Value Change {
            n264 = event-data() -> ()  [unwired: 1 in, 6 out]
            n265 = Bundle By Name(cluster=w705, "Measurments.Standby Power.Standby Power Spreadsheet"=string[][] []) -> (w704:T62)
          }
          event "X-Axis (Standby)", "Y-Axis (Standby)": Value Change {
            n266 = event-data() -> ()  [unwired: 1 in, 6 out]
            n267 = flat-sequence {
              tunnel: w711 -> [w717]
              tunnel: [w716] -> w710
              tunnel: ["X-Axis (Standby)"] -> w709
              tunnel: ["Y-Axis (Standby)"] -> w708
              tunnel: w710 -> [w720]
              tunnel: w709 -> [w719]
              tunnel: w708 -> [w718]
              frame #0 {
                n268 = Unbundle By Name(w717) -> ("Measurments.Standby Power.Standby Power Spreadsheet"=w716:string[][])
              }
              frame #1 {
                n269 = call "Standby Power Analysis.vi"("Y-Axis (Standby)"=w718, "X-Axis (Standby)"=w719, "Standby Power Spreadsheet"=w720) -> ("XY Graph Standby"=→"XY Graph Standby":cluster{dbl[], dbl[]})  [unwired: 7 in, 1 out]
              }
            }
          }
          event "Clear Graph Data": Value Change {
            n270 = event-data() -> ()  [unwired: 1 in, 6 out]
            n271 = Bundle By Name(cluster=w724, "Plot Array"=dbl[][] [[0.0, 0.0, 0.0], [0.0, 0.0, 0.0]]) -> (w723:T62)
          }
          event "Change Headers": Value Change {
            n272 = event-data() -> ()  [unwired: 1 in, 6 out]
            n273 = Unbundle By Name(w731) -> ("Full Data Output"=w733:string[][], "Filepath.General Setup Paths.Tool Base Path"=w737:path)
            n274 = local read "Point File Path"() -> (w727:path)
            n275 = Transpose 2D Array(2D array=w733) -> (transposed array=w732:string[][])
            n276 = call "Dynamic Headers Change Headers.vi"("Point Startup (WasherDOE)"=w727, "Tree Selection"=T53 "1-1", "Error In"=w736, "Tool Base Path"=w737, "Chamber Data"=w732) -> ("Error Out"=w735:errorcluster, "Point File Path"=→"Point File Path":path)  [unwired: 3 in, 2 out]
            n277 = Bundle By Name(cluster=w731, "Force Read Point"=TRUE) -> (w730:T62)
            n278 = call <vilib>:"Add State(s) to Queue__jki_lib_state_machine.vi"("State(s) in (\"\")"=w739) -> ("States Out"=w738:string)  [unwired: 14 in]
          }
          event "Set Parameters": Value Change {
            n279 = event-data() -> ("NewVal"=w740:bool)  [unwired: 1 in, 5 out]
            n280 = case shown="True" w740 {
              tunnel: w743 -> [w745 w756]
              tunnel: [w745 w748] -> w742
              tunnel: w741 -> [_ w752]
              frame False {
              }
              frame True {
                n281 = Unbundle By Name(w752) -> ("Washer Controls Input.Test Fixture Hardware.Power.Power Supply.Chroma 61605"=w751:refnum<visa-resource-name>)
                n282 = call "CHROMA Set Voltage.vi"("Phase"=CHROMA_Phase."P1", "Error In"=w756, "Voltage Setpoint"="L1 Voltage", "CHROMA VISA In"=w751) -> ("Error Out"=w755:errorcluster, "CHROMA VISA Out"=w750:refnum<visa-resource-name>)  [unwired: 6 in]
                n283 = call "CHROMA Set Voltage.vi"("Phase"=CHROMA_Phase."P2", "Error In"=w755, "Voltage Setpoint"="L2 Voltage", "CHROMA VISA In"=w750) -> ("Error Out"=w749:errorcluster, "CHROMA VISA Out"=w747:refnum<visa-resource-name>)  [unwired: 6 in]
                n284 = call "CHROMA Set Frequency.vi"("Error In"=w749, "Frequency"="Frequency", "CHROMA VISA In"=w747) -> ("Error Out"=w748:errorcluster)  [unwired: 7 in, 1 out]
              }
            }
          }
          event "Set Initialization": Value Change {
            n285 = event-data() -> ()  [unwired: 1 in, 6 out]
            n286 = Unbundle By Name(w760) -> ("Washer Controls Input.Test Fixture Hardware.Power.Power Supply.Chroma 61605"=w759:refnum<visa-resource-name>)
            n287 = call "CHROMA Initialize.vi"("Phase Shift Lines"="Phase Shift Lines", "Phase Shift Angle"="Phase Shift Angle", "Error In"=w762, "Voltage Limit"="Voltage Limit", "Voltage Range"="Voltage Range", "CHROMA VISA In"=w759) -> ("Error Out"=w761:errorcluster)  [unwired: 3 in, 2 out]
          }
          event "Power Supply Status": Value Change {
            n288 = event-data() -> ("NewVal"=w771:bool)  [unwired: 1 in, 5 out]
            n289 = Unbundle By Name(w770) -> ("Washer Controls Input.Test Fixture Hardware.Power.Power Supply.Chroma 61605"=w772:refnum<visa-resource-name>)
            n290 = case shown="False" w771 {
              tunnel: w775 -> [w779 w784]
              tunnel: [w778 w783] -> w774
              tunnel: w772 -> [w777 w782]
              tunnel: [w776 w781] -> w768
              frame False {
                n291 = call "CHROMA Set Output State.vi"("Error In"=w779, "Chroma Output State"=CHROMA_Output_State."Chroma OFF", "CHROMA VISA In"=w777) -> ("Error Out"=w778:errorcluster, "CHROMA VISA Out"=w776:refnum<visa-resource-name>)  [unwired: 6 in, 1 out]
              }
              frame True {
                n292 = call "CHROMA Set Output State.vi"("Error In"=w784, "Chroma Output State"=CHROMA_Output_State."Chroma ON", "CHROMA VISA In"=w782) -> ("Error Out"=w783:errorcluster, "CHROMA VISA Out"=w781:refnum<visa-resource-name>)  [unwired: 6 in, 1 out]
              }
            }
            n293 = Bundle By Name(cluster=w770, "Washer Controls Input.Test Fixture Hardware.Power.Power Supply.Chroma 61605"=w768) -> (w769:T62)
          }
          event "Update Calibration": Value Change {
            n294 = event-data() -> ()  [unwired: 1 in, 6 out]
            n295 = Unbundle By Name(w786) -> ("Filepath.General Setup Paths.Calibration File Path"=w790:path)
            n296 = call "Calibration.vi"("error in (no error)"=w789, "Calibration File Path"=w790) -> ("error out"=w788:errorcluster)  [unwired: 8 in, 1 out]
          }
          event "Dryer Pre-Condition": Value Change {
            n297 = event-data() -> ()  [unwired: 1 in, 6 out]
            n298 = Unbundle By Name(w793) -> ("Washer Controls Input.Test Fixture Hardware.Power.Power Supply.Chroma 61605"=w801:refnum<visa-resource-name>, "Washer Controls Input.Test Fixture Hardware"=w794:T9)
            n299 = call "DPT Panel Dryer PreCondition.vi"("Test Fixture Hardware"=w794, "Error In"=w804) -> ("Cold Dryer Weight"=w791:dbl, "Error Out"=w802:errorcluster)  [unwired: 12 in]
            n300 = call "CHROMA Set Output State.vi"("Error In"=w802, "Chroma Output State"=CHROMA_Output_State."Chroma OFF", "CHROMA VISA In"=w801) -> ("Error Out"=w797:errorcluster, "CHROMA VISA Out"=w799:refnum<visa-resource-name>)  [unwired: 6 in, 1 out]
            n301 = local write "Cold Dryer Weight (lbs)"(w791) -> ()
            n302 = Bundle By Name(cluster=w793, "Washer Controls Input.Initialize.Washer In.Appliance Details.Dryer.Dryer Initial IMC Data.Empty Dryer Cold Weigth"=w791) -> (w792:T62)
            n303 = call "UTILITY Delay mS.vi"("Error In"=w797, "milliseconds to wait"=u32 1000) -> ("Error Out"=w796:errorcluster)  [unwired: 13 in]
            n304 = call <vilib>:"Add State(s) to Queue__jki_lib_state_machine.vi"("State(s) in (\"\")"=w805) -> ("States Out"=w806:string)  [unwired: 14 in]
            n305 = call "CHROMA Set Output State.vi"("Error In"=w796, "Chroma Output State"=CHROMA_Output_State."Chroma ON", "CHROMA VISA In"=w799) -> ("Error Out"=w800:errorcluster)  [unwired: 6 in, 2 out]
          }
          event "Set Configuration": Value Change {
            n306 = event-data() -> ()  [unwired: 1 in, 6 out]
            n307 = local read "Wiring (0: 1P2W, 1P2W, 1P2W)"() -> (w821:T6)
            n308 = Unbundle By Name(w816) -> ("Power Analyzer"=w814:T37, "Washer Controls Input.Test Fixture Hardware.Power.Yokogawa.WT500.Power VISA Yokogawa WT500"=w817:refnum<visa-resource-name>)
            n309 = case shown="\"WT500\"" w814 {
              tunnel: w821 -> [_ w830]
              tunnel: w820 -> [w822 w834]
              tunnel: [w822 w835] -> w813
              tunnel: "Update Rate (3: 500ms)" -> [_ w831]
              tunnel: "Crest Factor (0: 3)" -> [_ w823]
              tunnel: w817 -> [_ w832]
              tunnel: "Voltage Range (8: 1000V)" -> [_ w829]
              tunnel: "Current Range (7: 40A)" -> [_ w828]
              tunnel: "Element (0: All)" -> [_ w827]
              tunnel: "Display Format" -> [_ w825]
              frame "", Default {
              }
              frame "WT500" {
                n310 = call "WT500 General Setup.vi"("VISA Refnum in"=w832, "Wiring (0: 1P2W, 1P2W, 1P2W)"=w830, "V Range (8: 1000V)"=w829, "error in (no error)"=w834, "Element (0: All)"=w827, "Display Format"=w825, "Update Rate (3: 500ms)"=w831, "I Range (7: 40A)"=w828, "Reset Wh"=TRUE, "Crest Factor (0: 3)"=w823) -> ("VISA Refnum out"=w826:refnum<visa-resource-name>, "error out"=w833:errorcluster)  [unwired: 5 in, 3 out]
                n311 = call "YKWT500 Start Stop Integration.vi"("error in (no error)"=w833, "Start/Stop (False: Stop)"="Start/Stop (Wh Integration)", "VISA resource name"=w826) -> ("error out"=w835:errorcluster)  [unwired: 7 in, 1 out]
              }
            }
            n312 = call <vilib>:"Clear Errors.vi"("error in (no error)"=w813, "specific error code to clear (0: all)"=0) -> ("error out"=w812:errorcluster)  [unwired: 4 in, 1 out]
          }
        }
      }
      frame "---------- Core ----------" {
        n313 = call <vilib>:"Add State(s) to Queue__jki_lib_state_machine.vi"("State(s) in (\"\")"=w840) -> ("States Out"=w839:string)  [unwired: 14 in]
      }
      frame Default {
        w850 = 42 items=["No error", "Argument error", "Memory is full", "Out of zone", "End of file", "File already open", "Generic file I/O error", "File not found", "File permission error", "Disk is full", "Duplicate path", "Too many files open", "System feature not enabled", "Resource file not found", "Cannot add resource", "Resource not found", "Image not found", "Image memory error", "Pen does not exist", "Config type invalid", "Config token not found", "Config parse error", "Config memory error", "Bad external code format", "Bad external code offset", "External code not present", "Null window", "Destroy window error", "Null menu", "Print aborted", "Bad print record", "Print driver error", "Windows error during printing", "Memory error during printing", "Print dialog error", "Generic print error", "Invalid device refnum", "Device not found", "Device parameter error", "Device unit error", "Cannot open device", "Device call aborted", "Generic error", "Cancelled by user", "Object ID too low", "Object ID too high", "Object not in heap", "Unknown heap", "Unknown object (invalid DefProc)", "Unknown object (DefProc not in table)", "Message out of range", "Invalid (null) method", "Unknown message", "Manager call not supported", "Bad address", "Network operation in progress", "Network operation timed out", "Connection is busy", "Network attribute not supported", "Network error", "Address in use", "System out of memory", "Connection aborted", "Connection refused", "Not connected", "Already connected", "Connection closed", "Initialization error (interapplication manager)", "Bad occurrence", "Wait on unbound occurrence handler", "Occurrence queue overflow", "Datalog type conflict", "Unused", "Unrecognized type (interapplication manager)", "Memory corrupt", "Failed to make temporary DLL", "Old CIN version", "Drag socket not found", "Failed to load drop-object", "Failed to register OLE object", "Failed to release OLE object", "Format specifier type mismatch", "Unknown format specifier", "Too few format specifiers", "Too many format specifiers", "Scan failed", "Newer CIN version", "Error converting to variant", "Runtime menu error", "Password tampered", "Variant attribute not found", "Incompatible variant data type", "Event data is not available", "Event Store is not present", "Occurrence is not found", "Event Queue is not created", "Event info is not available", "Refnum passed is NULL", "Error retrieving Class GUID", "Error retrieving CoClass GUID", "Error retrieving TypeLib GUID.", "Bad built application magic bytes.", "Specific driver is different from the specific driver associated with the Logical Name.", "There is no session opened to the class driver.", "Max Error", "MAX - Error with config objects", "MAX - Error loading configuration", "MAX - Group not supported"]
        # "Current State"
        # "Handle mistyped state name (developer tool)"
        n314 = Format Into String(format string="Software Exception: Unhandled State \"%s\"." ("message"), error in=w846, w842) -> (resulting string=w849:string, error out=w848:errorcluster)  [unwired: 1 in]
        n315 = call <vilib>:"Error Cluster From Error Code.vi"("show call chain? (False)"=TRUE, "error in (no error)"=w848, "error message (\"\")"=w849, "error code (0)"=w850) -> ("error out"=w847:errorcluster)  [unwired: 5 in]
        n316 = call <vilib>:"Add State(s) to Queue__jki_lib_state_machine.vi"("State(s) in (\"\")"=w845) -> ("States Out"=w844:string)  [unwired: 14 in]
      }
      frame "Initialize Core Data" {
        # "originally closed?"
        # "exe?"
        # "If panel starts closed or is an EXE, then close it when we exit"
        n317 = property class="App"() -> ("App.Kind"=w858:T56)  [unwired: 2 in, 2 out]
        n318 = control-ref of="Current VI Reference"() -> (w852:refnum<vi>)
        n319 = property class="VI"() -> ("Front Panel.Open"=w859:bool)  [unwired: 2 in, 2 out]
        n320 = Not(x=w859) -> (.not. x?=w856:bool)
        n321 = Equal?(x=w858, y=T56."Run Time System" ("Application:Kind")) -> (x = y?=w855:bool)
        n322 = Or(x=w856, y=w855) -> (x .or. y?=w853:bool)
        n323 = Bundle By Name(cluster=w854, "Core.Current VI Reference"=w852, "Core.Close Panel on Exit?"=w853) -> (w861:T62)
        n324 = call <vilib>:"Add State(s) to Queue__jki_lib_state_machine.vi"("State(s) in (\"\")"=w863) -> ("States Out"=w862:string)  [unwired: 14 in]
      }
      frame "Error Handler" {
        n325 = call <vilib>:"General Error Handler.vi"("error in (no error)"=w866) -> ()  [unwired: 10 in, 5 out]
        n326 = call <vilib>:"Add State(s) to Queue__jki_lib_state_machine.vi"("State(s) in Front (\"\")"="/* Post Error States", "State(s) in (\"\")"=w870) -> ("States Out"=w869:string)  [unwired: 13 in]
      }
      frame "Exit" {
        w871 = TRUE
        n327 = call <vilib>:"Add State(s) to Queue__jki_lib_state_machine.vi"("State(s) in (\"\")"=w875) -> ("States Out"=w874:string)  [unwired: 14 in]
        "Main Exit" <- w871
      }
      frame "---------- Data ----------" {
        n328 = call <vilib>:"Add State(s) to Queue__jki_lib_state_machine.vi"("State(s) in (\"\")"=w879) -> ("States Out"=w878:string)  [unwired: 14 in]
      }
      frame "Data: Initialize" {
        n329 = flat-sequence {
          tunnel: [w899] -> w885
          tunnel: w882 -> [w898]
          tunnel: [w898] -> w881
          frame #0 {
            w892 = FALSE  # Force Read Point
            w893 = FALSE  # Wait for Power Threshold (Output)
            w894 = string[][] []  # Full Data Output
            w895 = FALSE  # Reset Timer
            w897 = FALSE  # New File
            w900 = dbl[][] []  # Plot Array
            w901 = string[][] []  # Save Data
            w906 = T60 {"IGBT Temp (Deg C)"=0, "Speed"=0, "Load Size"=0, "Temperature"=0, "Water Pressure"=0, "Detergent"=0, "Fabric Softener"=0, "Direction"="", "Det"=FALSE, "FS"=FALSE, "Recirc"=FALSE, "Drain"=FALSE, "Hot"=FALSE, "Cold"=FALSE, "LidClosed"=FALSE, "LidLocked"=FALSE, "Motor Speed"=0, "Latched Out Of Balance"=0, "Raw Out Of Balance"=0, "Plaster Status"=0, "Inverter Power (Watts)"=0, "Profiler Status"="", "Profiler CRC"=0, "Current Inverter Action"="", "Target Speed (BRPM)"=0, "Latched Agitate Motor Temp (Deg C)"=0, "Current Motor Temp (Deg C)"=0, "Error Codes 1"=""}  # Laundry GEA2 Data
            w904 = T61 {"Model Information"=[], "Program Names"=[], "Search Program Name"="", "Parsed Program List"=[], "Header"=[], "Search Model Name"="", "File Search Parameters"=[], "Test Date"=timestamp(0 s since 1904-01-01), "AF/MF Unit Number"="", "Stby Pwr Unit"="", "Model Details Header"=[], "Model Details Output"=[], "End of Cycle Commands"=[], "Raw Data"=[], "Startup Config Data"=[]}  # Configuration File Param
            w907 = string[][] []  # Calibration
            w909 = string[][] []  # Total Array
            n330 = Bundle("Core"=T57 {"Current VI Reference"=refnum, "Close Panel on Exit?"=FALSE}, "Total Array"=w909, "Measurments"="Measurments", "Calibration"=w907, "Filepath"="Filepath", "Laundry GEA2 Data"=w906, "Configuration File Param"=w904, "Excel Report"=refnum<class "NI_report.lvclass"> refnum, "Washer Controls Input"="Washer Controls Input", "Power Analyzer"="Power Analyzer", "Save Data"=w901, "Plot Array"=w900, "New File"=w897, "Reset Timer"=w895, "Full Data Output"=w894, "Wait for Power Threshold (Output)"=w893, "Force Read Point"=w892) -> (w899:T62)  [unwired: 1 in]
          }
        }
        n331 = call <vilib>:"Add State(s) to Queue__jki_lib_state_machine.vi"("State(s) in (\"\")"=w891) -> ("States Out"=w890:string)  [unwired: 14 in]
        n332 = Current VI's Path() -> (path=w889:path)
        n333 = call "UTILITY This VIs Path.vi"("path"=w889, "error in (no error)"=w881) -> ("Folder Path"=w883:path, "FileVersionInfo Out"=w888:T19, "error out"=w886:errorcluster)  [unwired: 7 in, 4 out]
        "Folder Path" <- w883
        n334 = Unbundle By Name(w888) -> ("FileVersion"=→"File  Version":string)
        n335 = Bundle By Name(cluster=w885, "Filepath.General Setup Paths.Tool Base Path"=w883) -> (w884:T62)
        n336 = local write "Main Tab"(T1."Main" ("Main Tab")) -> ()
      }
      frame "Get File Info" {
        # "I removed Capacity measurments"
        # "If you are logging data, enable the auto terminate\nbutton"
        # "Setup the file and location"
        n337 = local read "Front Program Name"() -> (w916:string)
        n338 = Unbundle By Name(w919) -> ("Filepath"=w918:T38, "Washer Controls Input"=w915:T8)
        n339 = call "DOE Search Program Name.vi"("Program Name"=w916) -> ("LV Program"=w911:T49)  [unwired: 10 in]
        n340 = call "Save File DOE File Setup.vi"("Filepath In"=w918, "Washer Controls In"=w915, "error in (no error)"=w924, "Config State"="Config State", "LV Program"=w911) -> ("Washer Controls Out"=w913:T8, "Filepath Out"=w922:T38, "error out"=w914:errorcluster)  [unwired: 12 in]
        "Washer Controls" <- w913
        n341 = Unbundle By Name(w913) -> ("Initialize.Washer In"=w912:T17)
        n342 = local write "Filepath"(w922) -> ()
        n343 = Bundle By Name(cluster=w919, "Washer Controls Input.Initialize.Washer In"=w912, "Filepath"=w922) -> (w921:T62)
        n344 = call <vilib>:"Add State(s) to Queue__jki_lib_state_machine.vi"("State(s) in (\"\")"=w925) -> ("States Out"=w926:string)  [unwired: 14 in]
        n345 = flat-sequence {
          tunnel: w914 -> [w929]
          tunnel: [w929] -> w923
          frame #0 {
            w927 = TRUE ("Start Saving Data")
            n346 = property on="Auto-Terminate Prog" class="Bool (strict)"("DisabledEnum"=T45."Enabled" ("Disabled")) -> ()  [unwired: 2 in, 2 out]
            n347 = local write "Start Saving Data"(w927) -> ()
            n348 = local write "Wait for Power Threshold"(w927) -> ()
          }
        }
        n349 = Unbundle By Name(w921) -> ("Washer Controls Input.Initialize.Washer In.Appliance Details.File Name Output Array"=→"File Name Output Array":string[][])
      }
      frame "Load Config File" {
        # "Load the config file"
        n350 = Unbundle By Name(w936) -> ("Filepath"=w932:T38, "Washer Controls Input"=w934:T8)
        n351 = local read "Front Program Name"() -> (w938:string)
        n352 = case shown="\"Portable\"" w938 {
          tunnel: [Save_File_DOE_LabView_Program."DOE Stand" ("LV Program") Save_File_DOE_LabView_Program."Dishwasher Kitchen" ("LV Program") Save_File_DOE_LabView_Program."Portable Stand" ("LV Program")] -> w933
          frame "DOE Stand", Default {
          }
          frame "Kitchen" {
          }
          frame "Portable" {
          }
        }
        n353 = call "Save File DOE File Setup.vi"("Filepath In"=w932, "Washer Controls In"=w934, "error in (no error)"=w941, "Config State"=Save_File_DOE_Configuration_State."Load Config", "LV Program"=w933) -> ("Washer Controls Out"=w931:T8, "Filepath Out"=w940:T38, "error out"=w939:errorcluster)  [unwired: 12 in]
        n354 = Unbundle By Name(w931) -> ("Test Fixture Hardware"=w930:T9)
        n355 = local write "Washer Controls"(w931) -> ()
        n356 = call <vilib>:"Add State(s) to Queue__jki_lib_state_machine.vi"("State(s) in (\"\")"=w942) -> ("States Out"=w943:string)  [unwired: 14 in]
        n357 = Bundle By Name(cluster=w936, "Washer Controls Input.Test Fixture Hardware"=w930, "Filepath"=w940) -> (w935:T62)
        n358 = local write "Filepath"(w940) -> ()
      }
      frame "Populate XY Axis" {
        n359 = Unbundle By Name(w950) -> ("Save Data"=w948:string[][])
        n360 = Index Array(array=w948, index (row)=0 ("disabled index (col)")) -> (element=w952:string[])  [unwired: 1 in]
        n361 = Index Array(array=w948, index (row)=0 ("disabled index (col)")) -> (element=w954:string[])  [unwired: 1 in]
        n362 = Index Array(array=w948, index (row)=0 ("disabled index (col)")) -> (element=w947:string[])  [unwired: 1 in]
        n363 = property on="X-Axis" class="CmbBox"("Strings[]"=w952) -> ()  [unwired: 2 in, 2 out]
        n364 = property on="Y-Axis-1" class="CmbBox"("Strings[]"=w954) -> ()  [unwired: 2 in, 2 out]
        n365 = property on="Y-Axis-2" class="CmbBox"("Strings[]"=w947) -> ()  [unwired: 2 in, 2 out]
        n366 = call <vilib>:"Add State(s) to Queue__jki_lib_state_machine.vi"("State(s) in (\"\")"=w956) -> ("States Out"=w957:string)  [unwired: 14 in]
      }
      frame "---- Initialization ----" {
        n367 = call <vilib>:"Add State(s) to Queue__jki_lib_state_machine.vi"("State(s) in (\"\")"=w961) -> ("States Out"=w960:string)  [unwired: 14 in]
      }
      frame "Init 34972" {
        n368 = Unbundle By Name(w965) -> ("Washer Controls Input.Test Fixture Hardware.Analog Data.Select Analog"=w964:string)
        n369 = case shown="\"\", Default" w964 {
          tunnel: w966 -> [w974 w976]
          tunnel: [w973 w976] -> w962
          tunnel: w965 -> [w972 w975]
          tunnel: [w970 w975] -> w963
          frame "34970A_DISH_DOE_1", "34970A_DISH_DOE_2", "34970A_DISH_DOE_3", "34972A_1", "34972A_2", "34972A_3", "34972A_4", "34972A_5", "34972A_6", "AGILENT", "AGILENT_HCC" {
            n370 = Unbundle By Name(w972) -> ("Washer Controls Input.Test Fixture Hardware"=w969:T9)
            n371 = call "DOE Agilent Setup.vi"("error in (no error)"=w974, "Test Fixture Hardware"=w969) -> ("error out"=w973:errorcluster, "Test Fixture Hardware Output"=w971:T9)  [unwired: 8 in]
            n372 = Bundle By Name(cluster=w972, "Washer Controls Input.Test Fixture Hardware"=w971) -> (w970:T62)
          }
          frame "", Default {
          }
        }
        n373 = call <vilib>:"Add State(s) to Queue__jki_lib_state_machine.vi"("State(s) in (\"\")"=w967) -> ("States Out"=w968:string)  [unwired: 14 in]
      }
      frame "Init Time" {
        n374 = call "UTILITY E-Time.vi"("Reset"=TRUE) -> ("Elapsed Time (sec)"=→"Start Time (sec)":dbl)  [unwired: 8 in, 2 out]
        n375 = call <vilib>:"Add State(s) to Queue__jki_lib_state_machine.vi"("State(s) in (\"\")"=w982) -> ("States Out"=w981:string)  [unwired: 14 in]
      }
      frame "Equipment" {
        n376 = Unbundle By Name(w985) -> ("Washer Controls Input.Test Fixture Hardware.Power.Yokogawa"=w991:T63, "Washer Controls Input.Test Fixture Hardware.Power.Aplus"=w990:T64, "Power Analyzer"=w993:T37, "Washer Controls Input.Test Fixture Hardware.Power.Yokogawa.WT500.V Range (8: 1000V)"=w988:i32, "Washer Controls Input.Test Fixture Hardware.Power.Yokogawa.WT500.I Range (7: 40A)"=w987:i32, "Washer Controls Input.Test Fixture Hardware.Power.Yokogawa.WT500.Update Rate (3: 500ms)"=w986:i32)
        n377 = case shown="\"APLUS\"" w993 {
          tunnel: w992 -> [w996 w1008 w1013 w1021 w1032 w1042 w1052 w1065 w1068 w1070]
          tunnel: [w996 w1007 w1012 w1020 w1031 w1041 w1051 w1058 w1068 w1070] -> w989
          tunnel: w991 -> [_ _ w1011 w1019 w1034 w1044 w1054 w1066 _ _]
          tunnel: w990 -> [_ w1002 _ _ _ _ _ _ _ _]
          tunnel: w988 -> [_ _ _ _ _ _ _ w1064 _ _]
          tunnel: w987 -> [_ _ _ _ _ _ _ w1063 _ _]
          tunnel: w986 -> [_ _ _ _ _ _ _ w1062 _ _]
          tunnel: w985 -> [w997 w998 w1009 w1017 w1030 w1040 w1050 w1061 w1067 w1069]
          tunnel: [w997 w998 w1009 w1017 w1029 w1039 w1049 w1061 w1067 w1069] -> w984
          tunnel: "Manual Range (20 <10> A)" -> [_ _ _ _ w1025 w1035 w1045 _ _ _]
          frame "", Default {
          }
          frame "APLUS" {
            w1003 = u16 2 items=["0.1s", "0.25s", "0.5s", "1s", "2s", "5s"] ("Sample Rate (1: 0.25s)")
            w1004 = u16 12 items=["Auto", "5mA", "10mA", "20mA", "50mA", "100mA", "200mA", "0.5A", "1A", "2A", "5A", "10A", "20A", "50mV", "100mV", "200mV", "2.5V", "5V", "10V"] ("A Range (12: 20A)")
            w1005 = u16 4 items=["Auto", "15V", "30V", "60V", "150V", "300V", "600V"] ("V Range (6: 600V)")
            n378 = Unbundle By Name(w1002) -> ("Aplus IP Address"=w1001:string, "Remote Port"=w1000:i32, "Instrument"=w999:string)
            n379 = call "APLUS IEC 2015 Setup.vi"("Remote IP Address"=w1001, "Instrument"=w999, "Sample Rate (1: 0.25s)"=w1003, "Remote Port"=w1000, "V Range (6: 600V)"=w1005, "A Range (12: 20A)"=w1004, "error in"=w1008, "Reset WattHours"=TRUE) -> ("error out"=w1007:errorcluster)  [unwired: 5 in, 2 out]
          }
          frame "WT210" {
            w1014 = u16 2 items=["0.1s", "0.25s", "0.5s", "1s", "2s", "5s"] ("Sample Rate (1: 0.25s)")
            w1015 = u16 12 items=["Auto", "5mA", "10mA", "20mA", "50mA", "100mA", "200mA", "0.5A", "1A", "2A", "5A", "10A", "20A", "50mV", "100mV", "200mV", "2.5V", "5V", "10V"] ("A Range (12: 20A)")
            w1016 = u16 4 items=["Auto", "15V", "30V", "60V", "150V", "300V", "600V"] ("V Range (6: 600V)")
            # "Cannot have Auto Scale and integration on older units"
            n380 = Unbundle By Name(w1011) -> ("WT210.Power VISA Yokogawa WT210"=w1010:refnum<visa-resource-name>)
            n381 = call "WT210 IEC 2015 Setup.vi"("VISA Input"=w1010, "V Range (6: 600V)"=w1016, "A Range (12: 20A)"=w1015, "Sample Rate (1: 0.25s)"=w1014, "error in (no error)"=w1013) -> ("error out"=w1012:errorcluster)  [unwired: 7 in, 3 out]
          }
          frame "WT230" {
            w1022 = u16 2 items=["0.1s", "0.25s", "0.5s", "1s", "2s", "5s"] ("Sample Rate (1: 0.25s)")
            w1023 = u16 12 items=["Auto", "5mA", "10mA", "20mA", "50mA", "100mA", "200mA", "0.5A", "1A", "2A", "5A", "10A", "20A", "50mV", "100mV", "200mV", "2.5V", "5V", "10V"] ("A Range (12: 20A)")
            w1024 = u16 5 items=["Auto", "15V", "30V", "60V", "150V", "300V", "600V"] ("V Range (6: 600V)")
            # "Cannot have Auto Scale and integration on older units"
            n382 = Unbundle By Name(w1019) -> ("WT210.Power VISA Yokogawa WT210"=w1018:refnum<visa-resource-name>)
            n383 = call "WT210 IEC 2015 Setup.vi"("VISA Input"=w1018, "V Range (6: 600V)"=w1024, "A Range (12: 20A)"=w1023, "Sample Rate (1: 0.25s)"=w1022, "error in (no error)"=w1021) -> ("error out"=w1020:errorcluster)  [unwired: 7 in, 3 out]
          }
          frame "WT300" {
            w1027 = 0.1 items=["100m"=0.1, "250m"=0.25, "500m"=0.5, "1"=1.0, "2"=2.0, "5"=5.0] ("Update Rate (250m s)")
            n384 = Unbundle By Name(w1034) -> ("WT210.Power VISA Yokogawa WT210"=w1033:refnum<visa-resource-name>)
            n385 = call "WT300 IEC 2015 Setup.vi"("VISA Input"=w1033, "Update Rate (250m s)"=w1027, "error in (no error)"=w1032, "Enable Auto Range (F: Disable)"=FALSE, "Manual Range (20 <10> A)"=w1025) -> ("VISA Output"=w1028:refnum<visa-resource-name>, "error out"=w1031:errorcluster)  [unwired: 7 in, 2 out]
            n386 = Bundle By Name(cluster=w1030, "Washer Controls Input.Test Fixture Hardware.Power.Yokogawa.WT210.Power VISA Yokogawa WT210"=w1028) -> (w1029:T62)
          }
          frame "WT300_1" {
            w1037 = 0.1 items=["100m"=0.1, "250m"=0.25, "500m"=0.5, "1"=1.0, "2"=2.0, "5"=5.0] ("Update Rate (250m s)")
            n387 = Unbundle By Name(w1044) -> ("WT310_2.Power VISA Yokogawa WT310_2"=w1043:refnum<visa-resource-name>)
            n388 = call "WT300 IEC 2015 Setup.vi"("VISA Input"=w1043, "Update Rate (250m s)"=w1037, "error in (no error)"=w1042, "Enable Auto Range (F: Disable)"=FALSE, "Manual Range (20 <10> A)"=w1035) -> ("VISA Output"=w1038:refnum<visa-resource-name>, "error out"=w1041:errorcluster)  [unwired: 7 in, 2 out]
            n389 = Bundle By Name(cluster=w1040, "Washer Controls Input.Test Fixture Hardware.Power.Yokogawa.WT310_2.Power VISA Yokogawa WT310_2"=w1038) -> (w1039:T62)
          }
          frame "WT300_2" {
            w1047 = 0.1 items=["100m"=0.1, "250m"=0.25, "500m"=0.5, "1"=1.0, "2"=2.0, "5"=5.0] ("Update Rate (250m s)")
            n390 = Unbundle By Name(w1054) -> ("WT310_3.Power VISA Yokogawa WT310_3"=w1053:refnum<visa-resource-name>)
            n391 = call "WT300 IEC 2015 Setup.vi"("VISA Input"=w1053, "Update Rate (250m s)"=w1047, "error in (no error)"=w1052, "Enable Auto Range (F: Disable)"=FALSE, "Manual Range (20 <10> A)"=w1045) -> ("VISA Output"=w1048:refnum<visa-resource-name>, "error out"=w1051:errorcluster)  [unwired: 7 in, 2 out]
            n392 = Bundle By Name(cluster=w1050, "Washer Controls Input.Test Fixture Hardware.Power.Yokogawa.WT310_3.Power VISA Yokogawa WT310_3"=w1048) -> (w1049:T62)
          }
          frame "WT500" {
            n393 = Unbundle By Name(w1066) -> ("WT500.Power VISA Yokogawa WT500"=w1056:refnum<visa-resource-name>)
            n394 = call "WT500 IEC 2015 Setup.vi"("VISA Input"=w1056, "Wiring (0: 1P2W, 1P2W, 1P2W)"="Wiring (0: 1P2W, 1P2W, 1P2W)", "V Range (8: 1000V)"=w1064, "I Range (7: 40A)"=w1063, "Update Rate (3: 500ms)"=w1062, "Error In"=w1065, "Start/Stop (False: Stop)"=TRUE) -> ("Error Out"=w1059:errorcluster)  [unwired: 4 in, 4 out]
            n395 = call <vilib>:"Clear Errors.vi"("error in (no error)"=w1059, "specific error code to clear (0: all)"=0) -> ("error out"=w1058:errorcluster)  [unwired: 4 in, 1 out]
          }
          frame "Debug" {
            # "Debug"
          }
          frame "OSI" {
          }
        }
        n396 = call <vilib>:"Add State(s) to Queue__jki_lib_state_machine.vi"("State(s) in (\"\")"=w995) -> ("States Out"=w994:string)  [unwired: 14 in]
      }
      frame "Initialize Chroma" {
        n397 = Unbundle By Name(w1076) -> ("Washer Controls Input.Test Fixture Hardware.Power.Power Supply.Use Chroma?"=w1072:bool, "Washer Controls Input.Test Fixture Hardware.Power.Power Supply.Chroma 61605"=w1075:refnum<visa-resource-name>)
        n398 = case shown="True" w1072 {
          tunnel: w1075 -> [_ w1085]
          tunnel: w1074 -> [w1081 w1084]
          tunnel: [w1081 w1083] -> w1073
          frame False {
          }
          frame True {
            n399 = call "CHROMA Initialize.vi"("Error In"=w1084, "CHROMA VISA In"=w1085) -> ("Error Out"=w1083:errorcluster, "Instrument Name"=→"Chroma Name":string)  [unwired: 7 in, 1 out]
          }
        }
        n400 = case shown="True" w1072 {
          tunnel: [T45."Disabled and Grayed Out" ("Disabled") T45."Enabled" ("Disabled")] -> w1071
          frame False {
          }
          frame True {
          }
        }
        n401 = property on="Set Initialization" class="Bool"("DisabledEnum"=w1071) -> ()  [unwired: 2 in, 2 out]
        n402 = property on="Power Supply Status" class="Bool (strict)"("DisabledEnum"=w1071) -> ()  [unwired: 2 in, 2 out]
        n403 = property on="Set Parameters" class="Bool"("DisabledEnum"=w1071) -> ()  [unwired: 2 in, 2 out]
        n404 = property on="L1 Voltage" class="DigNum (strict)"("DisabledEnum"=w1071) -> ()  [unwired: 2 in, 2 out]
        n405 = property on="L2 Voltage" class="DigNum (strict)"("DisabledEnum"=w1071) -> ()  [unwired: 2 in, 2 out]
        n406 = property on="Frequency" class="DigNum (strict)"("DisabledEnum"=w1071) -> ()  [unwired: 2 in, 2 out]
        n407 = call <vilib>:"Add State(s) to Queue__jki_lib_state_machine.vi"("State(s) in (\"\")"=w1078) -> ("States Out"=w1077:string)  [unwired: 14 in]
      }
      frame "Initialize Barometer" {
        n408 = Unbundle By Name(w1086) -> ("Washer Controls Input.Test Fixture Hardware.Barometric Pressure.Use Barometer?"=w1088:bool, "Washer Controls Input.Test Fixture Hardware.Barometric Pressure.HEISE 901A"=w1087:refnum<visa-resource-name>)
        n409 = case shown="False" w1088 {
          tunnel: w1090 -> [w1093 w1096]
          tunnel: [w1093 w1095] -> w1089
          tunnel: w1087 -> [_ w1094]
          frame False {
          }
          frame True {
            n410 = call "Heise Barometric Pressure 901A Initialize.vi"("error in (no error)"=w1096, "VISA Refnum in"=w1094) -> ("error out"=w1095:errorcluster)  [unwired: 8 in, 1 out]
          }
        }
        n411 = call <vilib>:"Add State(s) to Queue__jki_lib_state_machine.vi"("State(s) in (\"\")"=w1092) -> ("States Out"=w1091:string)  [unwired: 14 in]
      }
      frame "Off-Standby Mode" {
        # "Pause the DAQ during Standby collection"
        n412 = Unbundle By Name(w1109) -> ("Washer Controls Input.Initialize.Washer In.Appliance Details.Appliance Common"=w1098:T20, "Washer Controls Input.Test Fixture Hardware.Power"=w1111:T10, "Power Analyzer"=w1110:T37)
        n413 = local read "Station Name (Specific)"() -> (w1102:string)
        n414 = call "Off Mode Standby Mode Power Measure SM.vi"("Power"=w1111, "Station Label"=w1102, "Appliance Common"=w1098, "Power Analyzer"=w1110, "Error In"=w1101) -> ("Standby Power Out"=w1097:T28, "Error Out"=w1100:errorcluster)  [unwired: 9 in]
        "Measurments.Standby Power" <- w1097
        n415 = Unbundle By Name(w1097) -> ("Standby Power Spreadsheet"=w1099:string[][])
        "Standby Power Data" <- w1099
        n416 = call <vilib>:"Add State(s) to Queue__jki_lib_state_machine.vi"("State(s) in (\"\")"=w1113) -> ("States Out"=w1112:string)  [unwired: 14 in]
        n417 = Index Array(array=w1099, index (col)=0 ("disabled index (col)")) -> (element=w1106:string[])  [unwired: 1 in]
        n418 = Search 1D Array(1D array=w1106, element="System Date" ("regular expression")) -> (index of element=w1104:i32)  [unwired: 1 in]
        n419 = Index Array(array=w1099, index (row)=w1104) -> (element=w1103:string[])  [unwired: 1 in]
        n420 = property on="X-Axis (Standby)" class="CmbBox"("Strings[]"=w1103) -> ()  [unwired: 2 in, 2 out]
        n421 = property on="Y-Axis (Standby)" class="CmbBox"("Strings[]"=w1103) -> ()  [unwired: 2 in, 2 out]
        n422 = Bundle By Name(cluster=w1109, "Measurments.Standby Power"=w1097) -> (w1108:T62)
      }
      frame "Data: Cleanup" {
        n423 = Unbundle By Name(w1114) -> ("Core.Current VI Reference"=w1117:refnum<vi>)
        n424 = Close Reference(reference=w1117, error in (no error)=w1116) -> (error out=w1115:errorcluster)
        n425 = call <vilib>:"Add State(s) to Queue__jki_lib_state_machine.vi"("State(s) in (\"\")"=w1119) -> ("States Out"=w1118:string)  [unwired: 14 in]
      }
      frame "---------- UI ----------" {
        n426 = call <vilib>:"Add State(s) to Queue__jki_lib_state_machine.vi"("State(s) in (\"\")"=w1123) -> ("States Out"=w1122:string)  [unwired: 14 in]
      }
      frame "UI: Initialize" {
        # "This prevents sending a \nblank file path to the Sys Exe\nVI below (ERD)"
        n427 = Unbundle By Name(w1134) -> ("Filepath.General Setup Paths.Tool Base Path"=w1142:path)
        n428 = call "UTILITY Initialize Front Panel Controls.vi"("Initial DOE Config"=w1142) -> ("Initial DOE Config 2"=w1132:path, "Front Panel Controls DOE"=w1159:T65)  [unwired: 9 in]
        "Config Path with Tool Base" <- w1132
        n429 = Unbundle By Name(w1159) -> ("TC Type (K,J)"=w1140:string, "Station Name (Specific)"=→"Station Name (Specific)":string, "Agilent Gain"=w1139:dbl, "Scale"=w1146:string, "Flow Rates"=w1144:string, "Analog DAQ"=w1143:string, "Laurel Communication Type"=w1145:string, "Enable Dryer PreCondition"=w1125:bool, "Dishwasher Events Visible"=w1153:bool, "Standby Power Enabled"=w1128:bool, "Reset Power Meter Enabled"=w1129:bool, "Rinse Button Enabled"=w1152:bool, "Final RMC Enabled"=w1150:bool, "Reset Cold Laurel Meter Enabled"=w1148:bool, "Reset Hot Laurel Meter Enabled"=w1137:bool, "Test Stand Name (General)"=→"Front Program Name":string, "Power Analyzer"=w1161:string, "Scan Rate (Sec)"=w1160:dbl, "Auto Terminate Power Limit (Watts)"=w1158:dbl, "Time Limit At Power Level (Seconds)"=w1157:dbl, "Hot Water Estimated Water Usage (Gallons)"=w1156:dbl, "Cold Water Estimated Water Usage (Gallons)"=w1155:dbl, "Max File Size"=→"Max File Size":dbl, "Use Chroma?"=w1135:bool, "Use Heise Barometric Pressure"=w1127:bool, "Cycles Per Year"=w1124:u32)
        "Dishwasher Events Visible" <- w1153
        n430 = Bundle By Name(cluster=w1134, "Filepath.General Setup Paths.General Startup Config Path"=w1132) -> (w1133:T62)
        n431 = case shown="True" w1125 {
          tunnel: [T45."Disabled and Grayed Out" ("Disabled") T45."Enabled" ("Disabled")] -> w1126
          frame False {
          }
          frame True {
          }
        }
        n432 = case shown="True" w1128 {
          tunnel: [T45."Disabled and Grayed Out" ("Disabled") T45."Enabled" ("Disabled")] -> w1131
          frame False {
          }
          frame True {
          }
        }
        n433 = case shown="True" w1129 {
          tunnel: [T45."Disabled and Grayed Out" ("Disabled") T45."Enabled" ("Disabled")] -> w1130
          frame False {
          }
          frame True {
          }
        }
        n434 = case shown="True" w1152 {
          tunnel: [T45."Disabled and Grayed Out" ("Disabled") T45."Enabled" ("Disabled")] -> w1151
          frame False {
          }
          frame True {
          }
        }
        n435 = case shown="True" w1150 {
          tunnel: [T45."Disabled and Grayed Out" ("Disabled") T45."Enabled" ("Disabled")] -> w1149
          frame False {
          }
          frame True {
          }
        }
        n436 = case shown="True" w1148 {
          tunnel: [T45."Disabled and Grayed Out" ("Disabled") T45."Enabled" ("Disabled")] -> w1147
          frame False {
          }
          frame True {
          }
        }
        n437 = case shown="True" w1137 {
          tunnel: [T45."Disabled and Grayed Out" ("Disabled") T45."Enabled" ("Disabled")] -> w1136
          frame False {
          }
          frame True {
          }
        }
        n438 = local write "Enable RMC Collection"(w1125) -> ()
        n439 = local write "Cold Estimated Water Usage (Gallons)"(w1155) -> ()
        n440 = local write "Hot Estimated Water Usage (Gallons)"(w1156) -> ()
        n441 = local write "Time Limit At Power Limit (Seconds)"(w1157) -> ()
        n442 = local write "Scan Rate (Seconds)"(w1160) -> ()
        n443 = local write "Power Limit (Watts)"(w1158) -> ()
        n444 = property on="Rinse Button?" class="Bool (strict)"("DisabledEnum"=w1151) -> ()  [unwired: 2 in, 2 out]
        n445 = property on="Final Weight" class="Bool"("DisabledEnum"=w1149) -> ()  [unwired: 2 in, 2 out]
        n446 = property on="Reset Cold Laurel Meter" class="Bool"("DisabledEnum"=w1147) -> ()  [unwired: 2 in, 2 out]
        n447 = property on="Reset Hot Laurel Meter" class="Bool"("DisabledEnum"=w1136) -> ()  [unwired: 2 in, 2 out]
        n448 = property on="Dryer Pre-Condition" class="Bool"("DisabledEnum"=w1126) -> ()  [unwired: 2 in, 2 out]
        n449 = property on="Start Standby Power" class="Bool"("DisabledEnum"=w1131) -> ()  [unwired: 2 in, 2 out]
        n450 = property on="Reset Power Meter" class="Bool"("DisabledEnum"=w1130) -> ()  [unwired: 2 in, 2 out]
        n451 = call <vilib>:"Add State(s) to Queue__jki_lib_state_machine.vi"("State(s) in (\"\")"=w1168) -> ("States Out"=w1167:string)  [unwired: 14 in]
        n452 = case shown="\"WT300\"" w1161 {
          tunnel: [UTILITY_Power_Analyzer."" ("Power Analyzer") UTILITY_Power_Analyzer."APLUS" ("Power Analyzer") UTILITY_Power_Analyzer."WT210" ("Power Analyzer") UTILITY_Power_Analyzer."WT500" ("Power Analyzer") UTILITY_Power_Analyzer."WT300" ("Power Analyzer") UTILITY_Power_Analyzer."OSI" ("Power Analyzer") UTILITY_Power_Analyzer."WT230" ("Power Analyzer") UTILITY_Power_Analyzer."WT300_1" ("Power Analyzer") UTILITY_Power_Analyzer."WT300_2" ("Power Analyzer")] -> w1165
          tunnel: w1164 -> [w1185 w1187 w1189 w1191 w1193 w1195 w1197 w1199 w1201]
          tunnel: [w1185 w1187 w1189 w1191 w1193 w1195 w1197 w1199 w1201] -> w1163
          frame Default {
          }
          frame "APLUS" {
          }
          frame "WT210" {
          }
          frame "WT500" {
          }
          frame "WT300" {
          }
          frame "OSI" {
          }
          frame "WT230" {
          }
          frame "WT310_1" {
          }
          frame "WT310_2" {
          }
        }
        n453 = property on="Dishwasher Events" class="Clust (strict)"("Visible"=w1153) -> ()  [unwired: 2 in, 2 out]
        n454 = property on="Meters To Collect (Hot Cold)" class="Str"("Value"=w1144) -> ()  [unwired: 2 in, 2 out]
        n455 = property on="Select Analog" class="Str"("Value"=w1143) -> ()  [unwired: 2 in, 2 out]
        n456 = property on="Laurel Communication Type" class="Str"("Value"=w1145) -> ()  [unwired: 2 in, 2 out]
        n457 = local write "Power Analyzer"(w1165) -> ()
        n458 = flat-sequence {
          tunnel: w1163 -> [w1184]
          tunnel: [w1184] -> w1162
          frame #0 {
            "Start DAQ" <- TRUE ("Start ERD")
          }
        }
        n459 = Bundle By Name(cluster=w1133, "Washer Controls Input.Test Fixture Hardware.Analog Data.Agilent.TC Type (K,J,T)"=w1140, "Washer Controls Input.Test Fixture Hardware.Analog Data.Agilent.Agilent Gain"=w1139, "Washer Controls Input.Test Fixture Hardware.Weight Scale.Select Scale"=w1146, "Washer Controls Input.Test Fixture Hardware.Flow Rates.Meters To Collect (Hot Cold)"=w1144, "Washer Controls Input.Test Fixture Hardware.Analog Data.Select Analog"=w1143, "Washer Controls Input.Test Fixture Hardware.Flow Rates.Laurel Communication Type"=w1145, "Power Analyzer"=w1165, "Washer Controls Input.Test Fixture Hardware.Power.Power Supply.Use Chroma?"=w1135, "Washer Controls Input.Test Fixture Hardware.Barometric Pressure.Use Barometer?"=w1127, "Washer Controls Input.Initialize.Washer In.Appliance Details.Appliance Common.Cycles Per Year"=w1124) -> (w1166:T62)
        n460 = property on="Agilent Gain" class="DigNum (strict)"("Value"=w1139) -> ()  [unwired: 2 in, 2 out]
      }
      frame "UI: Cursor Set" {
        n461 = case shown="\"Idle\", Default" w1203 {
          tunnel: w1205 -> [w1210 w1212]
          tunnel: [w1209 w1211] -> w1204
          frame "Idle", Default {
            n462 = call <vilib>:"Unset Busy.vi"("error in (no error)"=w1210) -> ("error out"=w1209:errorcluster)  [unwired: 10 in]
          }
          frame "Busy" {
            n463 = call <vilib>:"Set Busy.vi"("error in (no error)"=w1212) -> ("error out"=w1211:errorcluster)  [unwired: 9 in, 1 out]
          }
        }
        n464 = call <vilib>:"Add State(s) to Queue__jki_lib_state_machine.vi"("State(s) in (\"\")"=w1208) -> ("States Out"=w1207:string)  [unwired: 14 in]
      }
      frame "UI: Front Panel State" {
        n465 = Unbundle By Name(w1215) -> ("Core.Current VI Reference"=w1214:refnum<vi>)
        n466 = case shown="\"Open\", Default" w1213 {
          tunnel: w1217 -> [w1223 w1236]
          tunnel: [w1225 w1237] -> w1216
          tunnel: w1214 -> [w1224 w1234]
          frame "Open", Default {
            n467 = property class="VI"(reference=w1224, error in=w1223) -> (reference out=w1221:refnum<vi>, error out=w1222:errorcluster, "Front Panel.Open"=w1220:bool)
            n468 = case shown="False" w1220 {
              tunnel: [w1228 w1231] -> w1225
              tunnel: w1222 -> [w1227 w1231]
              tunnel: w1221 -> [w1226 _]
              frame False {
                n469 = invoke class="VI" method="FP.Open"(reference=w1226, error in=w1227, "Activate"=TRUE, "State"=T58."Maximized") -> (error out=w1228:errorcluster)  [unwired: 1 in, 4 out]
              }
              frame True {
              }
            }
          }
          frame "Close" {
            n470 = property class="VI"(reference=w1234, error in=w1236) -> (reference out=w1233:refnum<vi>, error out=w1235:errorcluster, "Front Panel.Open"=w1232:bool)
            n471 = case shown="True" w1232 {
              tunnel: [w1238 w1241] -> w1237
              tunnel: w1235 -> [w1238 w1240]
              tunnel: w1233 -> [_ w1239]
              frame False {
              }
              frame True {
                n472 = disable-structure shown="Disabled" {
                  disable-tunnel: [w1244 _] -> w1241
                  disable-tunnel: w1240 -> [w1243 _]
                  disable-tunnel: w1239 -> [w1242 _]
                  frame Disabled {
                    n473 = invoke class="VI" method="FP.Close"(reference=w1242, error in=w1243) -> (error out=w1244:errorcluster)  [unwired: 1 in, 2 out]
                  }
                  frame Enabled {
                  }
                }
              }
            }
          }
        }
        n474 = call <vilib>:"Add State(s) to Queue__jki_lib_state_machine.vi"("State(s) in (\"\")"=w1219) -> ("States Out"=w1218:string)  [unwired: 14 in]
      }
      frame "---------- Macro ----------" {
        n475 = call <vilib>:"Add State(s) to Queue__jki_lib_state_machine.vi"("State(s) in (\"\")"=w1248) -> ("States Out"=w1247:string)  [unwired: 14 in]
      }
      frame "Macro: Initialize" {
        # "Go through once to initialize the Populate XY Axis \nroutine"
        n476 = call <vilib>:"Add State(s) to Queue__jki_lib_state_machine.vi"("State(s) in Front (\"\")"="Data: Initialize\nInitialize Core Data\nLoad Config File\nUI: Initialize\nUI: Front Panel State >> Open\nInit 34972\nEquipment\nInitialize Chroma\nInitialize Barometer\nInit Time\nUI Update\nGather Analog Data\nGather Flow Rates\nGet Power Data\nCheck Newfi\nShow Data\nPopulate XY Axis", "State(s) in (\"\")"=w1253) -> ("States Out"=w1252:string)  [unwired: 13 in]
      }
      frame "Macro: Exit" {
        n477 = Unbundle By Name(w1272) -> ("Core.Close Panel on Exit?"=w1271:bool, "Washer Controls Input.Test Fixture Hardware.Barometric Pressure.Use Barometer?"=w1254:bool, "Washer Controls Input.Test Fixture Hardware.Barometric Pressure.HEISE 901A"=w1255:refnum<visa-resource-name>, "Washer Controls Input.Test Fixture Hardware.Analog Data.Agilent"=w1260:T66, "Washer Controls Input.Test Fixture Hardware.Analog Data.Select Analog"=w1261:string, "Washer Controls Input.Test Fixture Hardware.Flow Rates.Hot Water Laurel VISA"=w1264:refnum<visa-resource-name>, "Washer Controls Input.Test Fixture Hardware.Flow Rates.Cold Water Laurel VISA"=w1265:refnum<visa-resource-name>, "Washer Controls Input.Test Fixture Hardware.Flow Rates.Laurel Communication Type"=w1262:string)
        n478 = local write "Test Status"("Shutting Down...." ("Test Status")) -> ()
        n479 = case shown="\"SERIAL\"" w1262 {
          tunnel: w1258 -> [w1308 w1313]
          tunnel: [w1308 w1311] -> w1259
          tunnel: w1265 -> [_ w1310]
          tunnel: w1264 -> [_ w1309]
          frame "TCP", Default {
          }
          frame "SERIAL" {
            n480 = VISA Close(VISA resource name=w1310, error in (no error)=w1313) -> (error out=w1312:errorcluster)
            n481 = VISA Close(VISA resource name=w1309, error in (no error)=w1312) -> (error out=w1311:errorcluster)
          }
        }
        n482 = case shown="Default" w1261 {
          tunnel: w1260 -> [_ w1283 w1287 w1291 w1295 w1299 w1303 w1307]
          tunnel: w1259 -> [w1279 w1281 w1285 w1289 w1293 w1297 w1301 w1305]
          tunnel: [w1279 w1280 w1284 w1288 w1292 w1296 w1300 w1304] -> w1257
          frame Default {
          }
          frame "AGILENT" {
            n483 = Unbundle By Name(w1283) -> ("Agilent 34972_1"=w1282:refnum<visa-resource-name>)
            n484 = VISA Close(VISA resource name=w1282, error in (no error)=w1281) -> (error out=w1280:errorcluster)
          }
          frame "34972A_1" {
            n485 = Unbundle By Name(w1287) -> ("Agilent 34972_1"=w1286:refnum<visa-resource-name>)
            n486 = VISA Close(VISA resource name=w1286, error in (no error)=w1285) -> (error out=w1284:errorcluster)
          }
          frame "34972A_2" {
            n487 = Unbundle By Name(w1291) -> ("Agilent 34972_2"=w1290:refnum<visa-resource-name>)
            n488 = VISA Close(VISA resource name=w1290, error in (no error)=w1289) -> (error out=w1288:errorcluster)
          }
          frame "34972A_3" {
            n489 = Unbundle By Name(w1295) -> ("Agilent 34972_3"=w1294:refnum<visa-resource-name>)
            n490 = VISA Close(VISA resource name=w1294, error in (no error)=w1293) -> (error out=w1292:errorcluster)
          }
          frame "34972A_4" {
            n491 = Unbundle By Name(w1299) -> ("Agilent 34972_4"=w1298:refnum<visa-resource-name>)
            n492 = VISA Close(VISA resource name=w1298, error in (no error)=w1297) -> (error out=w1296:errorcluster)
          }
          frame "34972A_5" {
            n493 = Unbundle By Name(w1303) -> ("Agilent 34972_5"=w1302:refnum<visa-resource-name>)
            n494 = VISA Close(VISA resource name=w1302, error in (no error)=w1301) -> (error out=w1300:errorcluster)
          }
          frame "34972A_6" {
            n495 = Unbundle By Name(w1307) -> ("Agilent 34972_6"=w1306:refnum<visa-resource-name>)
            n496 = VISA Close(VISA resource name=w1306, error in (no error)=w1305) -> (error out=w1304:errorcluster)
          }
        }
        n497 = Select(t="UI: Front Panel State >> Close", s=w1271, f="") -> (s? t:f=w1268:string)
        n498 = case shown="True" w1254 {
          tunnel: w1257 -> [w1275 w1278]
          tunnel: [w1275 w1277] -> w1256
          tunnel: w1255 -> [_ w1276]
          frame False {
          }
          frame True {
            n499 = call "Heise Barometric Pressure 901A Close.vi"("error in (no error)"=w1278, "VISA Refnum in"=w1276) -> ("error out"=w1277:errorcluster)  [unwired: 9 in]
          }
        }
        n500 = call <vilib>:"Add State(s) to Queue__jki_lib_state_machine.vi"("State(s) in (\"\")"=w1268, "State(s) at Back (\"\")"="Exit") -> ("States Out"=w1266:string)  [unwired: 13 in]
        n501 = call <vilib>:"Add State(s) to Queue__jki_lib_state_machine.vi"("State(s) in Front (\"\")"=w1266, "State(s) in (\"\")"=w1274) -> ("States Out"=w1273:string)  [unwired: 13 in]
      }
      frame "---------- Collection Loop ----------" {
        n502 = call <vilib>:"Add State(s) to Queue__jki_lib_state_machine.vi"("State(s) in (\"\")"=w1317) -> ("States Out"=w1316:string)  [unwired: 14 in]
      }
      frame "UI Update" {
        n503 = Unbundle By Name(w1320) -> ("Reset Timer"=w1327:bool, "Wait for Power Threshold (Output)"=w1318:bool)
        n504 = flat-sequence {
          tunnel: w1327 -> [w1334]
          tunnel: [w1334] -> w1329
          tunnel: [w1332] -> w1328
          tunnel: w1326 -> [w1333]
          tunnel: [w1333] -> w1325
          tunnel: w1318 -> [w1332]
          tunnel: w1329 -> [w1335]
          tunnel: w1328 -> [w1336]
          tunnel: w1325 -> [w1340]
          tunnel: [w1335] -> w1323
          tunnel: [w1339] -> w1322
          tunnel: [w1338] -> w1321
          tunnel: [w1349] -> w1324
          tunnel: w1323 -> [w1347]
          tunnel: w1322 -> [w1349]
          tunnel: w1321 -> [w1348]
          tunnel: w1320 -> [w1346]
          tunnel: [w1345] -> w1319
          frame #0 {
          }
          frame #1 {
            n505 = Compound Arithmetic op=OR("Reset", w1335, w1336) -> (w1341:bool)
            n506 = call "UTILITY Elapsed Time.vi"("error in (no error)"=w1340, "Reset Timer"=w1341) -> ("error out"=w1339:errorcluster, "Main Loop Rate"=→"Main Loop Rate":dbl, "Elapsed Time"=→"Elapsed Time":dbl, "Total Array"=w1338:string[][], "Main Start"=→"Main Start":dbl)  [unwired: 5 in]
          }
          frame #2 {
            n507 = case shown="False" w1347 {
              tunnel: [w1351 w1357] -> w1345
              tunnel: w1346 -> [w1352 w1356]
              tunnel: w1348 -> [w1350 w1353]
              frame False {
                n508 = Bundle By Name(cluster=w1352, "Total Array"=w1350) -> (w1351:T62)
              }
              frame True {
                n509 = Bundle By Name(cluster=w1356, "Reset Timer"=FALSE, "Plot Array"=dbl[][] [[0.0, 0.0, 0.0], [0.0, 0.0, 0.0]], "Total Array"=w1353) -> (w1357:T62)
              }
            }
          }
        }
        n510 = call <vilib>:"Add State(s) to Queue__jki_lib_state_machine.vi"("State(s) in (\"\")"=w1331) -> ("States Out"=w1330:string)  [unwired: 14 in]
      }
      frame "Get Power Data" {
        # "Look at this..not sure what it is doing :)...and i wrote it..lol"
        n511 = Unbundle By Name(w1358) -> ("Total Array"=w1363:string[][], "Washer Controls Input.Test Fixture Hardware.Power.Yokogawa.WT500.Power VISA Yokogawa WT500"=w1362:refnum<visa-resource-name>, "Washer Controls Input.Test Fixture Hardware.Power.Yokogawa.WT210.Power VISA Yokogawa WT210"=w1364:refnum<visa-resource-name>, "Washer Controls Input.Test Fixture Hardware.Power.Aplus.Aplus IP Address"=w1369:string, "Washer Controls Input.Test Fixture Hardware.Power.Aplus.Remote Port"=w1368:i32, "Power Analyzer"=w1365:T37)
        n512 = case shown="\"WT230\"" w1365 {
          tunnel: w1369 -> [_ w1396 _ _ _ _ _ _ _ _]
          tunnel: w1368 -> [_ w1395 _ _ _ _ _ _ _ _]
          tunnel: w1367 -> [w1372 w1394 w1417 w1446 w1468 w1492 w1516 w1549 w1551 w1552]
          tunnel: [w1372 w1393 w1416 w1445 w1467 w1491 w1515 w1548 w1551 w1552] -> w1366
          tunnel: w1358 -> [w1375 w1392 w1415 w1444 w1471 w1495 w1519 w1547 w1550 w1553]
          tunnel: [w1374 w1391 w1414 w1443 w1470 w1494 w1518 w1546 w1550 w1553] -> w1361
          tunnel: w1363 -> [w1373 w1390 w1413 w1442 w1469 w1493 w1517 w1527 _ _]
          tunnel: w1364 -> [_ _ w1418 w1447 _ _ _ _ _ _]
          tunnel: w1362 -> [_ _ _ _ _ _ _ w1520 _ _]
          tunnel: w1358 -> [_ _ _ _ w1449 w1473 w1497 _ _ _]
          frame "", Default {
            n513 = Bundle By Name(cluster=w1375, "Total Array"=w1373) -> (w1374:T62)
          }
          frame "APLUS" {
            n514 = call "APLUS Camille Bauer Driver.vi"("error in (no error)"=w1394, "Remote Port"=w1395, "Remote IP Address"=w1396) -> ("error out"=w1393:errorcluster, "Power Data"=w1389:T27, "APLUS Data"=w1380:string[][])  [unwired: 4 in, 2 out]
            n515 = Unbundle By Name(w1389) -> ("Voltage (V):Element 1"=w1388:dbl, "Current (A):Element 1"=w1387:dbl, "Power (W):Sigma"=w1386:dbl, "Watt Hours (Wh):Sigma"=w1385:dbl, "Frequency (Hz):Element 1"=w1384:dbl, "Apparent Power (VA):Element 1"=w1383:dbl, "Power Factor:Element 1"=w1382:dbl, "Voltage Harmonic (%):Element 1"=w1381:dbl, "Watt Hours (Wh):Sigma"=w1378:dbl, "Max Watt Hours"=w1377:dbl)
            n516 = Build Array (concatenate)(w1390, w1380) -> (w1379:string[][])
            n517 = Max & Min(x=w1378, y=w1377) -> (max(x,y)=w1376:dbl)  [unwired: 1 out]
            n518 = Bundle By Name(cluster=w1392, "Total Array"=w1379, "Measurments.Power Measurements.Voltage (V):Element 1"=w1388, "Measurments.Power Measurements.Current (A):Element 1"=w1387, "Measurments.Power Measurements.Power (W):Sigma"=w1386, "Measurments.Power Measurements.Watt Hours (Wh):Sigma"=w1385, "Measurments.Power Measurements.Frequency (Hz):Element 1"=w1384, "Measurments.Power Measurements.Apparent Power (VA):Element 1"=w1383, "Measurments.Power Measurements.Power Factor:Element 1"=w1382, "Measurments.Power Measurements.Voltage Harmonic (%):Element 1"=w1381, "Measurments.Power Measurements.Max Watt Hours"=w1376) -> (w1391:T62)
          }
          frame "WT210" {
            n519 = call "WT210 Get Data.vi"("Collect Element 3 Data"=FALSE ("Collect Element 2 Data"), "error in (no error)"=w1417, "VISA resource name"=w1418) -> ("error out"=w1416:errorcluster, "Power Data"=w1412:T27, "Yokogawa Data"=w1402:string[][])  [unwired: 3 in, 3 out]
            n520 = Build Array (concatenate)(w1413, w1402) -> (w1401:string[][])
            n521 = Unbundle By Name(w1412) -> ("Voltage (V):Element 1"=w1411:dbl, "Current (A):Element 1"=w1410:dbl, "Power (W):Sigma"=w1409:dbl, "Watt Hours (Wh):Sigma"=w1408:dbl, "Frequency (Hz):Element 1"=w1403:dbl, "Apparent Power (VA):Element 1"=w1407:dbl, "Power Factor:Element 1"=w1406:dbl, "Voltage Crest Factor:Element 1"=w1405:dbl, "Current Crest Factor:Element 1"=w1404:dbl, "Watt Hours (Wh):Sigma"=w1400:dbl, "Max Watt Hours"=w1399:dbl)
            n522 = Max & Min(x=w1400, y=w1399) -> (max(x,y)=w1398:dbl)  [unwired: 1 out]
            n523 = Bundle By Name(cluster=w1415, "Total Array"=w1401, "Measurments.Power Measurements.Voltage (V):Element 1"=w1411, "Measurments.Power Measurements.Current (A):Element 1"=w1410, "Measurments.Power Measurements.Power (W):Sigma"=w1409, "Measurments.Power Measurements.Watt Hours (Wh):Sigma"=w1408, "Measurments.Power Measurements.Frequency (Hz):Element 1"=w1403, "Measurments.Power Measurements.Apparent Power (VA):Element 1"=w1407, "Measurments.Power Measurements.Power Factor:Element 1"=w1406, "Measurments.Power Measurements.Voltage Crest Factor:Element 1"=w1405, "Measurments.Power Measurements.Current Crest Factor:Element 1"=w1404, "Measurments.Power Measurements.Max Watt Hours"=w1398) -> (w1414:T62)
          }
          frame "WT230" {
            n524 = call "WT210 Get Data.vi"("Collect Element 3 Data"=TRUE ("Collect Element 2 Data"), "error in (no error)"=w1446, "VISA resource name"=w1447) -> ("error out"=w1445:errorcluster, "Power Data"=w1441:T27, "Yokogawa Data"=w1431:string[][])  [unwired: 3 in, 3 out]
            n525 = Build Array (concatenate)(w1442, w1431) -> (w1430:string[][])
            n526 = Unbundle By Name(w1441) -> ("Voltage (V):Element 1"=w1440:dbl, "Current (A):Element 1"=w1439:dbl, "Power (W):Sigma"=w1438:dbl, "Watt Hours (Wh):Sigma"=w1437:dbl, "Frequency (Hz):Element 1"=w1432:dbl, "Apparent Power (VA):Element 1"=w1436:dbl, "Power Factor:Element 1"=w1435:dbl, "Voltage Crest Factor:Element 1"=w1434:dbl, "Current Crest Factor:Element 1"=w1433:dbl, "Watt Hours (Wh):Sigma"=w1429:dbl, "Max Watt Hours"=w1428:dbl, "Voltage (V):Element 2"=w1425:dbl, "Current (A):Element 2"=w1424:dbl, "Power Factor:Element 2"=w1423:dbl, "Apparent Power (VA):Element 2"=w1422:dbl, "Voltage Crest Factor:Element 2"=w1421:dbl, "Current Crest Factor:Element 2"=w1420:dbl, "Voltage Harmonic (%):Element 2"=w1419:dbl)
            n527 = Max & Min(x=w1429, y=w1428) -> (max(x,y)=w1427:dbl)  [unwired: 1 out]
            n528 = Bundle By Name(cluster=w1444, "Total Array"=w1430, "Measurments.Power Measurements.Voltage (V):Element 1"=w1440, "Measurments.Power Measurements.Current (A):Element 1"=w1439, "Measurments.Power Measurements.Power (W):Sigma"=w1438, "Measurments.Power Measurements.Watt Hours (Wh):Sigma"=w1437, "Measurments.Power Measurements.Frequency (Hz):Element 1"=w1432, "Measurments.Power Measurements.Apparent Power (VA):Element 1"=w1436, "Measurments.Power Measurements.Power Factor:Element 1"=w1435, "Measurments.Power Measurements.Voltage Crest Factor:Element 1"=w1434, "Measurments.Power Measurements.Current Crest Factor:Element 1"=w1433, "Measurments.Power Measurements.Max Watt Hours"=w1427, "Measurments.Power Measurements.Voltage (V):Element 2"=w1425, "Measurments.Power Measurements.Current (A):Element 2"=w1424, "Measurments.Power Measurements.Power Factor:Element 2"=w1423, "Measurments.Power Measurements.Apparent Power (VA):Element 2"=w1422, "Measurments.Power Measurements.Voltage Crest Factor:Element 2"=w1421, "Measurments.Power Measurements.Current Crest Factor:Element 2"=w1420, "Measurments.Power Measurements.Voltage Harmonic (%):Element 2"=w1419) -> (w1443:T62)
          }
          frame "WT300" {
            n529 = Unbundle By Name(w1449) -> ("Washer Controls Input.Test Fixture Hardware.Power.Yokogawa.WT210.Power VISA Yokogawa WT210"=w1448:refnum<visa-resource-name>)
            n530 = call "WT300 Get Data.vi"("error in (no error)"=w1468, "VISA resource name"=w1448) -> ("error out"=w1467:errorcluster, "Power Data"=w1466:T27, "Yokogawa Data"=w1453:string[][])  [unwired: 4 in, 3 out]
            n531 = Unbundle By Name(w1466) -> ("Voltage (V):Element 1"=w1465:dbl, "Current (A):Element 1"=w1464:dbl, "Power (W):Sigma"=w1463:dbl, "Watt Hours (Wh):Sigma"=w1462:dbl, "Frequency (Hz):Element 1"=w1461:dbl, "Apparent Power (VA):Element 1"=w1460:dbl, "Power Factor:Element 1"=w1459:dbl, "Voltage Crest Factor:Element 1"=w1458:dbl, "Current Crest Factor:Element 1"=w1456:dbl, "Voltage Harmonic (%):Element 1"=w1457:dbl, "Time:Element 1"=w1455:dbl, "Watt Hours (Wh):Sigma"=w1452:dbl, "Max Watt Hours"=w1451:dbl)
            n532 = Build Array (concatenate)(w1469, w1453) -> (w1454:string[][])
            n533 = Max & Min(x=w1452, y=w1451) -> (max(x,y)=w1450:dbl)  [unwired: 1 out]
            n534 = Bundle By Name(cluster=w1471, "Total Array"=w1454, "Measurments.Power Measurements.Voltage (V):Element 1"=w1465, "Measurments.Power Measurements.Current (A):Element 1"=w1464, "Measurments.Power Measurements.Power (W):Sigma"=w1463, "Measurments.Power Measurements.Watt Hours (Wh):Sigma"=w1462, "Measurments.Power Measurements.Frequency (Hz):Element 1"=w1461, "Measurments.Power Measurements.Apparent Power (VA):Element 1"=w1460, "Measurments.Power Measurements.Power Factor:Element 1"=w1459, "Measurments.Power Measurements.Voltage Crest Factor:Element 1"=w1458, "Measurments.Power Measurements.Current Crest Factor:Element 1"=w1456, "Measurments.Power Measurements.Voltage Harmonic (%):Element 1"=w1457, "Measurments.Power Measurements.Time:Element 1"=w1455, "Measurments.Power Measurements.Max Watt Hours"=w1450) -> (w1470:T62)
          }
          frame "WT300_1" {
            n535 = Unbundle By Name(w1473) -> ("Washer Controls Input.Test Fixture Hardware.Power.Yokogawa.WT310_2.Power VISA Yokogawa WT310_2"=w1472:refnum<visa-resource-name>)
            n536 = call "WT300 Get Data.vi"("error in (no error)"=w1492, "VISA resource name"=w1472) -> ("error out"=w1491:errorcluster, "Power Data"=w1490:T27, "Yokogawa Data"=w1477:string[][])  [unwired: 4 in, 3 out]
            n537 = Unbundle By Name(w1490) -> ("Voltage (V):Element 1"=w1489:dbl, "Current (A):Element 1"=w1488:dbl, "Power (W):Sigma"=w1487:dbl, "Watt Hours (Wh):Sigma"=w1486:dbl, "Frequency (Hz):Element 1"=w1485:dbl, "Apparent Power (VA):Element 1"=w1484:dbl, "Power Factor:Element 1"=w1483:dbl, "Voltage Crest Factor:Element 1"=w1482:dbl, "Current Crest Factor:Element 1"=w1480:dbl, "Voltage Harmonic (%):Element 1"=w1481:dbl, "Time:Element 1"=w1479:dbl, "Watt Hours (Wh):Sigma"=w1476:dbl, "Max Watt Hours"=w1475:dbl)
            n538 = Build Array (concatenate)(w1493, w1477) -> (w1478:string[][])
            n539 = Max & Min(x=w1476, y=w1475) -> (max(x,y)=w1474:dbl)  [unwired: 1 out]
            n540 = Bundle By Name(cluster=w1495, "Total Array"=w1478, "Measurments.Power Measurements.Voltage (V):Element 1"=w1489, "Measurments.Power Measurements.Current (A):Element 1"=w1488, "Measurments.Power Measurements.Power (W):Sigma"=w1487, "Measurments.Power Measurements.Watt Hours (Wh):Sigma"=w1486, "Measurments.Power Measurements.Frequency (Hz):Element 1"=w1485, "Measurments.Power Measurements.Apparent Power (VA):Element 1"=w1484, "Measurments.Power Measurements.Power Factor:Element 1"=w1483, "Measurments.Power Measurements.Voltage Crest Factor:Element 1"=w1482, "Measurments.Power Measurements.Current Crest Factor:Element 1"=w1480, "Measurments.Power Measurements.Voltage Harmonic (%):Element 1"=w1481, "Measurments.Power Measurements.Time:Element 1"=w1479, "Measurments.Power Measurements.Max Watt Hours"=w1474) -> (w1494:T62)
          }
          frame "WT300_2" {
            n541 = Unbundle By Name(w1497) -> ("Washer Controls Input.Test Fixture Hardware.Power.Yokogawa.WT310_3.Power VISA Yokogawa WT310_3"=w1496:refnum<visa-resource-name>)
            n542 = call "WT300 Get Data.vi"("error in (no error)"=w1516, "VISA resource name"=w1496) -> ("error out"=w1515:errorcluster, "Power Data"=w1514:T27, "Yokogawa Data"=w1501:string[][])  [unwired: 4 in, 3 out]
            n543 = Unbundle By Name(w1514) -> ("Voltage (V):Element 1"=w1513:dbl, "Current (A):Element 1"=w1512:dbl, "Power (W):Sigma"=w1511:dbl, "Watt Hours (Wh):Sigma"=w1510:dbl, "Frequency (Hz):Element 1"=w1509:dbl, "Apparent Power (VA):Element 1"=w1508:dbl, "Power Factor:Element 1"=w1507:dbl, "Voltage Crest Factor:Element 1"=w1506:dbl, "Current Crest Factor:Element 1"=w1504:dbl, "Voltage Harmonic (%):Element 1"=w1505:dbl, "Time:Element 1"=w1503:dbl, "Watt Hours (Wh):Sigma"=w1500:dbl, "Max Watt Hours"=w1499:dbl)
            n544 = Build Array (concatenate)(w1517, w1501) -> (w1502:string[][])
            n545 = Max & Min(x=w1500, y=w1499) -> (max(x,y)=w1498:dbl)  [unwired: 1 out]
            n546 = Bundle By Name(cluster=w1519, "Total Array"=w1502, "Measurments.Power Measurements.Voltage (V):Element 1"=w1513, "Measurments.Power Measurements.Current (A):Element 1"=w1512, "Measurments.Power Measurements.Power (W):Sigma"=w1511, "Measurments.Power Measurements.Watt Hours (Wh):Sigma"=w1510, "Measurments.Power Measurements.Frequency (Hz):Element 1"=w1509, "Measurments.Power Measurements.Apparent Power (VA):Element 1"=w1508, "Measurments.Power Measurements.Power Factor:Element 1"=w1507, "Measurments.Power Measurements.Voltage Crest Factor:Element 1"=w1506, "Measurments.Power Measurements.Current Crest Factor:Element 1"=w1504, "Measurments.Power Measurements.Voltage Harmonic (%):Element 1"=w1505, "Measurments.Power Measurements.Time:Element 1"=w1503, "Measurments.Power Measurements.Max Watt Hours"=w1498) -> (w1518:T62)
          }
          frame "WT500" {
            n547 = call "WT500 Get Power Data.vi"("Error In"=w1549, "VISA resource name"=w1520) -> ("Error Out"=w1548:errorcluster, "Power Data Out"=w1545:T27, "Data Array"=w1526:string[][])  [unwired: 3 in, 3 out]
            n548 = Build Array (concatenate)(w1527, w1526) -> (w1525:string[][])
            n549 = Unbundle By Name(w1545) -> ("Voltage (V):Element 1"=w1544:dbl, "Voltage (V):Element 2"=w1524:dbl, "Current (A):Element 1"=w1543:dbl, "Current (A):Element 2"=w1542:dbl, "Power (W):Sigma"=w1541:dbl, "Watt Hours (Wh):Sigma"=w1540:dbl, "Current Crest Factor:Element 1"=w1539:dbl, "Current Crest Factor:Element 2"=w1538:dbl, "Voltage Harmonic (%):Element 1"=w1537:dbl, "Voltage Harmonic (%):Element 2"=w1536:dbl, "Voltage Crest Factor:Element 1"=w1535:dbl, "Voltage Crest Factor:Element 2"=w1534:dbl, "Time:Element 1"=w1533:dbl, "Frequency (Hz):Element 1"=w1532:dbl, "Apparent Power (VA):Element 1"=w1531:dbl, "Apparent Power (VA):Element 2"=w1530:dbl, "Power Factor:Element 1"=w1529:dbl, "Power Factor:Element 2"=w1528:dbl, "Watt Hours (Wh):Sigma"=w1523:dbl, "Max Watt Hours"=w1522:dbl)
            n550 = Max & Min(x=w1523, y=w1522) -> (max(x,y)=w1521:dbl)  [unwired: 1 out]
            n551 = Bundle By Name(cluster=w1547, "Total Array"=w1525, "Measurments.Power Measurements.Voltage (V):Element 1"=w1544, "Measurments.Power Measurements.Voltage (V):Element 2"=w1524, "Measurments.Power Measurements.Current (A):Element 1"=w1543, "Measurments.Power Measurements.Current (A):Element 2"=w1542, "Measurments.Power Measurements.Power (W):Sigma"=w1541, "Measurments.Power Measurements.Watt Hours (Wh):Sigma"=w1540, "Measurments.Power Measurements.Current Crest Factor:Element 1"=w1539, "Measurments.Power Measurements.Current Crest Factor:Element 2"=w1538, "Measurments.Power Measurements.Voltage Harmonic (%):Element 1"=w1537, "Measurments.Power Measurements.Voltage Harmonic (%):Element 2"=w1536, "Measurments.Power Measurements.Voltage Crest Factor:Element 1"=w1535, "Measurments.Power Measurements.Voltage Crest Factor:Element 2"=w1534, "Measurments.Power Measurements.Time:Element 1"=w1533, "Measurments.Power Measurements.Frequency (Hz):Element 1"=w1532, "Measurments.Power Measurements.Apparent Power (VA):Element 1"=w1531, "Measurments.Power Measurements.Apparent Power (VA):Element 2"=w1530, "Measurments.Power Measurements.Power Factor:Element 1"=w1529, "Measurments.Power Measurements.Power Factor:Element 2"=w1528, "Measurments.Power Measurements.Max Watt Hours"=w1521) -> (w1546:T62)
          }
          frame "Debug" {
          }
          frame "OSI" {
          }
        }
        n552 = Unbundle By Name(w1361) -> ("Measurments.Power Measurements.Power (W):Sigma"=→"Power (Watts)":dbl, "Measurments.Power Measurements.Voltage (V):Element 1"=→"Voltage":dbl)
        n553 = call <vilib>:"Add State(s) to Queue__jki_lib_state_machine.vi"("State(s) in (\"\")"=w1371) -> ("States Out"=w1370:string)  [unwired: 14 in]
      }
      frame "Gather Analog Data" {
        n554 = Unbundle By Name(w1562) -> ("Washer Controls Input.Test Fixture Hardware.Analog Data.Select Analog"=w1564:string, "Total Array"=w1563:string[][], "Washer Controls Input.Test Fixture Hardware"=w1560:T9, "Washer Controls Input.Test Fixture Hardware.Analog Data.NI Tasks (Dryer DOE)"=w1559:refnum<k21>[])
        n555 = local read "Water Temperature"() -> (w1557:dbl)
        n556 = local read "Hot Water Rate (GPM)"() -> (w1556:dbl)
        n557 = local read "Water Pressure"() -> (w1558:dbl)
        n558 = case shown="\"NI\"" w1564 {
          tunnel: w1566 -> [w1572 w1586 w1618 w1623 w1643 w1653 w1667 w1677 w1695 w1708 w1744 w1763 w1776 w1793 w1810]
          tunnel: [w1572 w1585 w1610 w1622 w1644 w1652 w1666 w1678 w1694 w1707 w1738 w1762 w1775 w1792 w1809] -> w1565
          tunnel: w1562 -> [_ w1598 w1612 w1621 w1637 w1654 w1668 w1681 w1696 w1706 w1745 _ w1772 w1789 w1806]
          tunnel: w1562 -> [w1571 w1596 w1617 w1625 w1639 w1651 w1665 w1680 w1693 w1709 w1741 w1757 w1774 w1791 w1808]
          tunnel: [w1570 w1595 w1616 w1624 w1638 w1650 w1664 w1679 w1692 w1710 w1740 w1760 w1773 w1790 w1807] -> w1555
          tunnel: w1563 -> [w1569 w1594 w1615 w1620 w1645 w1649 w1663 w1682 w1691 w1705 w1742 w1758 w1769 w1786 w1803]
          tunnel: "Disable Digital" -> [_ _ _ _ w1633 w1647 w1661 w1675 w1689 w1703 _ _ w1767 w1784 w1801]
          tunnel: w1560 -> [_ w1573 _ w1619 w1632 w1646 w1660 w1674 w1688 w1702 _ _ w1768 w1785 w1802]
          tunnel: w1559 -> [_ _ _ _ _ _ _ _ _ _ _ w1756 _ _ _]
          tunnel: w1558 -> [_ _ _ _ _ _ _ _ _ _ _ _ w1765 w1783 w1799]
          tunnel: w1557 -> [_ _ _ _ _ _ _ _ _ _ _ _ w1766 w1782 w1800]
          tunnel: w1556 -> [_ _ _ _ _ _ _ _ _ _ _ _ w1764 w1781 w1798]
          frame Default {
            n559 = Bundle By Name(cluster=w1571, "Total Array"=w1569) -> (w1570:T62)
          }
          frame "AGILENT" {
            # "Used in Washer DOE"
            # "Read all of the data and give\ndata in the correct order"
            n560 = Unbundle By Name(w1598) -> ("Washer Controls Input.Test Fixture Hardware.Analog Data.Agilent.TC Channels-List"=w1597:string, "Washer Controls Input.Test Fixture Hardware.Analog Data.Agilent.Analog Channels-List"=w1591:string, "Washer Controls Input.Test Fixture Hardware.Analog Data.Agilent.Agilent 34972_1"=w1588:refnum<visa-resource-name>, "Washer Controls Input.Test Fixture Hardware.Analog Data.TC Coefficients"=w1589:T13)
            n561 = Concatenate Strings(w1597, "," ("string"), w1591) -> (w1587:string)
            n562 = call "Agilent 34970 Get Data Main.vi"("error in (no error)"=w1586, "Analog Channels-List"=w1587, "VISA Refnum in"=w1588) -> ("error out"=w1585:errorcluster, "Sorted Data"=w1574:dbl[])  [unwired: 3 in, 4 out]
            n563 = call "DOE Parse Temperature and Voltage.vi"("Test Fixture Hardware"=w1573, "TC Coefficients"=w1589, "All Data"=w1574) -> ("DOE Agilent Data"=w1593:string[][], "Data Output"=w1584:T67)  [unwired: 6 in, 1 out]
            n564 = Unbundle By Name(w1584) -> ("Cold Water Pressure"=w1583:dbl, "Cold Water Pressure-Avg"=w1582:dbl, "Hot Water Pressure"=w1581:dbl, "Hot Water Pressure-Avg"=w1580:dbl, "Cold Water Temp"=w1579:dbl, "Cold Water Temp-Avg"=w1578:dbl, "Hot Water Temp"=w1577:dbl, "Hot Water Temp-Avg"=w1576:dbl, "Scale (lbs)"=w1575:dbl)
            n565 = Build Array (concatenate)(w1594, w1593) -> (w1592:string[][])
            n566 = Bundle By Name(cluster=w1596, "Total Array"=w1592, "Measurments.Water Measurements.Cold Water Pressure (psi)"=w1583, "Measurments.Water Measurements.Cold Water Pressure Max (psi)"=w1582, "Measurments.Water Measurements.Hot Water Pressure (psi)"=w1581, "Measurments.Water Measurements.Hot Water Pressure Max (psi)"=w1580, "Measurments.Water Measurements.Cold Water Temperature (°F)"=w1579, "Measurments.Water Measurements.Cold Water Temperature Max (°F)"=w1578, "Measurments.Water Measurements.Hot Water Temperature (°F)"=w1577, "Measurments.Water Measurements.Hot Water Temperature Max (°F)"=w1576, "Measurments.Weight Scale.Gross Weigth (lbs)"=w1575) -> (w1595:T62)
          }
          frame "ADVANTECH" {
            # "Used in Advanced Development Lab and Portable Stand (AP1 Component Lab)"
            n567 = Unbundle By Name(w1612) -> ("Washer Controls Input.Test Fixture Hardware.Analog Data.TC Coefficients"=w1611:T13)
            n568 = call "Advantech DAQ Get Data.vi"("Error In"=w1618, "TC Coefficients"=w1611) -> ("Error Out"=w1610:errorcluster, "Advantech"=w1609:T67, "Avantech DAQ"=w1614:string[][])  [unwired: 6 in, 1 out]
            n569 = Unbundle By Name(w1609) -> ("Cold Water Pressure"=w1608:dbl, "Cold Water Pressure-Avg"=w1607:dbl, "Hot Water Pressure"=w1606:dbl, "Hot Water Pressure-Avg"=w1605:dbl, "Cold Water Temp"=w1604:dbl, "Cold Water Temp-Avg"=w1603:dbl, "Hot Water Temp"=w1602:dbl, "Hot Water Temp-Avg"=w1601:dbl, "Ambient Temp"=w1600:dbl, "Room Humidity"=w1599:dbl)
            n570 = Build Array (concatenate)(w1615, w1614) -> (w1613:string[][])
            n571 = Bundle By Name(cluster=w1617, "Total Array"=w1613, "Measurments.Water Measurements.Cold Water Pressure (psi)"=w1608, "Measurments.Water Measurements.Cold Water Pressure Max (psi)"=w1607, "Measurments.Water Measurements.Hot Water Pressure (psi)"=w1606, "Measurments.Water Measurements.Hot Water Pressure Max (psi)"=w1605, "Measurments.Water Measurements.Cold Water Temperature (°F)"=w1604, "Measurments.Water Measurements.Cold Water Temperature Max (°F)"=w1603, "Measurments.Water Measurements.Hot Water Temperature (°F)"=w1602, "Measurments.Water Measurements.Hot Water Temperature Max (°F)"=w1601, "Measurments.Ambient Conditions.Ambient Temperature  1 (°F)"=w1600, "Measurments.Ambient Conditions.Ambient Humidity 1 (%)"=w1599) -> (w1616:T62)
          }
          frame "MW100" {
            # "Used in the New Kitchen"
            n572 = Unbundle By Name(w1621) -> ("Washer Controls Input.Test Fixture Hardware.Analog Data.Yokogawa.MW100"=w1627:refnum<visa-resource-name>, "Measurments"=w1628:T26)
            n573 = call "DOE Kitchen Agilent.vi"("Data Logger Type"=DOE_Data_Logger_Type."MW100", "error in (no error)"=w1623, "Test Fixture Hardware"=w1619, "Measurments"=w1628, "VISA Resource Name"=w1627) -> ("error out"=w1622:errorcluster, "Measurments Output"=w1630:T26, "Kitchen Analog Data"=w1631:string[][])  [unwired: 4 in]
            n574 = Build Array (concatenate)(w1620, w1631) -> (w1629:string[][])
            n575 = Bundle By Name(cluster=w1625, "Total Array"=w1629, "Measurments"=w1630) -> (w1624:T62)
          }
          frame "34972A_1" {
            # "Used in the Old Kitchen"
            n576 = Unbundle By Name(w1637) -> ("Washer Controls Input.Test Fixture Hardware.Analog Data.Agilent.Agilent 34972_1"=w1635:refnum<visa-resource-name>, "Measurments"=w1636:T26)
            n577 = call "DOE Kitchen Agilent.vi"("Data Logger Type"=DOE_Data_Logger_Type."Agilent", "Disable Digital"=w1633, "error in (no error)"=w1643, "Test Fixture Hardware"=w1632, "Measurments"=w1636, "VISA Resource Name"=w1635) -> ("error out"=w1644:errorcluster, "Measurments Output"=w1641:T26, "Kitchen Analog Data"=w1642:string[][])  [unwired: 3 in]
            n578 = Build Array (concatenate)(w1645, w1642) -> (w1640:string[][])
            n579 = Bundle By Name(cluster=w1639, "Total Array"=w1640, "Measurments"=w1641) -> (w1638:T62)
          }
          frame "34972A_2" {
            # "Used in the Old Kitchen"
            n580 = Unbundle By Name(w1654) -> ("Washer Controls Input.Test Fixture Hardware.Analog Data.Agilent.Agilent 34972_2"=w1655:refnum<visa-resource-name>, "Measurments"=w1656:T26)
            n581 = call "DOE Kitchen Agilent.vi"("Data Logger Type"=DOE_Data_Logger_Type."Agilent", "Disable Digital"=w1647, "error in (no error)"=w1653, "Test Fixture Hardware"=w1646, "Measurments"=w1656, "VISA Resource Name"=w1655) -> ("error out"=w1652:errorcluster, "Measurments Output"=w1658:T26, "Kitchen Analog Data"=w1659:string[][])  [unwired: 3 in]
            n582 = Build Array (concatenate)(w1649, w1659) -> (w1657:string[][])
            n583 = Bundle By Name(cluster=w1651, "Total Array"=w1657, "Measurments"=w1658) -> (w1650:T62)
          }
          frame "34972A_3" {
            # "Used in the Old Kitchen"
            n584 = Unbundle By Name(w1668) -> ("Washer Controls Input.Test Fixture Hardware.Analog Data.Agilent.Agilent 34972_3"=w1669:refnum<visa-resource-name>, "Measurments"=w1670:T26)
            n585 = call "DOE Kitchen Agilent.vi"("Data Logger Type"=DOE_Data_Logger_Type."Agilent", "Disable Digital"=w1661, "error in (no error)"=w1667, "Test Fixture Hardware"=w1660, "Measurments"=w1670, "VISA Resource Name"=w1669) -> ("error out"=w1666:errorcluster, "Measurments Output"=w1672:T26, "Kitchen Analog Data"=w1673:string[][])  [unwired: 3 in]
            n586 = Build Array (concatenate)(w1663, w1673) -> (w1671:string[][])
            n587 = Bundle By Name(cluster=w1665, "Total Array"=w1671, "Measurments"=w1672) -> (w1664:T62)
          }
          frame "34972A_4" {
            # "Used in the Old Kitchen"
            n588 = Unbundle By Name(w1681) -> ("Washer Controls Input.Test Fixture Hardware.Analog Data.Agilent.Agilent 34972_4"=w1683:refnum<visa-resource-name>, "Measurments"=w1684:T26)
            n589 = call "DOE Kitchen Agilent.vi"("Data Logger Type"=DOE_Data_Logger_Type."Agilent", "Disable Digital"=w1675, "error in (no error)"=w1677, "Test Fixture Hardware"=w1674, "Measurments"=w1684, "VISA Resource Name"=w1683) -> ("error out"=w1678:errorcluster, "Measurments Output"=w1686:T26, "Kitchen Analog Data"=w1687:string[][])  [unwired: 3 in]
            n590 = Build Array (concatenate)(w1682, w1687) -> (w1685:string[][])
            n591 = Bundle By Name(cluster=w1680, "Total Array"=w1685, "Measurments"=w1686) -> (w1679:T62)
          }
          frame "34972A_5" {
            # "Used in the Old Kitchen"
            n592 = Unbundle By Name(w1696) -> ("Washer Controls Input.Test Fixture Hardware.Analog Data.Agilent.Agilent 34972_5"=w1697:refnum<visa-resource-name>, "Measurments"=w1698:T26)
            n593 = call "DOE Kitchen Agilent.vi"("Data Logger Type"=DOE_Data_Logger_Type."Agilent", "Disable Digital"=w1689, "error in (no error)"=w1695, "Test Fixture Hardware"=w1688, "Measurments"=w1698, "VISA Resource Name"=w1697) -> ("error out"=w1694:errorcluster, "Measurments Output"=w1700:T26, "Kitchen Analog Data"=w1701:string[][])  [unwired: 3 in]
            n594 = Build Array (concatenate)(w1691, w1701) -> (w1699:string[][])
            n595 = Bundle By Name(cluster=w1693, "Total Array"=w1699, "Measurments"=w1700) -> (w1692:T62)
          }
          frame "34972A_6" {
            # "Used in the Old Kitchen"
            n596 = Unbundle By Name(w1706) -> ("Washer Controls Input.Test Fixture Hardware.Analog Data.Agilent.Agilent 34972_6"=w1711:refnum<visa-resource-name>, "Measurments"=w1712:T26)
            n597 = call "DOE Kitchen Agilent.vi"("Data Logger Type"=DOE_Data_Logger_Type."Agilent", "Disable Digital"=w1703, "error in (no error)"=w1708, "Test Fixture Hardware"=w1702, "Measurments"=w1712, "VISA Resource Name"=w1711) -> ("error out"=w1707:errorcluster, "Measurments Output"=w1714:T26, "Kitchen Analog Data"=w1715:string[][])  [unwired: 3 in]
            n598 = Build Array (concatenate)(w1705, w1715) -> (w1713:string[][])
            n599 = Bundle By Name(cluster=w1709, "Total Array"=w1713, "Measurments"=w1714) -> (w1710:T62)
          }
          frame "AGILENT_HCC" {
            w1724 = T52 0 items=["both", "start of string", "end of string"] ("location (both)")
            w1731 = T52 0 items=["both", "start of string", "end of string"] ("location (both)")
            n600 = Unbundle By Name(w1745) -> ("Washer Controls Input.Test Fixture Hardware.Analog Data.Agilent.Agilent 34972_2"=w1727:refnum<visa-resource-name>, "Washer Controls Input.Test Fixture Hardware.Analog Data.Agilent.Agilent 34972_1"=w1728:refnum<visa-resource-name>, "Washer Controls Input.Test Fixture Hardware.Analog Data.Agilent.TC Channels-List"=w1722:string, "Washer Controls Input.Test Fixture Hardware.Analog Data.Agilent.Analog Channels-List"=w1721:string, "Washer Controls Input.Test Fixture Hardware.Analog Data.Agilent.TC Channels-List 2"=w1725:string, "Washer Controls Input.Test Fixture Hardware.Analog Data.Agilent.Analog Channels-List 2"=w1733:string)
            n601 = Concatenate Strings(w1722, w1721) -> (w1723:string)
            n602 = Concatenate Strings(w1725, w1733) -> (w1732:string)
            n603 = call <vilib>:"Trim Whitespace.vi"("string"=w1723, "location (both)"=w1724) -> ("trimmed string"=w1720:string)
            n604 = call <vilib>:"Trim Whitespace.vi"("string"=w1732, "location (both)"=w1731) -> ("trimmed string"=w1726:string)
            n605 = call "Agilent 34970 Get Data Main.vi"("error in (no error)"=w1744, "Analog Channels-List"=w1720, "VISA Refnum in"=w1728) -> ("error out"=w1737:errorcluster, "Sorted Data"=w1716:dbl[], "Names"=w1718:string[])  [unwired: 3 in, 3 out]
            n606 = String Length(string=w1726) -> (length=w1730:i32)
            n607 = Greater Than 0?(x=w1730) -> (x > 0?=w1729:bool)
            n608 = case shown="True" w1729 {
              tunnel: w1737 -> [w1748 w1754]
              tunnel: w1727 -> [_ w1753]
              tunnel: [dbl[] [] ("Output Data Permutation") w1749] -> w1736
              tunnel: [w1748 w1752] -> w1734
              tunnel: w1726 -> [_ w1751]
              tunnel: [string[] [] ("Names") w1750] -> w1719
              frame False {
              }
              frame True {
                n609 = call "Agilent 34970 Get Data Main.vi"("error in (no error)"=w1754, "Analog Channels-List"=w1751, "VISA Refnum in"=w1753) -> ("error out"=w1752:errorcluster, "Sorted Data"=w1749:dbl[], "Names"=w1750:string[])  [unwired: 3 in, 3 out]
              }
            }
            n610 = Build Array (concatenate)(w1718, w1719) -> (w1717:string[])
            n611 = Build Array (concatenate)(w1716, w1736) -> (w1735:dbl[])
            n612 = call "DOE Washer HCC Labels AGILENT.vi"("Names"=w1717, "Error In"=w1734, "Agilent Data Input"=w1735) -> ("Error Out"=w1738:errorcluster, "HCC Data Output"=w1743:string[][])  [unwired: 7 in]
            n613 = Build Array (concatenate)(w1742, w1743) -> (w1739:string[][])
            n614 = Bundle By Name(cluster=w1741, "Total Array"=w1739) -> (w1740:T62)
          }
          frame "NI" {
            # "Using this section for Dryer Performance"
            n615 = call "DPT GET NI Data.vi"("NI Card Settings"="NI Card Settings", "Error In"=w1763, "Tasks In"=w1756) -> ("Error Out"=w1762:errorcluster, "cDAQ Data"=w1759:string[][])  [unwired: 7 in]
            n616 = Build Array (concatenate)(w1758, w1759) -> (w1761:string[][])
            n617 = Bundle By Name(cluster=w1757, "Total Array"=w1761) -> (w1760:T62)
          }
          frame "34970A_DISH_DOE_1" {
            # "Used in Kitchen DOE"
            n618 = Unbundle By Name(w1772) -> ("Washer Controls Input.Test Fixture Hardware.Analog Data.Agilent.Agilent 34972_1"=w1771:refnum<visa-resource-name>, "Measurments"=w1770:T26)
            n619 = call "DOE Kitchen Agilent.vi"("Flow Rate"=w1764, "Water Pressure"=w1765, "Data Logger Type"=DOE_Data_Logger_Type."Agilent_Laurel_DC_Clamp", "Disable Digital"=w1767, "Water Temperature"=w1766, "error in (no error)"=w1776, "Test Fixture Hardware"=w1768, "Measurments"=w1770, "VISA Resource Name"=w1771) -> ("error out"=w1775:errorcluster, "Measurments Output"=w1779:T26, "Kitchen Analog Data"=w1780:string[][])
            n620 = Build Array (concatenate)(w1769, w1780) -> (w1778:string[][])
            n621 = Bundle By Name(cluster=w1774, "Total Array"=w1778, "Measurments"=w1779) -> (w1773:T62)
          }
          frame "34970A_DISH_DOE_2" {
            # "Used in Kitchen DOE"
            n622 = Unbundle By Name(w1789) -> ("Washer Controls Input.Test Fixture Hardware.Analog Data.Agilent.Agilent 34972_2"=w1788:refnum<visa-resource-name>, "Measurments"=w1787:T26)
            n623 = call "DOE Kitchen Agilent.vi"("Flow Rate"=w1781, "Water Pressure"=w1783, "Data Logger Type"=DOE_Data_Logger_Type."Agilent_Laurel_DC_Clamp", "Disable Digital"=w1784, "Water Temperature"=w1782, "error in (no error)"=w1793, "Test Fixture Hardware"=w1785, "Measurments"=w1787, "VISA Resource Name"=w1788) -> ("error out"=w1792:errorcluster, "Measurments Output"=w1796:T26, "Kitchen Analog Data"=w1797:string[][])
            n624 = Build Array (concatenate)(w1786, w1797) -> (w1795:string[][])
            n625 = Bundle By Name(cluster=w1791, "Total Array"=w1795, "Measurments"=w1796) -> (w1790:T62)
          }
          frame "34970A_DISH_DOE_3" {
            # "Used in Kitchen DOE"
            n626 = Unbundle By Name(w1806) -> ("Washer Controls Input.Test Fixture Hardware.Analog Data.Agilent.Agilent 34972_3"=w1805:refnum<visa-resource-name>, "Measurments"=w1804:T26)
            n627 = call "DOE Kitchen Agilent.vi"("Flow Rate"=w1798, "Water Pressure"=w1799, "Data Logger Type"=DOE_Data_Logger_Type."Agilent_Laurel_DC_Clamp", "Disable Digital"=w1801, "Water Temperature"=w1800, "error in (no error)"=w1810, "Test Fixture Hardware"=w1802, "Measurments"=w1804, "VISA Resource Name"=w1805) -> ("error out"=w1809:errorcluster, "Measurments Output"=w1813:T26, "Kitchen Analog Data"=w1814:string[][])
            n628 = Build Array (concatenate)(w1803, w1814) -> (w1812:string[][])
            n629 = Bundle By Name(cluster=w1808, "Total Array"=w1812, "Measurments"=w1813) -> (w1807:T62)
          }
        }
        n630 = call <vilib>:"Add State(s) to Queue__jki_lib_state_machine.vi"("State(s) in (\"\")"=w1568) -> ("States Out"=w1567:string)  [unwired: 14 in]
        n631 = Unbundle By Name(w1555) -> ("Measurments.Water Measurements.Hot Water Temperature (°F)"=→"Water Temperature (°F)":dbl)
      }
      frame "Get Temp and Humidity" {
        w1829 = u16 2000 ("Remote Port")
        n632 = Unbundle By Name(w1842) -> ("Total Array"=w1840:string[][], "Washer Controls Input.Test Fixture Hardware.ITHX-Temp Humidity.IP Address 1"=w1844:string, "Washer Controls Input.Test Fixture Hardware.ITHX-Temp Humidity.IP Address 2"=w1831:string, "Washer Controls Input.Test Fixture Hardware.ITHX-Temp Humidity.IP Address 3"=w1830:string)
        n633 = call "Newport ITX-D3N.vi"("Device Number (Display In Header)"="1", "error in (no error)"=w1843, "Remote Port"=w1829, "Machine"=w1844) -> ("error out"=w1834:errorcluster, "iTHX/iBTHX Output"=w1837:T68, "Newport ITX Data"=w1839:string[][])  [unwired: 4 in, 1 out]
        n634 = call "Newport ITX-D3N.vi"("Device Number (Display In Header)"="2", "error in (no error)"=w1834, "Remote Port"=w1829, "Machine"=w1831) -> ("error out"=w1833:errorcluster, "iTHX/iBTHX Output"=w1828:T68, "Newport ITX Data"=w1820:string[][])  [unwired: 4 in, 1 out]
        n635 = call "Newport ITX-D3N.vi"("Device Number (Display In Header)"="3", "error in (no error)"=w1833, "Remote Port"=w1829, "Machine"=w1830) -> ("error out"=w1832:errorcluster, "iTHX/iBTHX Output"=w1827:T68, "Newport ITX Data"=w1819:string[][])  [unwired: 4 in, 1 out]
        n636 = Unbundle By Name(w1837) -> ("iBTHX Temperature (°F)"=w1815:dbl, "iBTHX Humidity (%)"=w1836:dbl, "iBTHX DewPoint Temp"=w1835:dbl)
        "Room Temperature" <- w1815
        n637 = Unbundle By Name(w1828) -> ("iBTHX Temperature (°F)"=w1826:dbl, "iBTHX Humidity (%)"=w1825:dbl, "iBTHX DewPoint Temp"=w1824:dbl)
        n638 = Unbundle By Name(w1827) -> ("iBTHX Temperature (°F)"=w1823:dbl, "iBTHX Humidity (%)"=w1822:dbl, "iBTHX DewPoint Temp"=w1821:dbl)
        n639 = call <vilib>:"Add State(s) to Queue__jki_lib_state_machine.vi"("State(s) in (\"\")"=w1846) -> ("States Out"=w1845:string)  [unwired: 14 in]
        n640 = Build Array (concatenate)(w1840, w1839, w1820, w1819) -> (w1838:string[][])
        n641 = Bundle By Name(cluster=w1842, "Total Array"=w1838, "Measurments.Ambient Conditions.Ambient Temperature  1 (°F)"=w1815, "Measurments.Ambient Conditions.Ambient Humidity 1 (%)"=w1836, "Measurments.Ambient Conditions.Ambient Dewpoint  1 (°F)"=w1835, "Measurments.Ambient Conditions.Ambient Temperature 2 (°F)"=w1826, "Measurments.Ambient Conditions.Ambient Humidity 2 (%)"=w1825, "Measurments.Ambient Conditions.Ambient Dewpoint 2 (°F)"=w1824, "Measurments.Ambient Conditions.Ambient Temperature 3 (°F)"=w1823, "Measurments.Ambient Conditions.Ambient Humidity 3 (%)"=w1822, "Measurments.Ambient Conditions.Ambient Dewpoint 3 (°F)"=w1821) -> (w1841:T62)
      }
      frame "Get Barometric Pressure" {
        n642 = Unbundle By Name(w1855) -> ("Total Array"=w1848:string[][], "Washer Controls Input.Test Fixture Hardware.Barometric Pressure.HEISE 901A"=w1850:refnum<visa-resource-name>, "Washer Controls Input.Test Fixture Hardware.Barometric Pressure.Use Barometer?"=w1851:bool)
        n643 = case shown="True" w1851 {
          tunnel: w1853 -> [w1860 w1867]
          tunnel: [w1860 w1866] -> w1852
          tunnel: w1850 -> [_ w1865]
          tunnel: [0.0 ("Barometric Pressure (in Hg)") w1864] -> w1849
          tunnel: w1848 -> [w1858 w1862]
          tunnel: [w1858 w1861] -> w1847
          frame False {
          }
          frame True {
            n644 = call "Heise Barometric Pressure 901A Send Receive.vi"("error in (no error)"=w1867, "VISA Refnum in"=w1865) -> ("error out"=w1866:errorcluster, "Barometric Data"=w1863:string[], "Barometric Pressure (in Hg)"=w1864:dbl)  [unwired: 6 in, 1 out]
            n645 = Build Array (concatenate)(w1862, w1863) -> (w1861:string[][])
          }
        }
        n646 = call <vilib>:"Add State(s) to Queue__jki_lib_state_machine.vi"("State(s) in (\"\")"=w1857) -> ("States Out"=w1856:string)  [unwired: 14 in]
        n647 = Bundle By Name(cluster=w1855, "Total Array"=w1847, "Measurments.Barometric Pressure.Barometric Pressure (in. Hg)"=w1849) -> (w1854:T62)
      }
      frame "Gather Flow Rates" {
        n648 = Unbundle By Name(w1876) -> ("Total Array"=w1874:string[][], "Washer Controls Input.Test Fixture Hardware.Flow Rates.Meters To Collect (Hot Cold)"=w1869:string, "Measurments"=→"Measurments 2":T26, "Washer Controls Input.Test Fixture Hardware"=→"Fixture Hardware":T9)
        n649 = local read "Measurments Output"() -> (w1870:T26)
        n650 = case shown="\"HOT\"" w1869 {
          tunnel: w1876 -> [w1881 w1897 w1906]
          tunnel: [w1880 w1896 w1905] -> w1875
          tunnel: w1874 -> [w1879 w1895 w1904]
          tunnel: w1872 -> [w1882 w1885 w1900]
          tunnel: [w1882 w1885 w1900] -> w1871
          tunnel: w1870 -> [_ w1883 w1899]
          frame Default {
            n651 = Bundle By Name(cluster=w1881, "Total Array"=w1879) -> (w1880:T62)
          }
          frame "HOT COLD" {
            # "Data type set in Laurel Loop"
            # "Washers have everything. So collect\nall."
            n652 = local read "Header Data"() -> (w1884:string[][])
            n653 = Unbundle By Name(w1883) -> ("Water Measurements.Hot Water Total (Gal)"=w1893:dbl, "Water Measurements.Hot Water Rate (GPM)"=w1892:dbl, "Water Measurements.Cold Water Total (Gal)"=w1891:dbl, "Water Measurements.Cold Water Rate (GPM)"=w1890:dbl, "Water Measurements.Cold Water Total During Wash (Gal)"=w1889:dbl, "Water Measurements.Hot Water Total During Wash (Gal)"=w1888:dbl, "Water Measurements.Rinse Cold (Gal)"=w1887:dbl, "Water Measurements.Rinse Hot (Gal)"=w1886:dbl)
            n654 = Build Array (concatenate)(w1895, w1884) -> (w1894:string[][])
            n655 = Bundle By Name(cluster=w1897, "Total Array"=w1894, "Measurments.Water Measurements.Hot Water Total (Gal)"=w1893, "Measurments.Water Measurements.Hot Water Rate (GPM)"=w1892, "Measurments.Water Measurements.Cold Water Total (Gal)"=w1891, "Measurments.Water Measurements.Cold Water Rate (GPM)"=w1890, "Measurments.Water Measurements.Cold Water Total During Wash (Gal)"=w1889, "Measurments.Water Measurements.Hot Water Total During Wash (Gal)"=w1888, "Measurments.Water Measurements.Rinse Cold (Gal)"=w1887, "Measurments.Water Measurements.Rinse Hot (Gal)"=w1886) -> (w1896:T62)
          }
          frame "HOT" {
            # "Data type set in Laurel Loop"
            # "Dishwashers only have hot water. Therefore only collect the \nhot water laurel"
            n656 = local read "Header Data"() -> (w1898:string[][])
            n657 = Build Array (concatenate)(w1904, w1898) -> (w1902:string[][])
            n658 = Unbundle By Name(w1899) -> ("Water Measurements.Hot Water Total (Gal)"=w1903:dbl, "Water Measurements.Hot Water Rate (GPM)"=w1901:dbl)
            n659 = Bundle By Name(cluster=w1906, "Total Array"=w1902, "Measurments.Water Measurements.Hot Water Total (Gal)"=w1903, "Measurments.Water Measurements.Hot Water Rate (GPM)"=w1901) -> (w1905:T62)
          }
        }
        n660 = call <vilib>:"Add State(s) to Queue__jki_lib_state_machine.vi"("State(s) in (\"\")"=w1878) -> ("States Out"=w1877:string)  [unwired: 14 in]
      }
      frame "Get Scale Data" {
        n661 = Unbundle By Name(w1911) -> ("Washer Controls Input.Test Fixture Hardware.Weight Scale.Select Scale"=w1908:string)
        n662 = Equal?(x=w1908, y="") -> (x = y?=w1907:bool)
        n663 = case shown="False" w1907 {
          tunnel: w1911 -> [w1915 w1917]
          tunnel: [w1915 w1921] -> w1910
          frame True {
          }
          frame False {
            # "Had to offload. Due to the timing being too long..."
            n664 = local read "Weight Data"() -> (w1922:string[][])
            n665 = Unbundle By Name(w1917) -> ("Total Array"=w1916:string[][])
            n666 = call "DOE Extract Weight Data.vi"("Weight Data"=w1922, "Total Array"=w1916) -> ("Net Weight (lbs)"=w1918:dbl, "Gross Weight (lbs)"=w1919:dbl, "Total Array Output"=w1920:string[][])  [unwired: 6 in, 1 out]
            n667 = Bundle By Name(cluster=w1917, "Total Array"=w1920, "Measurments.Weight Scale.Gross Weigth (lbs)"=w1919, "Measurments.Weight Scale.Net Weight (lbs)"=w1918) -> (w1921:T62)
          }
        }
        n668 = call <vilib>:"Add State(s) to Queue__jki_lib_state_machine.vi"("State(s) in (\"\")"=w1914) -> ("States Out"=w1913:string)  [unwired: 14 in]
      }
      frame "Get Gas Data" {
        # "I have to do this because the mass flow meter and \nWT500 do not play nice together. It will error out the \nWT500 if the communication is not isolated."
        n669 = Unbundle By Name(w1943) -> ("Total Array"=w1941:string[][], "Measurments.Barometric Pressure.Barometric Pressure (in. Hg)"=w1937:dbl)
        n670 = local read "DAQ Data Out"() -> (w1934:T40)
        n671 = call "FMA1600A Dryer Data Build.vi"("Barometric Pressure.Barometric Pressure (in. Hg)"=w1937, "Error In"=w1936, "DAQ Data In in"=w1934) -> ("Error Out"=w1940:errorcluster, "LPM (Vol. Flow)"=w1935:dbl, "Dryer Data"=w1939:string[][])  [unwired: 6 in]
        n672 = Build Array (concatenate)(w1941, w1939) -> (w1938:string[][])
        n673 = Unbundle By Name(w1934) -> ("Meter Bank 1.Panel Data.Heating Value (BTU/ft³)"=w1931:dbl, "Meter Bank 1.Panel Data.Ft³ / Hr (SCFH)"=w1932:dbl, "Meter Bank 1.Panel Data.15 Second Average (BTU/HR)"=w1923:dbl, "Meter Bank 1.Panel Data.30 Second Average (BTU/HR)"=w1924:dbl, "Meter Bank 1.Panel Data.Mass Flow"=w1925:dbl, "Meter Bank 1.Panel Data.Vol. Flow"=w1926:dbl, "Meter Bank 1.Panel Data.Gas Temperature"=w1927:dbl, "Meter Bank 1.Panel Data.Gas Pressure"=w1928:dbl, "Meter Bank 1.Panel Data.Tot.Flow"=w1929:dbl, "Meter Bank 1.Panel Data.Meter Type (Gas)"=w1930:T30)
        n674 = Bundle By Name(cluster=w1943, "Total Array"=w1938, "Measurments.Gas Data.Tot.Flow (Liters)"=w1935, "Measurments.Gas Data.Meter ID"=RANGE_Meter_Selector_1-2."Meter 1", "Measurments.Gas Data.Heating Value (BTU/ft³)"=w1931, "Measurments.Gas Data.Ft³ / Hr (SCFH)"=w1932, "Measurments.Gas Data.15 Second Average (BTU/HR)"=w1923, "Measurments.Gas Data.30 Second Average (BTU/HR)"=w1924, "Measurments.Gas Data.SLPM (Mass Flow)"=w1925, "Measurments.Gas Data.LPM (Vol. Flow)"=w1926, "Measurments.Gas Data.Gas Temperature (°F)"=w1927, "Measurments.Gas Data.Gas Pressure (PSIA)"=w1928, "Measurments.Gas Data.Tot.Flow (Liters)"=w1929, "Measurments.Gas Data.Meter Type (Gas)"=w1930) -> (w1942:T62)
        n675 = call <vilib>:"Add State(s) to Queue__jki_lib_state_machine.vi"("State(s) in (\"\")"=w1945) -> ("States Out"=w1944:string)  [unwired: 14 in]
      }
      frame "Dryer RMC Data" {
        n676 = Unbundle By Name(w1961) -> ("Total Array"=w1955:string[][], "Washer Controls Input.Initialize.Washer In.Appliance Details.Dryer.Dryer Initial IMC Data.Empty Dryer Cold Weigth"=→"Cold Dryer Weight (lbs)":dbl, "Washer Controls Input.Initialize.Washer In.Appliance Details.Appliance Common"=w1952:T20, "Measurments"=w1947:T26, "Washer Controls Input.Initialize.Washer In.Appliance Details.Dryer.Dryer Initial IMC Data"=w1954:T22)
        n677 = call "DOE Dryer EF Calculations.vi"("Est. Power (Watts)"="Est. Power (Watts)", "Use Estimated Standby Power"="Use Estimated Standby Power", "Use Runtime RMC Calculation?"=TRUE, "Error In"=w1958, "Dryer Initial IMC Data"=w1954, "Measurments"=w1947, "Appliance Common"=w1952) -> ("Error Out"=w1950:errorcluster, "Dryer Initial IMC Data Out"=w1953:T22, "Measurments Out"=w1948:T26, "RMC Data"=w1949:string[][])  [unwired: 1 in]
        n678 = Build Array (concatenate)(w1955, w1949) -> (w1959:string[][])
        n679 = Bundle By Name(cluster=w1961, "Total Array"=w1959, "Measurments"=w1948, "Washer Controls Input.Initialize.Washer In.Appliance Details.Dryer.Dryer Initial IMC Data"=w1953) -> (w1960:T62)
        n680 = call <vilib>:"Add State(s) to Queue__jki_lib_state_machine.vi"("State(s) in (\"\")"=w1963) -> ("States Out"=w1962:string)  [unwired: 14 in]
      }
      frame "Check Newfi" {
        n681 = Unbundle By Name(w1980) -> ("Measurments.Power Measurements.Power (W):Sigma"=→"P:Sigma":dbl, "Total Array"=w1973:string[][], "Force Read Point"=w1966:bool)
        n682 = local read "Standard GEA2"() -> (w1972:string[][])
        n683 = Build Array (concatenate)(w1973, w1972) -> (w1970:string[][])
        n684 = Transpose 2D Array(2D array=w1970) -> (transposed array=w1969:string[][])
        n685 = local read "Point File Path"() -> (w1977:path)
        n686 = call "RTS Build Point File Data.vi"("Force Read Point?"=w1966, "Disable System Time Filter"=TRUE, "Full List Box Data"=w1969, "Point File Location"=w1977) -> ("Custom Titles"=w1974:string[], "Custom Listbox Data"=w1975:string[][])  [unwired: 4 in, 2 out]
        n687 = local read "Limit Reached"() -> (w1978:bool)
        n688 = Replace Array Subset(array=w1975, new element=w1974, index (row)=0 ("disabled index (col)")) -> (w1964:string[][])  [unwired: 1 in]
        n689 = Transpose 2D Array(2D array=w1964) -> (transposed array=→"Data":string[][])
        n690 = And(x="Auto-Terminate Prog", y=w1978) -> (x .and. y?=w1981:bool)
        n691 = case shown="True" w1981 {
          tunnel: ["" "Add Final Data"] -> w1982
          frame False {
          }
          frame True {
          }
        }
        n692 = Bundle By Name(cluster=w1980, "Force Read Point"=FALSE, "Full Data Output"=w1970, "Save Data"=w1964) -> (w1979:T62)
        n693 = call <vilib>:"Add State(s) to Queue__jki_lib_state_machine.vi"("State(s) in Front (\"\")"=w1982, "State(s) in (\"\")"=w1986) -> ("States Out"=w1985:string)  [unwired: 13 in]
      }
      frame "Show Data" {
        # "The Washer and Dishwasher have different outputs. Therefore\ndistinguish between them"
        n694 = Unbundle By Name(w2002) -> ("Plot Array"=w1998:dbl[][], "Save Data"=w2003:string[][], "Measurments.Water Measurements.Hot Water Total (Gal)"=→"Hot Total Usage (Gal)":dbl, "Measurments.Water Measurements.Cold Water Total (Gal)"=→"Cold Total Usage (Gal)":dbl, "Filepath.Data File Paths.Data File Path"=w1997:path)
        n695 = local read "Dishwasher Events Visible"() -> (w1999:bool)
        n696 = case shown="True" w1999 {
          tunnel: w2002 -> [_ w2018]
          frame False {
          }
          frame True {
            n697 = Unbundle By Name(w2018) -> ("Measurments.Dishwasher.Drain Solonoid Event"=w2019:i32, "Measurments.Dishwasher.Pump Event"=w2020:i32, "Measurments.Dishwasher.Water Valve Event"=w2021:i32, "Measurments.Dishwasher.Heater Event"=w2022:i32, "Measurments.Dishwasher.Motor Event"=w2023:i32)
            n698 = Not Equal To 0?(x=w2019) -> (x != 0?=w2026:bool)
            n699 = Not Equal To 0?(x=w2020) -> (x != 0?=w2027:bool)
            n700 = Not Equal To 0?(x=w2021) -> (x != 0?=w2028:bool)
            n701 = Not Equal To 0?(x=w2022) -> (x != 0?=w2029:bool)
            n702 = Not Equal To 0?(x=w2023) -> (x != 0?=w2030:bool)
            n703 = Bundle By Name(cluster=T2 {"Drain Pump"=FALSE, "Circ Pump"=FALSE, "Water Valve"=FALSE, "Heater"=FALSE, "Extra"=FALSE} ("Dishwasher Events"), "Drain Pump"=w2026, "Circ Pump"=w2027, "Water Valve"=w2028, "Heater"=w2029, "Extra"=w2030) -> (→"Dishwasher Events":T2)
          }
        }
        n704 = local read "Max File Size"() -> (w1993:dbl)
        n705 = call "Save File Max Size Runtime.vi"("File Size"=w1993, "Old path"=w1997) -> ("New File"=w1992:bool, "New Path"=w1996:path)  [unwired: 7 in, 1 out]
        n706 = call "UTILITY Create Plot Array.vi"("Save Data"=w2003, "Plot Array in"=w1998) -> ("Plot Array out"=w1991:dbl[][])  [unwired: 8 in, 1 out]
        "Plot Array" <- w1991
        n707 = call <vilib>:"Add State(s) to Queue__jki_lib_state_machine.vi"("State(s) in (\"\")"=w2005) -> ("States Out"=w2004:string)  [unwired: 14 in]
        n708 = case shown="False" "Disable Plot" {
          tunnel: w2003 -> [w2012 _]
          tunnel: w1991 -> [w2006 _]
          frame False {
            n709 = call "UTILITY MultiPlot.vi"("Y-Axis-2"="Y-Axis-2", "Y-Axis-1"="Y-Axis-1", "X-Axis"="X-Axis", "Save Data"=w2012, "Plot Array"=w2006) -> ("Plot Cluster"=w2009:T3)  [unwired: 5 in, 1 out]
            n710 = case shown="False" "Pause Graph" {
              tunnel: w2009 -> [w2013 _]
              frame False {
                "XY Graph" <- w2013
              }
              frame True {
              }
            }
          }
          frame True {
          }
        }
        n711 = Bundle By Name(cluster=w2002, "Plot Array"=w1991, "Filepath.Data File Paths.Data File Path"=w1996, "New File"=w1992) -> (w1995:T62)
        n712 = case shown="True" w1992 {
          tunnel: w1995 -> [w2014 w2017]
          tunnel: [w2014 w2016] -> w1994
          frame False {
          }
          frame True {
            n713 = Bundle By Name(cluster=w2017, "Plot Array"=dbl[][] [[0.0, 0.0, 0.0], [0.0, 0.0, 0.0]]) -> (w2016:T62)
          }
        }
      }
      frame "Save Data" {
        # "Need to common with HEWH."
        n714 = Unbundle By Name(w2043) -> ("New File"=w2042:bool, "Filepath.Data File Paths.Data File Path"=w2033:path, "Washer Controls Input.Initialize.Washer In.Appliance Details.File Name Output Array"=w2031:string[][], "Save Data"=w2036:string[][])
        "Save Path" <- w2033
        "Save Data" <- w2036
        n715 = local read "Start Saving Data"() -> (w2041:bool)
        n716 = property on="Data File Path" class="Path"("Value"=w2033) -> ()  [unwired: 2 in, 2 out]
        n717 = Not Equal?(x=w2033, y=path "") -> (x != y?=w2037:bool)
        n718 = Equal?(x=TRUE, y=w2041) -> (x = y?=w2039:bool)
        n719 = Compound Arithmetic op=AND(w2039, w2037) -> (w2032:bool)
        n720 = case shown="True" w2032 {
          tunnel: w2033 -> [_ w2055]
          tunnel: w2035 -> [w2047 w2054]
          tunnel: [w2047 w2054] -> w2034
          tunnel: w2036 -> [_ w2049]
          tunnel: w2031 -> [_ w2048]
          frame False {
            n721 = local write "Test Status"("Not Collecting Data...." ("Test Status")) -> ()
          }
          frame True {
            n722 = local read "Write Header"() -> (w2052:bool)
            n723 = First Call?() -> (First Call?: T/F=w2053:bool)
            n724 = Or(x=w2053, y=w2052) -> (x .or. y?=w2051:bool)
            n725 = case shown="False" w2051 {
              tunnel: w2048 -> [_ w2067]
              tunnel: w2049 -> [w2061 w2066]
              tunnel: w2055 -> [w2057 w2062]
              frame False {
                # "Delete the header and only put the data in the file"
                n726 = Index Array(array=w2061, index (row)=1) -> (element=w2059:string[])  [unwired: 1 in]
                n727 = call-poly <vilib>:"Write Delimited Spreadsheet.vi"("file path (dialog if empty)"=w2057, "1D data"=w2059, "append to file? (new file:F)"=TRUE, "delimiter (\\t)"="," ("delimiter (\\t)")) -> ()  [unwired: 10 in, 2 out]
              }
              frame True {
                n728 = Build Array (concatenate)(w2067, w2066) -> (w2063:string[][])
                n729 = local write "Write Header"(FALSE ("Write Header")) -> ()
                n730 = call-poly <vilib>:"Write Delimited Spreadsheet.vi"("file path (dialog if empty)"=w2062, "2D data"=w2063, "delimiter (\\t)"="," ("delimiter (\\t)")) -> ()  [unwired: 11 in, 2 out]
              }
            }
            "Test Status" <- "Collecting Data...." ("Test Status")
          }
        }
        n731 = call <vilib>:"Add State(s) to Queue__jki_lib_state_machine.vi"("State(s) in (\"\")"=w2045) -> ("States Out"=w2044:string)  [unwired: 14 in]
        n732 = case shown="True" w2042 {
          frame False {
          }
          frame True {
            n733 = local write "Write Header"(TRUE ("Write Header")) -> ()
          }
        }
      }
      frame "--------- Export Data ---------" {
        n734 = call <vilib>:"Add State(s) to Queue__jki_lib_state_machine.vi"("State(s) in (\"\")"=w2072) -> ("States Out"=w2071:string)  [unwired: 14 in]
      }
      frame "Add Final Data" {
        # "Not best solution...but \ncuts down on memory usage"
        # "I am using this as a trigger. This is lazy. Fix later"
        n735 = Unbundle By Name(w2076) -> ("Washer Controls Input.Test Fixture Hardware.Weight Scale.Com Options.Setra Scale VISA"=w2075:refnum<visa-resource-name>)
        n736 = local read "Front Program Name"() -> (w2083:string)
        n737 = disable-structure shown="Disabled" {
          frame Disabled {
            n738 = call "Setra Main.vi"() -> ()  [unwired: 13 in, 3 out]
          }
          frame Enabled {
          }
        }
        n739 = call "DOE Search Program Name.vi"("Program Name"=w2083) -> ("LV Program"=w2081:T49)  [unwired: 10 in]
        n740 = local read "Use Estimated Standby Power"() -> (w2074:bool)
        n741 = local read "Est. Power (Watts)"() -> (w2073:dbl)
        n742 = case shown="\"Dryer\"" w2081 {
          tunnel: w2082 -> [w2094 w2100]
          tunnel: w2075 -> [_ w2099]
          tunnel: [w2094 w2112] -> w2080
          tunnel: w2076 -> [w2093 w2105]
          tunnel: [w2093 w2102] -> w2079
          tunnel: w2074 -> [_ w2107]
          tunnel: w2073 -> [_ w2106]
          frame Default {
          }
          frame "Dryer" {
            n743 = call "ICS425.vi"("VISA resource name"=w2099, "Runtime Gather?"=FALSE, "Error In"=w2100) -> ("Weight Output"=w2096:dbl, "Weight Output (string)"=w2095:string, "Error Out"=w2097:errorcluster)  [unwired: 10 in]
            n744 = Bundle By Name(cluster=w2105, "Measurments.Weight Scale.Gross Weigth (lbs)"=w2096, "Measurments.Weight Scale.Final Weight (lbs)"=w2095) -> (w2111:T62)
            n745 = Unbundle By Name(w2111) -> ("Washer Controls Input.Initialize.Washer In.Appliance Details.Appliance Common"=w2110:T20, "Measurments"=w2109:T26, "Washer Controls Input.Initialize.Washer In.Appliance Details.Dryer.Dryer Initial IMC Data"=w2108:T22)
            n746 = call "DOE Dryer EF Calculations.vi"("Est. Power (Watts)"=w2106, "Use Estimated Standby Power"=w2107, "Use Runtime RMC Calculation?"=FALSE, "Error In"=w2097, "Dryer Initial IMC Data"=w2108, "Measurments"=w2109, "Appliance Common"=w2110) -> ("Error Out"=w2112:errorcluster, "Dryer Initial IMC Data Out"=w2103:T22, "Measurments Out"=w2104:T26)  [unwired: 1 in, 1 out]
            n747 = Bundle By Name(cluster=w2105, "Measurments"=w2104, "Washer Controls Input.Initialize.Washer In.Appliance Details.Dryer.Dryer Initial IMC Data"=w2103) -> (w2102:T62)
          }
        }
        n748 = Unbundle By Name(w2079) -> ("Filepath.Data File Paths.Data File Path"=w2088:path, "Measurments"=w2087:T26, "Washer Controls Input.Initialize.Washer In.Appliance Details.Dryer.Dryer Initial IMC Data"=w2078:T22)
        n749 = local read "Elapsed Time"() -> (w2077:T33)
        n750 = call "DOE Add Final Headers.vi"("Elapsed Time"=w2077, "Dryer Initial IMC Data"=w2078, "Program Name"=w2083, "error in (no error)"=w2080, "Measurments"=w2087, "Data File Path"=w2088) -> ("error out"=w2089:errorcluster)  [unwired: 5 in]
        n751 = flat-sequence {
          tunnel: w2089 -> [w2119]
          tunnel: [w2119] -> w2084
          frame #0 {
            w2117 = FALSE ("Auto-Terminate Prog")
            n752 = local write "Auto-Terminate Prog"(w2117) -> ()
            n753 = local write "Start Saving Data"(FALSE ("Start Saving Data")) -> ()
            n754 = local write "Log Data"(w2117) -> ()
            "Write Header" <- TRUE ("Write Header")
          }
        }
        n755 = call <vilib>:"Add State(s) to Queue__jki_lib_state_machine.vi"("State(s) in (\"\")"=w2092) -> ("States Out"=w2091:string)  [unwired: 14 in]
        n756 = flat-sequence {
          tunnel: w2084 -> [w2116]
          tunnel: [w2116] -> w2086
          tunnel: w2076 -> [w2115]
          tunnel: [w2113] -> w2085
          frame #0 {
            n757 = Bundle By Name(cluster=w2115, "Filepath.Data File Paths.Data File Path"=path "") -> (w2113:T62)
          }
        }
        n758 = local write "Test Status"("Adding Final Headers...." ("Test Status")) -> ()
      }
    }
    n759 = case shown="True" "Debug Main" {
      tunnel: w533 -> [_ w550]
      tunnel: [w545 w547] -> w532
      tunnel: w534 -> [w545 w549]
      frame False {
      }
      frame True {
        n760 = Build Array (concatenate)(w549, w550) -> (w546:string[])
        "Test State" <- w546
        n761 = Array Size(array=w546) -> (size(s)=w548:i32)
        n762 = case shown="100" w548 {
          tunnel: [w551 w554] -> w547
          tunnel: w546 -> [w551 w555]
          frame 0, Default {
          }
          frame 100 {
            n763 = Delete From Array(array=w555, length=5, index=0) -> (array with subset deleted=w554:string[])  [unwired: 1 out]
          }
        }
        "Main State" <- w550
      }
    }
    "Main Loop" <- w531
  }
  n764 = case shown="\"IND560 SERIAL\"" w17 {
    tunnel: w18 -> [w2121 w2124 w2128 w2131]
    tunnel: [w2121 w2125 w2127 w2130] -> w10
    tunnel: w12 -> [_ w2123 _ _]
    tunnel: w3 -> [_ _ w2126 w2129]
    frame "False", Default {
    }
    frame "ZM301" {
      n765 = call-dynamic "Shutdown.vi"("error in"=w2124, "Modbus master in"=w2123) -> ("error out"=w2122:errorcluster)  [unwired: 9 in]
      n766 = call <vilib>:"Simple Error Handler.vi"("error in (no error)"=w2122) -> ("error out"=w2125:errorcluster)  [unwired: 1 in, 7 out]
    }
    frame "GSE 350" {
      n767 = call "GSE 350 Close.vi"("error in (no error)"=w2128, "VISA Refnum in"=w2126) -> ("error out"=w2127:errorcluster)  [unwired: 9 in]
    }
    frame "IND560 SERIAL" {
      n768 = call "IND560 Serial Close.vi"("error in (no error)"=w2131, "VISA Refnum in"=w2129) -> ("error out"=w2130:errorcluster)  [unwired: 9 in]
    }
  }
  n769 = Merge Errors(w10, w20, w24) -> (→"error out":errorcluster)
